vi "Lab Panel V3.0.vi"() -> ()   [LabVIEW 2013]
uses:
  <vilib>/Platform/TimedLoop/XDataNode/timing_clust.ctl
  <vilib>/Platform/TimedLoop/XDataNode/nitl_modes.ctl
  <vilib>/Platform/TimedLoop/XDataNode/wakeup.ctl
  <vilib>/platform/TimedLoop/XDataNode/XDataNode.xnode
  <vilib>/Platform/TimedLoop/XDataNode/XDNodeRunTimeDep.lvlib
panel:
  out "TEMP update":bool
  out "AI update":bool
  in  "stop":bool
  in  "Tab Control 2":T1(tab)
  out "LAB05-2 (SIG)":T2 {"PF" format="%.2f"; "AMPS" format="%.1f"}
  out "LAB05-1 (SIG)":T2 {"PF" format="%.2f"; "AMPS" format="%.1f"}
  out "LAB04-2 (SIG)":T2 {"PF" format="%.2f"; "AMPS" format="%.1f"}
  out "LAB04-1 (SIG)":T2 {"PF" format="%.2f"; "AMPS" format="%.1f"}
  out "LAB03-2 (SIG)":T2 {"PF" format="%.2f"; "AMPS" format="%.1f"}
  out "LAB03-1 (SIG)":T2 {"PF" format="%.2f"; "AMPS" format="%.1f"}
  out "LAB02-2 (SIG)":T2 {"PF" format="%.2f"; "AMPS" format="%.1f"}
  in  "LAB01-1RUN":bool
  in  "LAB05-1 (O/I)":bool
  in  "LAB05-2 (O/I)":bool
  in  "LAB04-1 (O/I)":bool
  in  "LAB04-2 (O/I)":bool
  in  "LAB02-1 (O/I)":bool
  in  "LAB02-2 (O/I)":bool
  in  "LAB01-2 (O/I)":bool
  in  "LAB01-1 (O/I)":bool
  in  "LAB03-1 (O/I)":bool
  in  "LAB05-2 RUN":bool
  in  "LAB05-1 RUN":bool
  in  "LAB04-2 RUN":bool
  in  "LAB04-1 RUN":bool
  in  "LAB03-2 RUN":bool
  in  "LAB03-1 RUN":bool
  in  "LAB02-2 RUN":bool
  in  "LAB02-1 RUN":bool
  in  "LAB01-2 RUN":bool
  in  "LAB05-2 SELECT":T3(radio)
  in  "LAB05-1 SELECT":T3(radio)
  in  "LAB04-2 SELECT":T3(radio)
  in  "LAB04-1 SELECT":T3(radio)
  in  "LAB03-2 SELECT":T3(radio)
  in  "LAB03-1 SELECT":T3(radio)
  in  "LAB02-2 SELECT":T3(radio)
  in  "LAB02-1 SELECT":T3(radio)
  in  "LAB01-2 SELECT":T3(radio)
  in  "LAB01-1 SELECT":T3(radio)
  in  "LAB03-2 (O/I)":bool
  out "LAB01-1 (SIG)":T2 {"PF" format="%.2f"; "AMPS" format="%.1f"}
  out "LAB01-2 (SIG)":T2 {"PF" format="%.2f"; "AMPS" format="%.1f"}
  out "LAB02-1 (SIG)":T2 {"PF" format="%.2f"; "AMPS" format="%.1f"}
  out "LAB05-2 (DISP)":T4 {"MINS" format="%.2g"}
  out "LAB05-1 (DISP)":T4 {"MINS" format="%.2g"}
  out "LAB04-2 (DISP)":T4 {"MINS" format="%.2g"}
  out "LAB04-1 (DISP)":T4 {"MINS" format="%.2g"}
  out "LAB03-2 (DISP)":T4 {"MINS" format="%.2g"}
  out "LAB03-1 (DISP)":T4 {"MINS" format="%.2g"}
  in  "LAB05-2 (SET)":T5
  in  "LAB05-1 (SET)":T5
  in  "LAB04-2 (SET)":T5
  in  "LAB04-1 (SET)":T5
  in  "LAB03-2 (SET)":T5
  in  "LAB03-1 (SET)":T5
  out "LAB02-2 (DISP)":T4 {"MINS" format="%.2g"}
  out "LAB02-1 (DISP)":T4 {"MINS" format="%.2g"}
  in  "LAB02-2 (SET)":T5
  in  "LAB02-1 (SET)":T5
  out "LAB05-2 (RESULT)":bool
  out "LAB05-1 (RESULT)":bool
  out "LAB04-2 (RESULT)":bool
  out "LAB04-1 (RESULT)":bool
  out "LAB03-2 (RESULT)":bool
  out "LAB03-1 (RESULT)":bool
  out "LAB02-2 (RESULT)":bool
  out "LAB02-1 (RESULT)":bool
  out "LAB01-2 (RESULT)":bool
  out "LAB01-1 (RESULT)":bool
  in  "LAB01-1 (SET)":T5
  in  "LAB01-2 (SET)":T5
  out "LAB01-1 (DISP)":T4 {"MINS" format="%.2g"}
  out "LAB01-2 (DISP)":T4 {"MINS" format="%.2f"}
  in  "Network Directory":path
  in  "JIG OFF TIME (S)":dbl=2.0 min=2.0 max=10.0 step=0.5 format="%.1g"
  in  "JIG ON TIME (S)":dbl=1.0 min=1.0 max=10.0 step=0.5 format="%.1g"
  out "LAB05-2 (FAIL)":cluster{"LO":dbl, "HI":dbl}
  out "LAB05-1 (FAIL)":cluster{"LO":dbl, "HI":dbl}
  out "LAB04-2 (FAIL)":cluster{"LO":dbl, "HI":dbl}
  out "LAB04-1 (FAIL)":cluster{"LO":dbl, "HI":dbl}
  out "LAB03-2 (FAIL)":cluster{"LO":dbl, "HI":dbl}
  out "LAB03-1 (FAIL)":cluster{"LO":dbl, "HI":dbl}
  out "LAB02-2 (FAIL)":cluster{"LO":dbl, "HI":dbl}
  out "LAB02-1 (FAIL)":cluster{"LO":dbl, "HI":dbl}
  out "LAB01-2 (FAIL)":cluster{"LO":dbl, "HI":dbl}
  out "LAB01-1 (FAIL)":cluster{"LO":dbl, "HI":dbl}
  out "LAB05-2 (TEMP START)":cluster{"TL":dbl, "TN":dbl}
  out "LAB04-2 (TEMP START)":cluster{"TL":dbl, "TN":dbl}
  out "LAB03-2 (TEMP START)":cluster{"TL":dbl, "TN":dbl}
  out "LAB02-2 (TEMP START)":cluster{"TL":dbl, "TN":dbl}
  out "LAB01-2 (TEMP START)":cluster{"TL":dbl, "TN":dbl}
  out "LAB05-1 (TEMP START)":cluster{"TL":dbl, "TN":dbl}
  out "LAB04-1 (TEMP START)":cluster{"TL":dbl, "TN":dbl}
  out "LAB03-1 (TEMP START)":cluster{"TL":dbl, "TN":dbl}
  out "LAB02-1 (TEMP START)":cluster{"TL":dbl, "TN":dbl}
  out "LAB01-1 (TEMP START)":cluster{"TL":dbl, "TN":dbl}
  out "LAB01-1 (JIG)":bool
  out "LAB01-2 (JIG)":bool
  out "LAB02-1 (JIG)":bool
  out "LAB02-2 (JIG)":bool
  out "LAB03-1 (JIG)":bool
  out "LAB03-2 (JIG)":bool
  out "LAB04-1 (JIG)":bool
  out "LAB04-2 (JIG)":bool
  out "LAB05-1 (JIG)":bool
  out "LAB05-2 (JIG)":bool
  out "LAB01 (CAL)":T6 {"2 (TN) cal" min=0.0 step=0.01 format="%.2f"; "2 (TL) cal" min=0.0 step=0.01 format="%.2f"; "2 (PF) cal" min=0.0 step=0.01 format="%.2f"; "2 (V) cal" min=0.0 step=0.01 format="%.2f"; "2 (A) cal" min=0.0 step=0.01 format="%.2f"; "1 (TN) cal" min=0.0 step=0.01 format="%.2f"; "1 (TL) cal" min=0.0 step=0.01 format="%.2f"; "1 (PF) cal" min=0.0 step=0.01 format="%.2f"; "1 (V) cal" min=0.0 step=0.01 format="%.2f"; "1  (A) cal" min=0.0 step=0.01 format="%.2f"}
  out "LAB03 (CAL)":T6 {"2 (TN) cal" min=0.0 step=0.01 format="%.2f"; "2 (TL) cal" min=0.0 step=0.01 format="%.2f"; "2 (PF) cal" min=0.0 step=0.01 format="%.2f"; "2 (V) cal" min=0.0 step=0.01 format="%.2f"; "2 (A) cal" min=0.0 step=0.01 format="%.2f"; "1 (TN) cal" min=0.0 step=0.01 format="%.2f"; "1 (TL) cal" min=0.0 step=0.01 format="%.2f"; "1 (PF) cal" min=0.0 step=0.01 format="%.2f"; "1 (V) cal" min=0.0 step=0.01 format="%.2f"; "1  (A) cal" min=0.0 step=0.01 format="%.2f"}
  out "LAB02 (CAL)":T7 {"2 (TN) cal" min=0.0 step=0.01 format="%.2f"; "2 (TL) cal" min=0.0 step=0.01 format="%.2f"; "2 (PF) cal" min=0.0 step=0.01 format="%.2f"; "2 (V) cal" min=0.0 step=0.01 format="%.2f"; "2 (A) cal" min=0.0 step=0.01 format="%.2f"; "1 (TN) cal" min=0.0 step=0.01 format="%.2f"; "1 (TL) cal" min=0.0 step=0.01 format="%.2f"; "1 (PF) cal" min=0.0 step=0.01 format="%.2f"; "1 (V) cal" min=0.0 step=0.01 format="%.2f"; "1 (A) cal" min=0.0 step=0.01 format="%.2f"}
  out "LAB05 (CAL)":T6 {"2 (TN) cal" min=0.0 step=0.01 format="%.2f"; "2 (TL) cal" min=0.0 step=0.01 format="%.2f"; "2 (PF) cal" min=0.0 step=0.01 format="%.2f"; "2 (V) cal" min=0.0 step=0.01 format="%.2f"; "2 (A) cal" min=0.0 step=0.01 format="%.2f"; "1 (TN) cal" min=0.0 step=0.01 format="%.2f"; "1 (TL) cal" min=0.0 step=0.01 format="%.2f"; "1 (PF) cal" min=0.0 step=0.01 format="%.2f"; "1 (V) cal" min=0.0 step=0.01 format="%.2f"; "1  (A) cal" min=0.0 step=0.01 format="%.2f"}
  out "LAB04 (CAL)":T6 {"2 (TN) cal" min=0.0 step=0.01 format="%.2f"; "2 (TL) cal" min=0.0 step=0.01 format="%.2f"; "2 (PF) cal" min=0.0 step=0.01 format="%.2f"; "2 (V) cal" min=0.0 step=0.01 format="%.2f"; "2 (A) cal" min=0.0 step=0.01 format="%.2f"; "1 (TN) cal" min=0.0 step=0.01 format="%.2f"; "1 (TL) cal" min=0.0 step=0.01 format="%.2f"; "1 (PF) cal" min=0.0 step=0.01 format="%.2f"; "1 (V) cal" min=0.0 step=0.01 format="%.2f"; "1  (A) cal" min=0.0 step=0.01 format="%.2f"}
  out "calibration file error out":errorcluster
  in  "CALIBRATE":bool
  in  "Tab Control":T8(tab)
  out "LAB01-2 (GRAPH)":dynamicdata(graph)
  out "LAB01-1 (GRAPH)":dynamicdata(graph)
  out "LAB02-2 (GRAPH)":dynamicdata(graph)
  out "LAB02-1 (GRAPH)":dynamicdata(graph)
  out "LAB03-2 (GRAPH)":dynamicdata(graph)
  out "LAB03-1 (GRAPH)":dynamicdata(graph)
  out "LAB04-2 (GRAPH)":dynamicdata(graph)
  out "LAB04-1 (GRAPH)":dynamicdata(graph)
  out "LAB05-2 (GRAPH)":dynamicdata(graph)
  out "LAB05-1 (GRAPH)":dynamicdata(graph)
  out "LAB05 TEMP":T9
  out "LAB04 TEMP":T9
  out "LAB02 TEMP":T9
  out "LAB01 TEMP":T9
  out "LAB03 TEMP":T9
  out "Analog Error Array":errorcluster[](array[cluster])
  out "AI loop time":dbl format="%.6g"
  out "loops":dbl
  in  "loop  delay(mS)":dbl
  out "on loops":dbl
  out "off loops":dbl
  out "jig cycle":dbl
  out "LAB01-1 (TDMS)":refnum<k34>
  out "data file error":errorcluster
  out "LAB02-1 (TDMS)":refnum<k34>
  out "LAB01-2 (TDMS)":refnum<k34>
  out "LAB02-2 (TDMS)":refnum<k34>
  out "LAB03-1 (TDMS)":refnum<k34>
  out "LAB03-2 (TDMS)":refnum<k34>
  out "LAB04-1 (TDMS)":refnum<k34>
  out "LAB04-2 (TDMS)":refnum<k34>
  out "LAB05-1 (TDMS)":refnum<k34>
  out "LAB05-2 (TDMS)":refnum<k34>
  # "LAB01"
  # "LAB02"
  # "LAB05"
  # "LAB03"
  # "LAB04"
  # "LAB01"
  # "LAB02"
  # "LAB03"
  # "LAB04"
  # "LAB05"
  # "JIG SET"
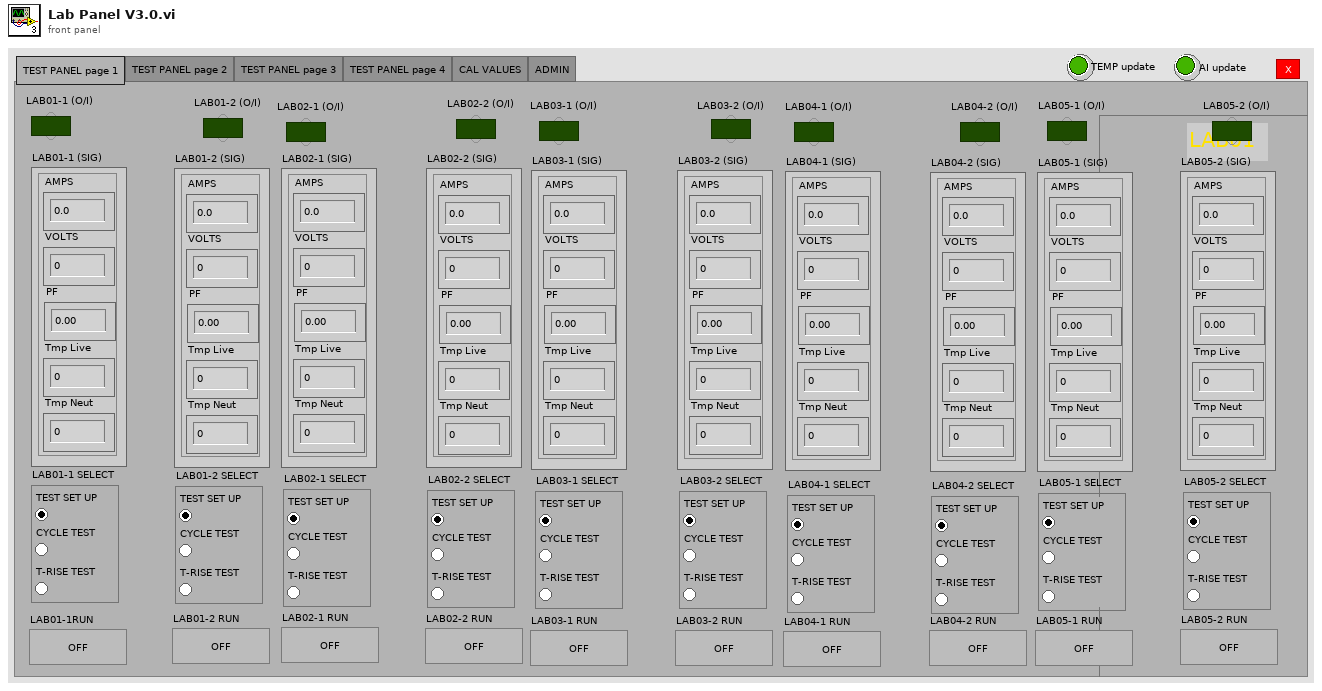
[diagram p1: front panel]
types:
  T1 = enum32{"TEST PANEL page 1", "TEST PANEL page 2", "TEST PANEL page 3", "TEST PANEL page 4", "CAL VALUES", "ADMIN"}
  T2 = cluster{"AMPS":dbl, "VOLTS":dbl, "PF":dbl, "Tmp Live":dbl, "Tmp Neut":dbl}
  T3 = enum32{"TEST SET UP", "CYCLE TEST", "T-RISE TEST"}
  T4 = cluster{"CYCLE":dbl, "MINS":dbl, "STATUS":string}
  T5 = cluster{"NAME":string, "DESCRIPTION":string, "CYCLES":dbl, "T-RISE mins":dbl, "T-RISE deg C":dbl}
  T6 = cluster{"1  (A) cal":dbl, "1 (V) cal":dbl, "1 (PF) cal":dbl, "1 (TL) cal":dbl, "1 (TN) cal":dbl, "2 (A) cal":dbl, "2 (V) cal":dbl, "2 (PF) cal":dbl, "2 (TL) cal":dbl, "2 (TN) cal":dbl}
  T7 = cluster{"1 (A) cal":dbl, "1 (V) cal":dbl, "1 (PF) cal":dbl, "1 (TL) cal":dbl, "1 (TN) cal":dbl, "2 (A) cal":dbl, "2 (V) cal":dbl, "2 (PF) cal":dbl, "2 (TL) cal":dbl, "2 (TN) cal":dbl}
  T8 = enum32{"LAB01", "LAB02", "LAB03", "LAB04", "LAB05", "TEMPERATURE", "ERROR"}
  T9 = cluster{"T1 Live":dbl, "T1 Neut":dbl, "T2 Live":dbl, "T2 Neut":dbl, "ID":dbl, "ER":dbl}
  T10 = enum8{"Enabled", "Disabled", "Disabled and Grayed Out"}
  T11 = typedef "XDNodeRunTimeDep.lvlib/timing_clust.ctl" = cluster{"Expected End [f-1]":u64, "Actual End [f-1]":u64, "Finished Late? [f-1]":bool, "Expected End [i-1]":u64, "Actual End [i-1]":u64, "Finished Late? [i-1]":bool, "Expected Start [i]":u64, "Actual Start [i]":u64, "Expected Start [f]":u64, "Actual Start [f]":u64, "Source Name":string, "Structure Name":string, "Period":i64, "Deadline":i64, "Offset":i64, "Start":i64, "Priority":i32, "Timeout":i32, "Mode":T12, "Wakeup Reason":T13, "Error":errorcluster, "Source Type":string, "Secondary Source Type":string, "Global End Time":u64, "Global Start Time":u64, "Frame Duration":u64, "Iteration Duration":u64, "Assigned CPU":i32, "I/O Scan Engine Mode":u32}
  T12 = typedef "XDNodeRunTimeDep.lvlib/nitl_modes.ctl" = enum32{"No Change", "Process missed periods, maintain original phase", "Discard missed periods, maintain original phase", "Process missed periods, ignore original phase", "Discard missed periods, ignore original phase"}
  T13 = typedef "XDNodeRunTimeDep.lvlib/wakeup.ctl" = enum32{"Normal", "Aborted", "Asynchronous wakeup", "Timing source error", "Timed loop error", "Timeout"}
  T14 = enum16{"open", "open or create", "create or replace", "create", "open (read-only)"}
  T15 = enum16{"open", "replace", "create", "open or create", "replace or create", "replace or create with confirmation"}
  T16 = cluster{"LAB01-1 (SET)":cluster{"NAME":string, "DESCRIPTION":string, "CYCLES":dbl, "T-RISE mins":dbl, "T-RISE deg C":dbl}, "LAB01-2 (SET)":cluster{"NAME":string, "DESCRIPTION":string, "CYCLES":dbl, "T-RISE mins":dbl, "T-RISE deg C":dbl}, "LAB02-1 (SET)":cluster{"NAME":string, "DESCRIPTION":string, "CYCLES":dbl, "T-RISE mins":dbl, "T-RISE deg C":dbl}, "LAB02-2 (SET)":cluster{"NAME":string, "DESCRIPTION":string, "CYCLES":dbl, "T-RISE mins":dbl, "T-RISE deg C":dbl}, "LAB03-1 (SET)":cluster{"NAME":string, "DESCRIPTION":string, "CYCLES":dbl, "T-RISE mins":dbl, "T-RISE deg C":dbl}, "LAB03-2 (SET)":cluster{"NAME":string, "DESCRIPTION":string, "CYCLES":dbl, "T-RISE mins":dbl, "T-RISE deg C":dbl}, "LAB04-1 (SET)":cluster{"NAME":string, "DESCRIPTION":string, "CYCLES":dbl, "T-RISE mins":dbl, "T-RISE deg C":dbl}, "LAB04-2 (SET)":cluster{"NAME":string, "DESCRIPTION":string, "CYCLES":dbl, "T-RISE mins":dbl, "T-RISE deg C":dbl}, "LAB05-1 (SET)":cluster{"NAME":string, "DESCRIPTION":string, "CYCLES":dbl, "T-RISE mins":dbl, "T-RISE deg C":dbl}, "LAB05-2 (SET)":cluster{"NAME":string, "DESCRIPTION":string, "CYCLES":dbl, "T-RISE mins":dbl, "T-RISE deg C":dbl}, "Network Directory":path}
  T17 = cluster{"T1":dbl, "T2":dbl, "T3":dbl, "T4":dbl, "ID":dbl, "ER":dbl}
  T18 = cluster{"LAB01-1 (A)":dbl, "LAB01-1 (V)":dbl, "LAB01-1 (PF)":dbl, "LAB01-2 (A)":dbl, "LAB01-2 (V)":dbl, "LAB01-2 (PF)":dbl}
  T19 = cluster{"LAB02-1 (A)":dbl, "LAB02-1 (V)":dbl, "LAB02-1 (PF)":dbl, "LAB02-2 (A)":dbl, "LAB02-2 (V)":dbl, "LAB02-2 (PF)":dbl}
  T20 = cluster{"LAB03-1 (A)":dbl, "LAB03-1 (V)":dbl, "LAB03-1 (PF)":dbl, "LAB03-2 (A)":dbl, "LAB03-2 (V)":dbl, "LAB03-2 (PF)":dbl}
  T21 = cluster{"LAB04-1 (A)":dbl, "LAB04-1 (V)":dbl, "LAB04-1 (PF)":dbl, "LAB04-2 (A)":dbl, "LAB04-2 (V)":dbl, "LAB04-2 (PF)":dbl}
  T22 = cluster{"LAB05-1 (A)":dbl, "LAB05-1 (V)":dbl, "LAB05-1 (PF)":dbl, "LAB05-2 (A)":dbl, "LAB05-2 (V)":dbl, "LAB05-2 (PF)":dbl}
  T23 = cluster{"LAB01-1 (FAIL)":cluster{"LO":dbl, "HI":dbl}, "LAB01-1 (SIG)":cluster{"AMPS":dbl, "VOLTS":dbl, "PF":dbl, "Tmp Live":dbl, "Tmp Neut":dbl}, "LAB01-1 (TEMP START)":cluster{"TL":dbl, "TN":dbl}, "LAB01-1 (DISP)":cluster{"CYCLE":dbl, "MINS":dbl, "STATUS":string}, "LAB01-1 (SET)":cluster{"NAME":string, "DESCRIPTION":string, "CYCLES":dbl, "T-RISE mins":dbl, "T-RISE deg C":dbl}, "LAB01-1 (TDMS)":refnum<k34>}
  T24 = cluster{"LAB01-2 (FAIL)":cluster{"LO":dbl, "HI":dbl}, "LAB01-2 (SIG)":cluster{"AMPS":dbl, "VOLTS":dbl, "PF":dbl, "Tmp Live":dbl, "Tmp Neut":dbl}, "LAB01-2 (TEMP START)":cluster{"TL":dbl, "TN":dbl}, "LAB01-2 (DISP)":cluster{"CYCLE":dbl, "MINS":dbl, "STATUS":string}, "LAB01-2 (SET)":cluster{"NAME":string, "DESCRIPTION":string, "CYCLES":dbl, "T-RISE mins":dbl, "T-RISE deg C":dbl}, "LAB01-2 (TDMS)":refnum<k34>}
  T25 = cluster{"LAB02-1 (FAIL)":cluster{"LO":dbl, "HI":dbl}, "LAB02-1 (SIG)":cluster{"AMPS":dbl, "VOLTS":dbl, "PF":dbl, "Tmp Live":dbl, "Tmp Neut":dbl}, "LAB02-1 (TEMP START)":cluster{"TL":dbl, "TN":dbl}, "LAB02-1 (DISP)":cluster{"CYCLE":dbl, "MINS":dbl, "STATUS":string}, "LAB02-1 (SET)":cluster{"NAME":string, "DESCRIPTION":string, "CYCLES":dbl, "T-RISE mins":dbl, "T-RISE deg C":dbl}, "LAB02-1 (TDMS)":refnum<k34>}
  T26 = cluster{"LAB02-2 (FAIL)":cluster{"LO":dbl, "HI":dbl}, "LAB02-2 (SIG)":cluster{"AMPS":dbl, "VOLTS":dbl, "PF":dbl, "Tmp Live":dbl, "Tmp Neut":dbl}, "LAB02-2 (TEMP START)":cluster{"TL":dbl, "TN":dbl}, "LAB02-2 (DISP)":cluster{"CYCLE":dbl, "MINS":dbl, "STATUS":string}, "LAB02-2 (SET)":cluster{"NAME":string, "DESCRIPTION":string, "CYCLES":dbl, "T-RISE mins":dbl, "T-RISE deg C":dbl}, "LAB02-2 (TDMS)":refnum<k34>}
  T27 = cluster{"LAB03-1 (FAIL)":cluster{"LO":dbl, "HI":dbl}, "LAB03-1 (SIG)":cluster{"AMPS":dbl, "VOLTS":dbl, "PF":dbl, "Tmp Live":dbl, "Tmp Neut":dbl}, "LAB03-1 (TEMP START)":cluster{"TL":dbl, "TN":dbl}, "LAB03-1 (DISP)":cluster{"CYCLE":dbl, "MINS":dbl, "STATUS":string}, "LAB03-1 (SET)":cluster{"NAME":string, "DESCRIPTION":string, "CYCLES":dbl, "T-RISE mins":dbl, "T-RISE deg C":dbl}, "LAB03-1 (TDMS)":refnum<k34>}
  T28 = cluster{"LAB03-2 (FAIL)":cluster{"LO":dbl, "HI":dbl}, "LAB03-2 (SIG)":cluster{"AMPS":dbl, "VOLTS":dbl, "PF":dbl, "Tmp Live":dbl, "Tmp Neut":dbl}, "LAB03-2 (TEMP START)":cluster{"TL":dbl, "TN":dbl}, "LAB03-2 (DISP)":cluster{"CYCLE":dbl, "MINS":dbl, "STATUS":string}, "LAB03-2 (SET)":cluster{"NAME":string, "DESCRIPTION":string, "CYCLES":dbl, "T-RISE mins":dbl, "T-RISE deg C":dbl}, "LAB03-2 (TDMS)":refnum<k34>}
  T29 = cluster{"LAB04-1 (FAIL)":cluster{"LO":dbl, "HI":dbl}, "LAB04-1 (SIG)":cluster{"AMPS":dbl, "VOLTS":dbl, "PF":dbl, "Tmp Live":dbl, "Tmp Neut":dbl}, "LAB04-1 (TEMP START)":cluster{"TL":dbl, "TN":dbl}, "LAB04-1 (DISP)":cluster{"CYCLE":dbl, "MINS":dbl, "STATUS":string}, "LAB04-1 (SET)":cluster{"NAME":string, "DESCRIPTION":string, "CYCLES":dbl, "T-RISE mins":dbl, "T-RISE deg C":dbl}, "LAB04-1 (TDMS)":refnum<k34>}
  T30 = cluster{"LAB04-2 (FAIL)":cluster{"LO":dbl, "HI":dbl}, "LAB04-2 (SIG)":cluster{"AMPS":dbl, "VOLTS":dbl, "PF":dbl, "Tmp Live":dbl, "Tmp Neut":dbl}, "LAB04-2 (TEMP START)":cluster{"TL":dbl, "TN":dbl}, "LAB04-2 (DISP)":cluster{"CYCLE":dbl, "MINS":dbl, "STATUS":string}, "LAB04-2 (SET)":cluster{"NAME":string, "DESCRIPTION":string, "CYCLES":dbl, "T-RISE mins":dbl, "T-RISE deg C":dbl}, "LAB04-2 (TDMS)":refnum<k34>}
  T31 = cluster{"LAB05-1 (FAIL)":cluster{"LO":dbl, "HI":dbl}, "LAB05-1 (SIG)":cluster{"AMPS":dbl, "VOLTS":dbl, "PF":dbl, "Tmp Live":dbl, "Tmp Neut":dbl}, "LAB05-1 (TEMP START)":cluster{"TL":dbl, "TN":dbl}, "LAB05-1 (DISP)":cluster{"CYCLE":dbl, "MINS":dbl, "STATUS":string}, "LAB05-1 (SET)":cluster{"NAME":string, "DESCRIPTION":string, "CYCLES":dbl, "T-RISE mins":dbl, "T-RISE deg C":dbl}, "LAB05-1 (TDMS)":refnum<k34>}
  T32 = cluster{"LAB05-2 (FAIL)":cluster{"LO":dbl, "HI":dbl}, "LAB05-2 (SIG)":cluster{"AMPS":dbl, "VOLTS":dbl, "PF":dbl, "Tmp Live":dbl, "Tmp Neut":dbl}, "LAB05-2 (TEMP START)":cluster{"TL":dbl, "TN":dbl}, "LAB05-2 (DISP)":cluster{"CYCLE":dbl, "MINS":dbl, "STATUS":string}, "LAB05-2 (SET)":cluster{"NAME":string, "DESCRIPTION":string, "CYCLES":dbl, "T-RISE mins":dbl, "T-RISE deg C":dbl}, "LAB05-2 (TDMS)":refnum<k34>}
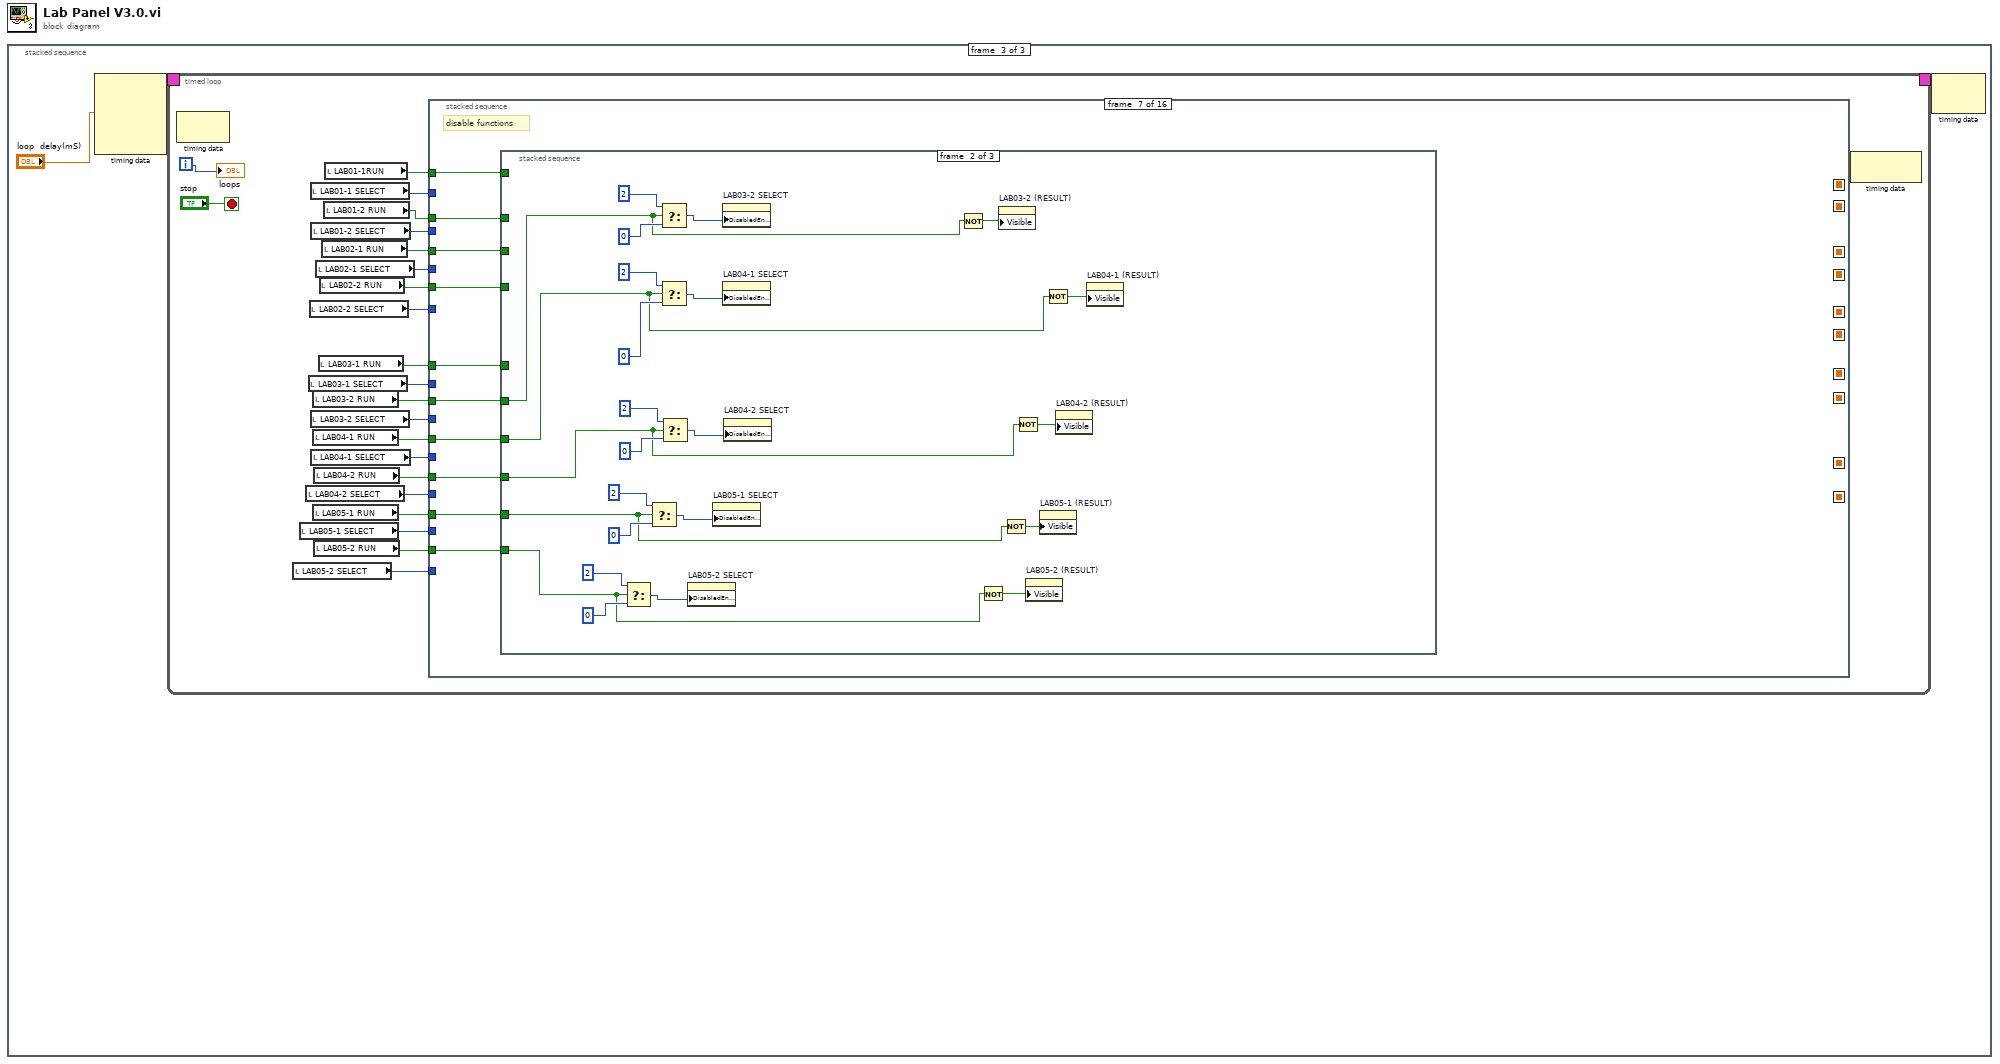
[diagram p0: block diagram]
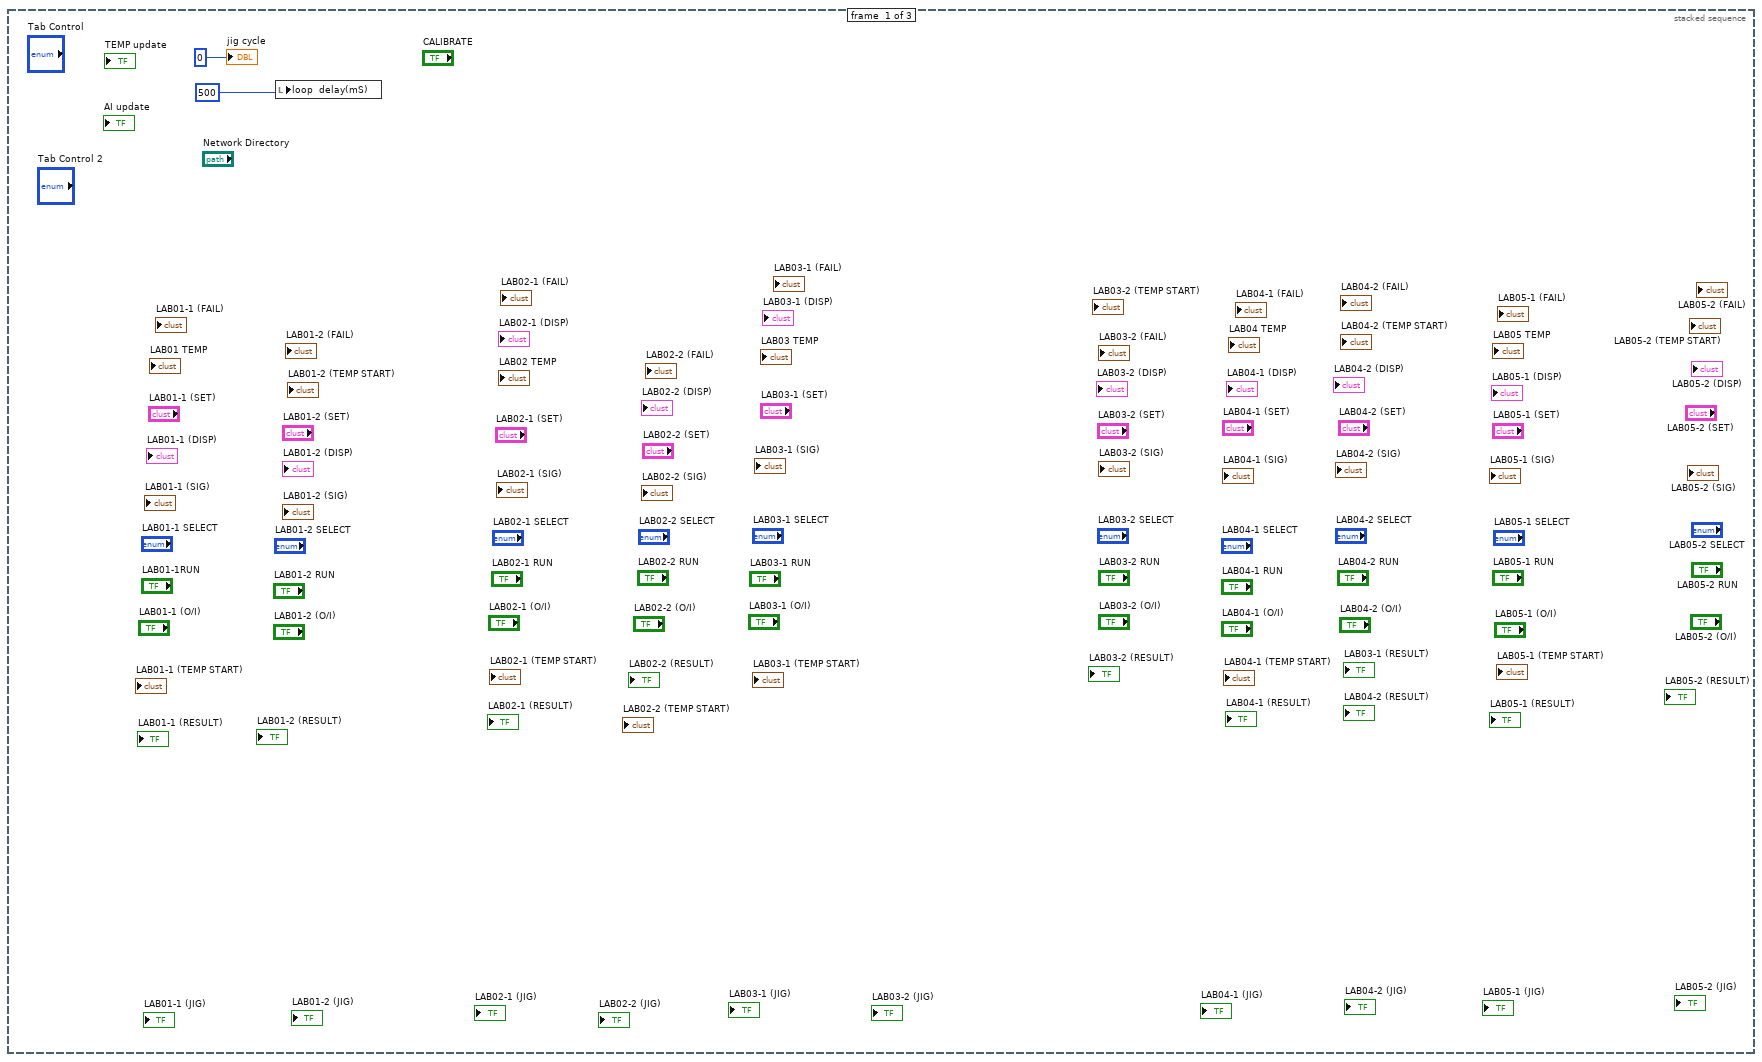
[diagram p2: hidden frame]
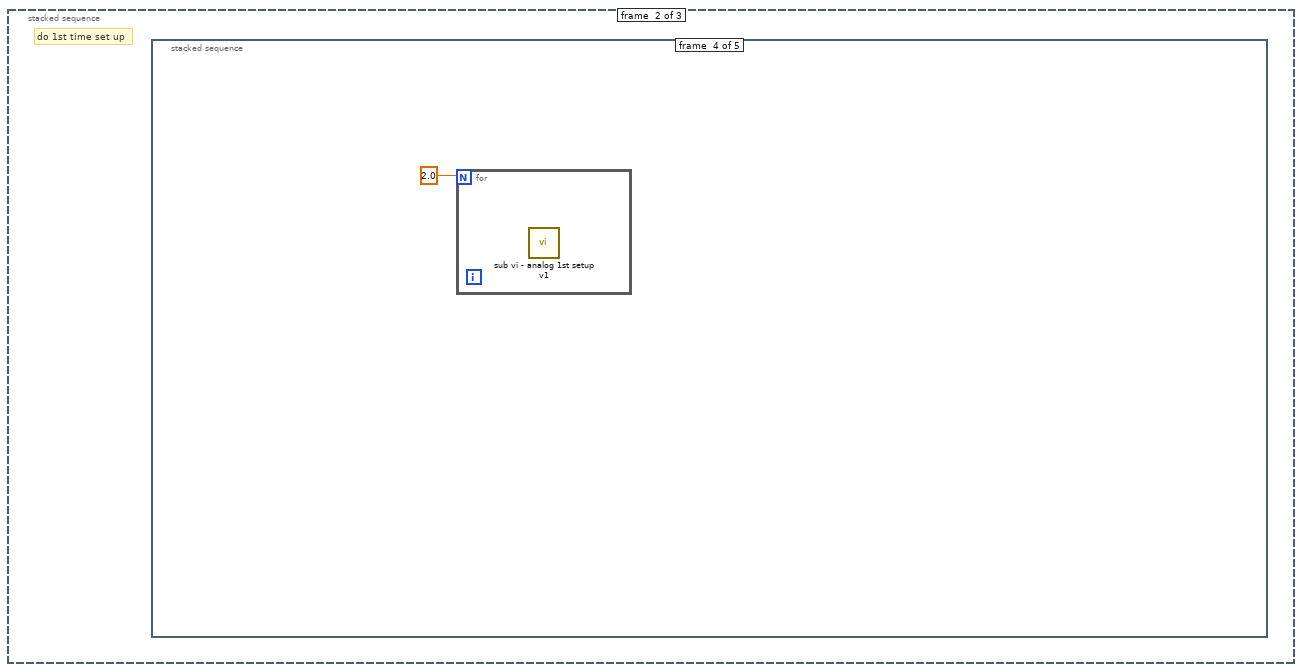
[diagram p3: hidden frame]
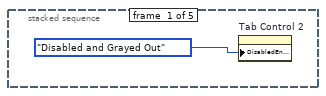
[diagram p4: hidden frame]
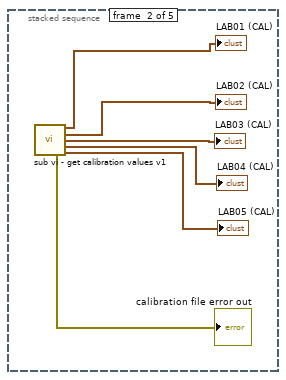
[diagram p5: hidden frame]
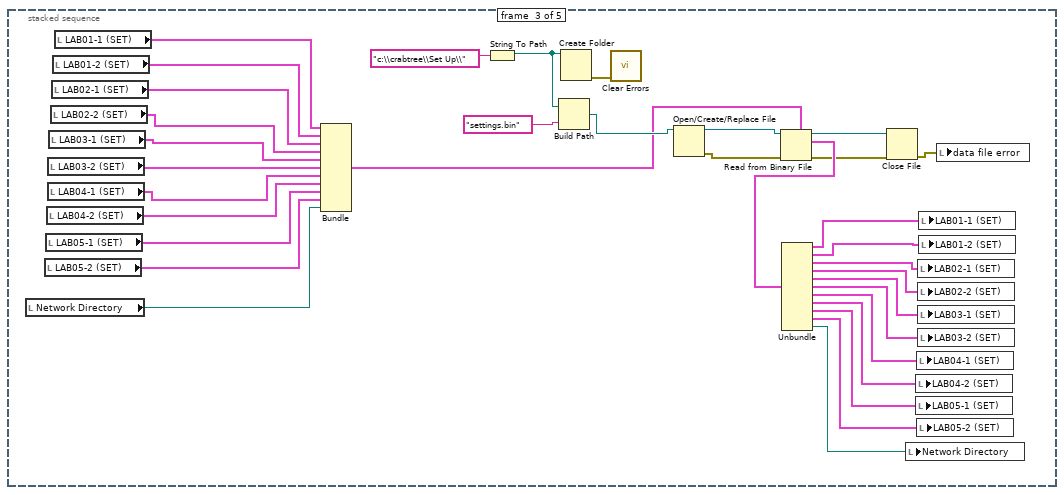
[diagram p6: hidden frame]
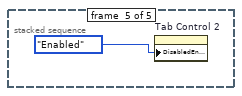
[diagram p7: hidden frame]
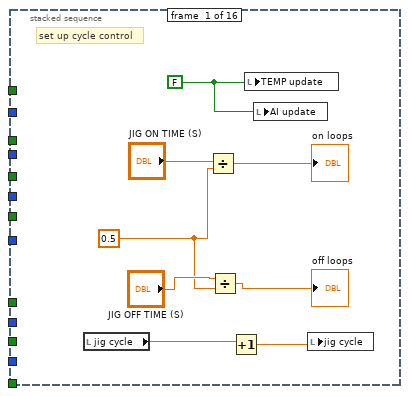
[diagram p8: hidden frame]
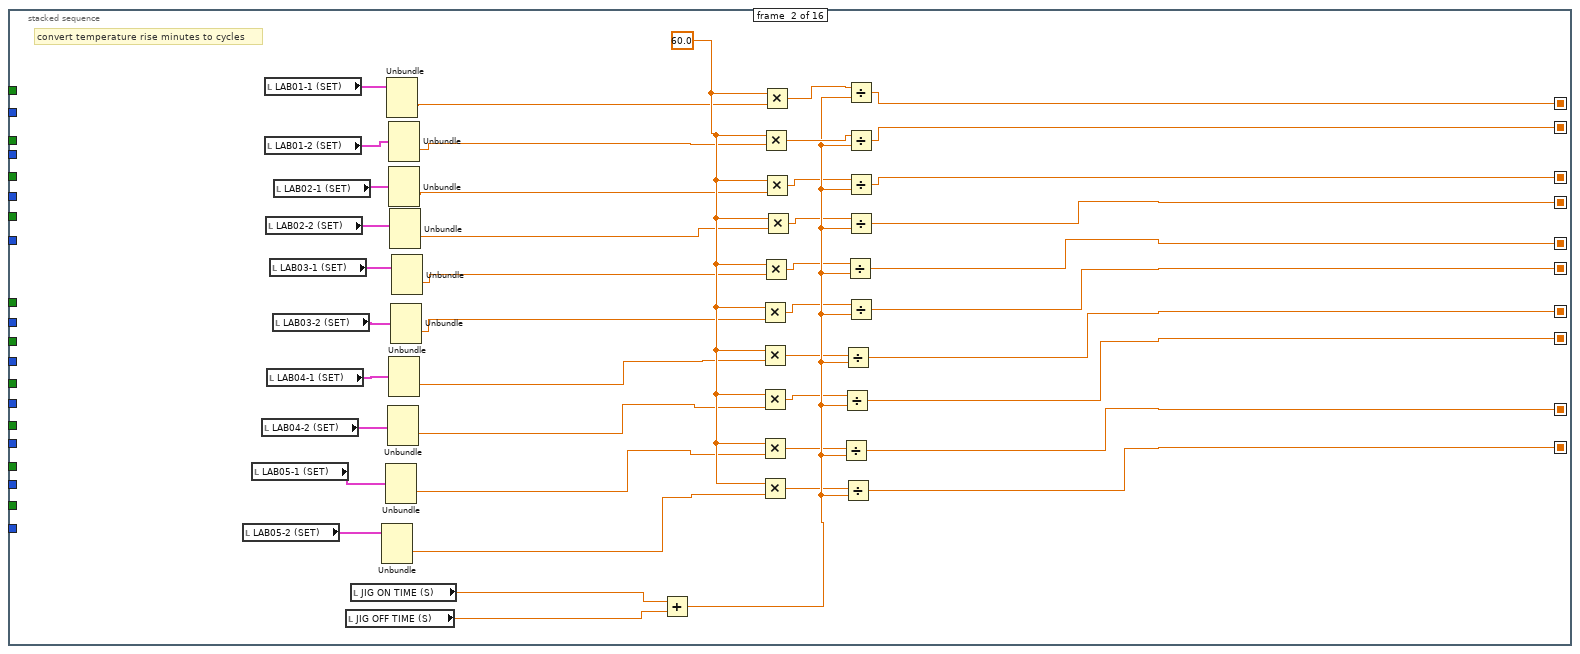
[diagram p9: hidden frame]
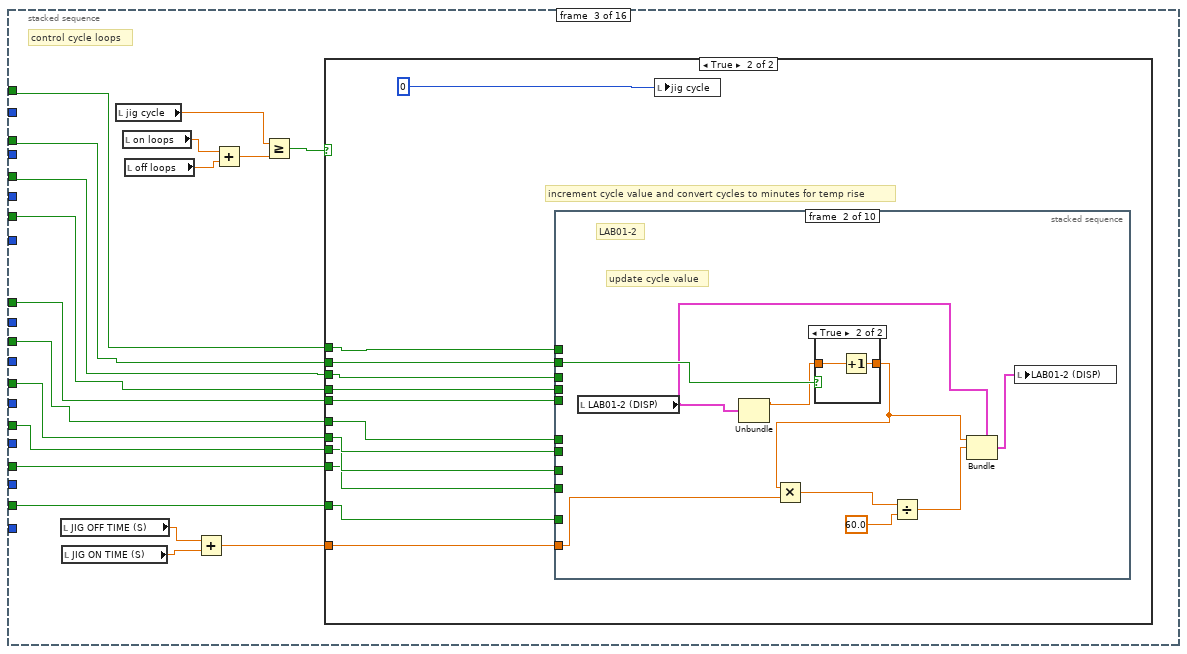
[diagram p10: hidden frame]
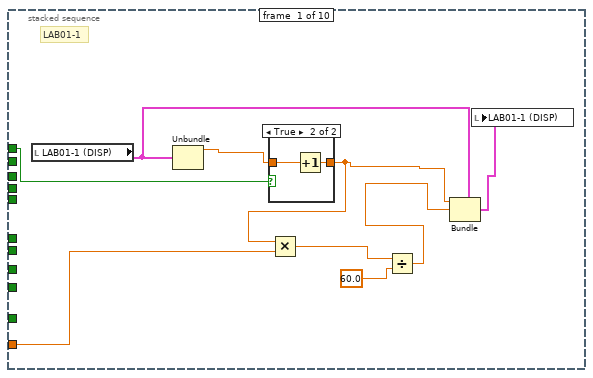
[diagram p12: hidden frame]
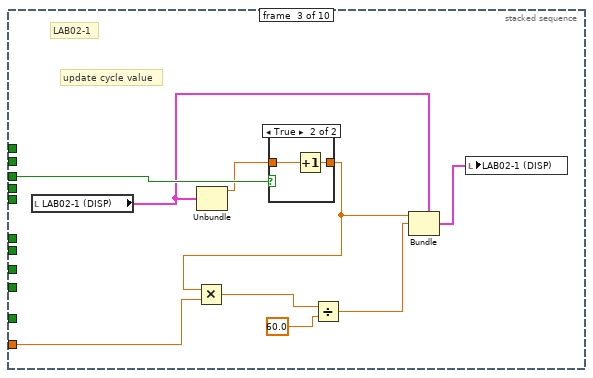
[diagram p15: hidden frame]
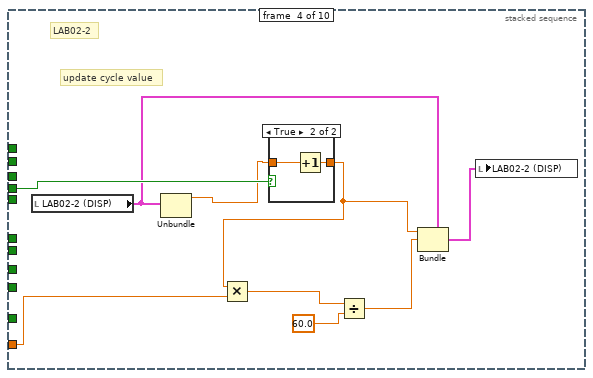
[diagram p17: hidden frame]
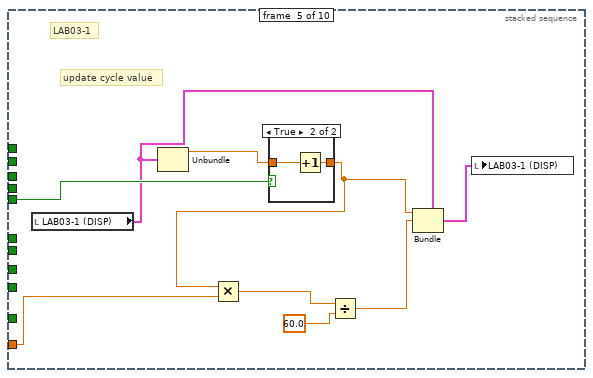
[diagram p19: hidden frame]
diagram:
  n1 = stacked-sequence {
    frame #0 {
      n2 = local write "loop  delay(mS)"(500) -> ()
      "jig cycle" <- 0
    }
    frame #1 {
      # "do 1st time set up"
      n3 = stacked-sequence {
        frame #0 {
          n4 = property on="Tab Control 2" class="TabCtl (strict)"("DisabledEnum"=T10."Disabled and Grayed Out" ("Disabled")) -> ()  [unwired: 2 in, 2 out]
        }
        frame #1 {
          n5 = call "sub vi - get calibration values v1.vi"() -> ("LAB01 (CAL)"=→"LAB01 (CAL)":T6, "LAB02 (CAL)"=→"LAB02 (CAL)":T7, "LAB03 (CAL)"=→"LAB03 (CAL)":T6, "LAB04 (CAL)"=→"LAB04 (CAL)":T6, "calibration file error out"=→"calibration file error out":errorcluster, "LAB05 (CAL)"=→"LAB05 (CAL)":T6)  [unwired: 10 in]
        }
        frame #2 {
          n6 = local read "Network Directory"() -> (w39:path)
          n7 = local read "LAB05-2 (SET)"() -> (w40:T5)
          n8 = local read "LAB05-1 (SET)"() -> (w41:T5)
          n9 = local read "LAB04-2 (SET)"() -> (w42:T5)
          n10 = local read "LAB03-2 (SET)"() -> (w38:T5)
          n11 = local read "LAB04-1 (SET)"() -> (w43:T5)
          n12 = local read "LAB03-1 (SET)"() -> (w37:T5)
          n13 = local read "LAB02-2 (SET)"() -> (w36:T5)
          n14 = local read "LAB02-1 (SET)"() -> (w35:T5)
          n15 = local read "LAB01-2 (SET)"() -> (w34:T5)
          n16 = local read "LAB01-1 (SET)"() -> (w33:T5)
          n17 = Bundle("LAB01-1 (SET)"=w33, "LAB01-2 (SET)"=w34, "LAB02-1 (SET)"=w35, "LAB02-2 (SET)"=w36, "LAB03-1 (SET)"=w37, "LAB03-2 (SET)"=w38, "LAB04-1 (SET)"=w43, "LAB04-2 (SET)"=w42, "LAB05-1 (SET)"=w41, "LAB05-2 (SET)"=w40, "Network Directory"=w39) -> (w26:T16)  [unwired: 1 in]
          n18 = String To Path(string="c:\\crabtree\\Set Up\\") -> (path=w30:path)
          n19 = Build Path(base path=w30, name or relative path="settings.bin") -> (appended path=w28:path)
          n20 = Create Folder(path (use dialog)=w30) -> (error out=w32:errorcluster)  [unwired: 2 in, 2 out]
          n21 = call <vilib>:"Clear Errors.vi"("error in (no error)"=w32) -> ()  [unwired: 6 in, 1 out]
          n22 = Open/Create/Replace File(file path (use dialog)=w28) -> (refnum out=w25:refnum<file>, error out=w27:errorcluster)  [unwired: 5 in, 1 out]
          n23 = Read from Binary File(5:w26, 8:w27, 11:w25) -> (0:w22:errorcluster, 2:w24:T16, 3:w23:refnum<file>)  [unwired: 3 in, 1 out]
          n24 = Unbundle(w24) -> ("LAB01-1 (SET)"=w20:T5, "LAB01-2 (SET)"=w19:T5, "LAB02-1 (SET)"=w18:T5, "LAB02-2 (SET)"=w17:T5, "LAB03-1 (SET)"=w16:T5, "LAB03-2 (SET)"=w15:T5, "LAB04-1 (SET)"=w14:T5, "LAB04-2 (SET)"=w13:T5, "LAB05-1 (SET)"=w12:T5, "LAB05-2 (SET)"=w11:T5, "Network Directory"=w10:path)
          n25 = Close File(refnum=w23, error in=w22) -> (error out=w21:errorcluster)  [unwired: 1 out]
          n26 = local write "Network Directory"(w10) -> ()
          n27 = local write "LAB04-2 (SET)"(w13) -> ()
          n28 = local write "LAB05-1 (SET)"(w12) -> ()
          n29 = local write "LAB04-1 (SET)"(w14) -> ()
          n30 = local write "LAB05-2 (SET)"(w11) -> ()
          n31 = local write "LAB02-1 (SET)"(w18) -> ()
          n32 = local write "LAB02-2 (SET)"(w17) -> ()
          n33 = local write "LAB03-1 (SET)"(w16) -> ()
          n34 = local write "LAB03-2 (SET)"(w15) -> ()
          n35 = local write "LAB01-1 (SET)"(w20) -> ()
          n36 = local write "LAB01-2 (SET)"(w19) -> ()
          n37 = local write "data file error"(w21) -> ()
        }
        frame #3 {
          n38 = for {
            N: 2.0 -> [_]
            n39 = call "sub vi - analog 1st setup v1.vi"() -> ()  [unwired: 11 in, 5 out]
          }
        }
        frame #4 {
          n40 = property on="Tab Control 2" class="TabCtl (strict)"("DisabledEnum"=T10."Enabled" ("Disabled")) -> ()  [unwired: 2 in, 2 out]
        }
      }
    }
    frame #2 {
      n41 = node-c288("loop  delay(mS)") -> (w48:T11)  [unwired: 3 in]
      n42 = timed-loop {
        timing: w48 -> [_]
        timing-out: [_] -> w47
        i -> [w70]
        stop <- "stop" stop-if-true
        n43 = node-c288() -> ()  [unwired: 1 in, 1 out]
        n44 = local read "LAB05-2 SELECT"() -> (w49:T3)
        n45 = local read "LAB05-1 SELECT"() -> (w50:T3)
        n46 = local read "LAB04-2 SELECT"() -> (w51:T3)
        n47 = local read "LAB03-1 SELECT"() -> (w54:T3)
        n48 = local read "LAB02-2 SELECT"() -> (w55:T3)
        n49 = local read "LAB01-1 SELECT"() -> (w58:T3)
        n50 = local read "LAB03-2 SELECT"() -> (w53:T3)
        n51 = local read "LAB01-2 SELECT"() -> (w57:T3)
        n52 = local read "LAB04-1 SELECT"() -> (w52:T3)
        n53 = local read "LAB03-2 RUN"() -> (w63:bool)
        n54 = local read "LAB04-1 RUN"() -> (w62:bool)
        n55 = local read "LAB05-1 RUN"() -> (w60:bool)
        n56 = local read "LAB04-2 RUN"() -> (w61:bool)
        n57 = local read "LAB05-2 RUN"() -> (w59:bool)
        n58 = local read "LAB02-1 SELECT"() -> (w56:T3)
        n59 = local read "LAB03-1 RUN"() -> (w64:bool)
        n60 = local read "LAB02-2 RUN"() -> (w65:bool)
        n61 = local read "LAB02-1 RUN"() -> (w66:bool)
        n62 = local read "LAB01-2 RUN"() -> (w67:bool)
        n63 = local read "LAB01-1RUN"() -> (w68:bool)
        n64 = stacked-sequence {
          seq-local: [_ w122 _ _ _ _ _ _ _ _ _ _ _ _ _ _] -> [_ _ _ _ _ w1501 _ _ _ _ _ _ _ _ _ _]
          seq-local: [_ w121 _ _ _ _ _ _ _ _ _ _ _ _ _ _] -> [_ _ _ _ _ _ _ _ _ _ _ _ _ _ _ _]
          seq-local: [_ w108 _ _ _ _ _ _ _ _ _ _ _ _ _ _] -> [_ _ _ _ _ _ _ _ _ _ _ _ _ _ _ _]
          seq-local: [_ w107 _ _ _ _ _ _ _ _ _ _ _ _ _ _] -> [_ _ _ _ _ _ _ _ _ _ _ _ _ _ _ _]
          seq-local: [_ w106 _ _ _ _ _ _ _ _ _ _ _ _ _ _] -> [_ _ _ _ _ _ _ _ _ _ _ _ _ _ _ _]
          seq-local: [_ w105 _ _ _ _ _ _ _ _ _ _ _ _ _ _] -> [_ _ _ _ _ _ _ _ _ _ _ _ _ _ _ _]
          seq-local: [_ w104 _ _ _ _ _ _ _ _ _ _ _ _ _ _] -> [_ _ _ _ _ _ _ _ _ _ _ _ _ _ _ _]
          seq-local: [_ w103 _ _ _ _ _ _ _ _ _ _ _ _ _ _] -> [_ _ _ _ _ _ _ _ _ _ _ _ _ _ _ _]
          seq-local: [_ w102 _ _ _ _ _ _ _ _ _ _ _ _ _ _] -> [_ _ _ _ _ _ _ _ _ _ _ _ _ _ _ _]
          seq-local: [_ w101 _ _ _ _ _ _ _ _ _ _ _ _ _ _] -> [_ _ _ _ _ _ _ _ _ _ _ _ _ _ _ _]
          tunnel: w68 -> [_ _ w138 w294 w1101 w1512 w1822 w1903 _ _ _ _ w2407 w2895 _ _]
          tunnel: w67 -> [_ _ w137 w292 w1100 w1511 w1821 w1904 _ _ _ _ w2406 w2893 _ _]
          tunnel: w66 -> [_ _ w136 w290 w1099 w1510 w1820 w1902 _ _ _ _ w2405 w2891 _ _]
          tunnel: w65 -> [_ _ w135 w288 w1098 w1509 w1819 w1901 _ _ _ _ w2404 w2889 _ _]
          tunnel: w64 -> [_ _ w134 w286 w1097 w1508 w1818 w1900 _ _ _ _ w2403 w2887 _ _]
          tunnel: w63 -> [_ _ w133 w284 w1096 w1507 w1817 w1899 _ _ _ _ w2402 w2885 _ _]
          tunnel: w62 -> [_ _ w132 w282 w1095 w1506 w1816 w1898 _ _ _ _ w2401 w2883 _ _]
          tunnel: w61 -> [_ _ w131 w280 w1094 w1505 w1815 w1897 _ _ _ _ w2400 w2881 _ _]
          tunnel: w60 -> [_ _ w130 w278 w1093 w1504 w1814 w1896 _ _ _ _ w2399 w2879 _ _]
          tunnel: w59 -> [_ _ w129 w276 w1092 w1503 w1813 w1895 _ _ _ _ w2398 w2877 _ _]
          tunnel: w58 -> [_ _ _ w293 w1091 w1502 _ _ _ _ _ _ _ w2897 _ _]
          tunnel: w57 -> [_ _ _ w291 w1090 w1500 _ _ _ _ _ _ _ w2892 _ _]
          tunnel: w56 -> [_ _ _ w289 w1089 w1499 _ _ _ _ _ _ _ w2890 _ _]
          tunnel: w55 -> [_ _ _ w287 w1088 w1498 _ _ _ _ _ _ _ w2888 _ _]
          tunnel: w54 -> [_ _ _ w285 w1087 w1497 _ _ _ _ _ _ _ w2886 _ _]
          tunnel: w53 -> [_ _ _ w283 w1086 w1496 _ _ _ _ _ _ _ w2884 _ _]
          tunnel: w52 -> [_ _ _ w281 w1085 w1495 _ _ _ _ _ _ _ w2882 _ _]
          tunnel: w51 -> [_ _ _ w279 w1084 w1494 _ _ _ _ _ _ _ w2880 _ _]
          tunnel: w50 -> [_ _ _ w277 w1083 w1493 _ _ _ _ _ _ _ w2878 _ _]
          tunnel: w49 -> [_ _ _ w275 w1082 w1492 _ _ _ _ _ _ _ w2876 _ _]
          frame #0 {
            w73 = FALSE
            w78 = 0.5
            # "set up cycle control"
            n65 = local read "jig cycle"() -> (w77:dbl)
            n66 = Divide(x="JIG ON TIME (S)", y=w78) -> (x/y=→"on loops":dbl)
            n67 = Divide(x="JIG OFF TIME (S)", y=w78) -> (x/y=→"off loops":dbl)
            n68 = Increment(x=w77) -> (x+1=w76:dbl)
            n69 = local write "TEMP update"(w73) -> ()
            n70 = local write "AI update"(w73) -> ()
            n71 = local write "jig cycle"(w76) -> ()
          }
          frame #1 {
            w118 = 60.0
            # "convert temperature rise minutes to cycles"
            n72 = local read "LAB05-2 (SET)"() -> (w82:T5)
            n73 = local read "LAB05-1 (SET)"() -> (w84:T5)
            n74 = local read "LAB04-2 (SET)"() -> (w86:T5)
            n75 = local read "LAB01-1 (SET)"() -> (w100:T5)
            n76 = local read "LAB01-2 (SET)"() -> (w98:T5)
            n77 = local read "LAB02-2 (SET)"() -> (w94:T5)
            n78 = local read "LAB04-1 (SET)"() -> (w88:T5)
            n79 = local read "LAB03-1 (SET)"() -> (w92:T5)
            n80 = local read "LAB03-2 (SET)"() -> (w90:T5)
            n81 = local read "LAB02-1 (SET)"() -> (w96:T5)
            n82 = local read "JIG OFF TIME (S)"() -> (w123:dbl)
            n83 = local read "JIG ON TIME (S)"() -> (w124:dbl)
            n84 = Unbundle(w82) -> ("T-RISE mins"=w81:dbl)  [unwired: 4 out]
            n85 = Unbundle(w84) -> ("T-RISE mins"=w83:dbl)  [unwired: 4 out]
            n86 = Unbundle(w100) -> ("T-RISE mins"=w99:dbl)  [unwired: 4 out]
            n87 = Unbundle(w86) -> ("T-RISE mins"=w85:dbl)  [unwired: 4 out]
            n88 = Unbundle(w98) -> ("T-RISE mins"=w97:dbl)  [unwired: 4 out]
            n89 = Unbundle(w96) -> ("T-RISE mins"=w95:dbl)  [unwired: 4 out]
            n90 = Unbundle(w88) -> ("T-RISE mins"=w87:dbl)  [unwired: 4 out]
            n91 = Unbundle(w94) -> ("T-RISE mins"=w93:dbl)  [unwired: 4 out]
            n92 = Unbundle(w90) -> ("T-RISE mins"=w89:dbl)  [unwired: 4 out]
            n93 = Unbundle(w92) -> ("T-RISE mins"=w91:dbl)  [unwired: 4 out]
            n94 = Add(x=w124, y=w123) -> (x+y=w117:dbl)
            n95 = Multiply(x=w118, y=w89) -> (x*y=w113:dbl)
            n96 = Multiply(x=w118, y=w87) -> (x*y=w112:dbl)
            n97 = Multiply(x=w118, y=w85) -> (x*y=w111:dbl)
            n98 = Multiply(x=w118, y=w83) -> (x*y=w110:dbl)
            n99 = Multiply(x=w118, y=w81) -> (x*y=w109:dbl)
            n100 = Multiply(x=w118, y=w97) -> (x*y=w119:dbl)
            n101 = Multiply(x=w118, y=w91) -> (x*y=w114:dbl)
            n102 = Multiply(x=w118, y=w99) -> (x*y=w120:dbl)
            n103 = Multiply(x=w118, y=w95) -> (x*y=w116:dbl)
            n104 = Multiply(x=w118, y=w93) -> (x*y=w115:dbl)
            n105 = Divide(x=w110, y=w117) -> (x/y=w102:dbl)
            n106 = Divide(x=w111, y=w117) -> (x/y=w103:dbl)
            n107 = Divide(x=w112, y=w117) -> (x/y=w104:dbl)
            n108 = Divide(x=w109, y=w117) -> (x/y=w101:dbl)
            n109 = Divide(x=w114, y=w117) -> (x/y=w106:dbl)
            n110 = Divide(x=w120, y=w117) -> (x/y=w122:dbl)
            n111 = Divide(x=w119, y=w117) -> (x/y=w121:dbl)
            n112 = Divide(x=w116, y=w117) -> (x/y=w108:dbl)
            n113 = Divide(x=w115, y=w117) -> (x/y=w107:dbl)
            n114 = Divide(x=w113, y=w117) -> (x/y=w105:dbl)
          }
          frame #2 {
            # "control cycle loops"
            n115 = local read "JIG OFF TIME (S)"() -> (w127:dbl)
            n116 = local read "JIG ON TIME (S)"() -> (w126:dbl)
            n117 = local read "jig cycle"() -> (w140:dbl)
            n118 = local read "on loops"() -> (w142:dbl)
            n119 = local read "off loops"() -> (w141:dbl)
            n120 = Add(x=w127, y=w126) -> (x+y=w125:dbl)
            n121 = Add(x=w142, y=w141) -> (x+y=w128:dbl)
            n122 = Greater Or Equal?(x=w140, y=w128) -> (x >= y?=w139:bool)
            n123 = case shown="True" w139 {
              tunnel: w138 -> [_ w153]
              tunnel: w137 -> [_ w152]
              tunnel: w136 -> [_ w151]
              tunnel: w135 -> [_ w150]
              tunnel: w134 -> [_ w149]
              tunnel: w133 -> [_ w148]
              tunnel: w132 -> [_ w147]
              tunnel: w131 -> [_ w146]
              tunnel: w130 -> [_ w145]
              tunnel: w129 -> [_ w144]
              tunnel: w125 -> [_ w143]
              frame False {
              }
              frame True {
                # "increment cycle value and convert cycles to minutes for temp rise"
                n124 = stacked-sequence {
                  tunnel: w153 -> [w163 _ _ _ _ _ _ _ _ _]
                  tunnel: w152 -> [_ w175 _ _ _ _ _ _ _ _]
                  tunnel: w151 -> [_ _ w187 _ _ _ _ _ _ _]
                  tunnel: w150 -> [_ _ _ w199 _ _ _ _ _ _]
                  tunnel: w149 -> [_ _ _ _ w211 _ _ _ _ _]
                  tunnel: w148 -> [_ _ _ _ _ w223 _ _ _ _]
                  tunnel: w147 -> [_ _ _ _ _ _ w235 _ _ _]
                  tunnel: w146 -> [_ _ _ _ _ _ _ w247 _ _]
                  tunnel: w145 -> [_ _ _ _ _ _ _ _ w259 _]
                  tunnel: w144 -> [_ _ _ _ _ _ _ _ _ w271]
                  tunnel: w143 -> [w160 w172 w184 w196 w208 w220 w232 w244 w256 w268]
                  frame #0 {
                    # "LAB01-1"
                    n125 = local read "LAB01-1 (DISP)"() -> (w158:T4)
                    n126 = Unbundle(w158) -> ("CYCLE"=w159:dbl)  [unwired: 2 out]
                    n127 = case shown="True" w163 {
                      tunnel: w159 -> [w164 w166]
                      tunnel: [w164 w165] -> w157
                      frame False {
                      }
                      frame True {
                        n128 = Increment(x=w166) -> (x+1=w165:dbl)
                      }
                    }
                    n129 = Multiply(x=w157, y=w160) -> (x*y=w161:dbl)
                    n130 = Divide(x=w161, y=60.0) -> (x/y=w156:dbl)
                    n131 = Bundle(cluster=w158, "CYCLE"=w157, "MINS"=w156) -> (w155:T4)  [unwired: 1 in]
                    n132 = local write "LAB01-1 (DISP)"(w155) -> ()
                  }
                  frame #1 {
                    # "update cycle value"
                    # "LAB01-2"
                    n133 = local read "LAB01-2 (DISP)"() -> (w170:T4)
                    n134 = Unbundle(w170) -> ("CYCLE"=w171:dbl)  [unwired: 2 out]
                    n135 = case shown="True" w175 {
                      tunnel: w171 -> [w176 w178]
                      tunnel: [w176 w177] -> w168
                      frame False {
                      }
                      frame True {
                        n136 = Increment(x=w178) -> (x+1=w177:dbl)
                      }
                    }
                    n137 = Multiply(x=w168, y=w172) -> (x*y=w173:dbl)
                    n138 = Divide(x=w173, y=60.0) -> (x/y=w167:dbl)
                    n139 = Bundle(cluster=w170, "CYCLE"=w168, "MINS"=w167) -> (w169:T4)  [unwired: 1 in]
                    n140 = local write "LAB01-2 (DISP)"(w169) -> ()
                  }
                  frame #2 {
                    # "update cycle value"
                    # "LAB02-1"
                    n141 = local read "LAB02-1 (DISP)"() -> (w182:T4)
                    n142 = Unbundle(w182) -> ("CYCLE"=w183:dbl)  [unwired: 2 out]
                    n143 = case shown="True" w187 {
                      tunnel: [w188 w190] -> w180
                      tunnel: w183 -> [w188 w189]
                      frame False {
                      }
                      frame True {
                        n144 = Increment(x=w189) -> (x+1=w190:dbl)
                      }
                    }
                    n145 = Multiply(x=w180, y=w184) -> (x*y=w185:dbl)
                    n146 = Divide(x=w185, y=60.0) -> (x/y=w179:dbl)
                    n147 = Bundle(cluster=w182, "CYCLE"=w180, "MINS"=w179) -> (w181:T4)  [unwired: 1 in]
                    n148 = local write "LAB02-1 (DISP)"(w181) -> ()
                  }
                  frame #3 {
                    # "update cycle value"
                    # "LAB02-2"
                    n149 = local read "LAB02-2 (DISP)"() -> (w194:T4)
                    n150 = Unbundle(w194) -> ("CYCLE"=w195:dbl)  [unwired: 2 out]
                    n151 = case shown="True" w199 {
                      tunnel: [w200 w202] -> w193
                      tunnel: w195 -> [w200 w201]
                      frame False {
                      }
                      frame True {
                        n152 = Increment(x=w201) -> (x+1=w202:dbl)
                      }
                    }
                    n153 = Multiply(x=w193, y=w196) -> (x*y=w197:dbl)
                    n154 = Divide(x=w197, y=60.0) -> (x/y=w192:dbl)
                    n155 = Bundle(cluster=w194, "CYCLE"=w193, "MINS"=w192) -> (w191:T4)  [unwired: 1 in]
                    n156 = local write "LAB02-2 (DISP)"(w191) -> ()
                  }
                  frame #4 {
                    # "update cycle value"
                    # "LAB03-1"
                    n157 = local read "LAB03-1 (DISP)"() -> (w206:T4)
                    n158 = Unbundle(w206) -> ("CYCLE"=w207:dbl)  [unwired: 2 out]
                    n159 = case shown="True" w211 {
                      tunnel: [w212 w214] -> w203
                      tunnel: w207 -> [w212 w213]
                      frame False {
                      }
                      frame True {
                        n160 = Increment(x=w213) -> (x+1=w214:dbl)
                      }
                    }
                    n161 = Multiply(x=w203, y=w208) -> (x*y=w209:dbl)
                    n162 = Divide(x=w209, y=60.0) -> (x/y=w204:dbl)
                    n163 = Bundle(cluster=w206, "CYCLE"=w203, "MINS"=w204) -> (w205:T4)  [unwired: 1 in]
                    n164 = local write "LAB03-1 (DISP)"(w205) -> ()
                  }
                  frame #5 {
                    # "update cycle value"
                    # "LAB03-2"
                    n165 = local read "LAB03-2 (DISP)"() -> (w218:T4)
                    n166 = Unbundle(w218) -> ("CYCLE"=w219:dbl)  [unwired: 2 out]
                    n167 = case shown="False" w223 {
                      tunnel: [w224 w226] -> w217
                      tunnel: w219 -> [w224 w225]
                      frame False {
                      }
                      frame True {
                        n168 = Increment(x=w225) -> (x+1=w226:dbl)
                      }
                    }
                    n169 = Multiply(x=w217, y=w220) -> (x*y=w221:dbl)
                    n170 = Divide(x=w221, y=60.0) -> (x/y=w216:dbl)
                    n171 = Bundle(cluster=w218, "CYCLE"=w217, "MINS"=w216) -> (w215:T4)  [unwired: 1 in]
                    n172 = local write "LAB03-2 (DISP)"(w215) -> ()
                  }
                  frame #6 {
                    # "update cycle value"
                    # "LAB04-1"
                    n173 = local read "LAB04-1 (DISP)"() -> (w230:T4)
                    n174 = Unbundle(w230) -> ("CYCLE"=w231:dbl)  [unwired: 2 out]
                    n175 = case shown="True" w235 {
                      tunnel: [w236 w238] -> w228
                      tunnel: w231 -> [w236 w237]
                      frame False {
                      }
                      frame True {
                        n176 = Increment(x=w237) -> (x+1=w238:dbl)
                      }
                    }
                    n177 = Multiply(x=w228, y=w232) -> (x*y=w233:dbl)
                    n178 = Divide(x=w233, y=60.0) -> (x/y=w227:dbl)
                    n179 = Bundle(cluster=w230, "CYCLE"=w228, "MINS"=w227) -> (w229:T4)  [unwired: 1 in]
                    n180 = local write "LAB04-1 (DISP)"(w229) -> ()
                  }
                  frame #7 {
                    # "update cycle value"
                    # "LAB04-2"
                    n181 = local read "LAB04-2 (DISP)"() -> (w242:T4)
                    n182 = Unbundle(w242) -> ("CYCLE"=w243:dbl)  [unwired: 2 out]
                    n183 = case shown="True" w247 {
                      tunnel: [w248 w250] -> w240
                      tunnel: w243 -> [w248 w249]
                      frame False {
                      }
                      frame True {
                        n184 = Increment(x=w249) -> (x+1=w250:dbl)
                      }
                    }
                    n185 = Multiply(x=w240, y=w244) -> (x*y=w246:dbl)
                    n186 = Divide(x=w246, y=60.0) -> (x/y=w239:dbl)
                    n187 = Bundle(cluster=w242, "CYCLE"=w240, "MINS"=w239) -> (w241:T4)  [unwired: 1 in]
                    n188 = local write "LAB04-2 (DISP)"(w241) -> ()
                  }
                  frame #8 {
                    # "update cycle value"
                    # "LAB05-1"
                    n189 = local read "LAB05-1 (DISP)"() -> (w254:T4)
                    n190 = Unbundle(w254) -> ("CYCLE"=w255:dbl)  [unwired: 2 out]
                    n191 = case shown="True" w259 {
                      tunnel: [w260 w262] -> w252
                      tunnel: w255 -> [w260 w261]
                      frame False {
                      }
                      frame True {
                        n192 = Increment(x=w261) -> (x+1=w262:dbl)
                      }
                    }
                    n193 = Multiply(x=w252, y=w256) -> (x*y=w257:dbl)
                    n194 = Divide(x=w257, y=60.0) -> (x/y=w251:dbl)
                    n195 = Bundle(cluster=w254, "CYCLE"=w252, "MINS"=w251) -> (w253:T4)  [unwired: 1 in]
                    n196 = local write "LAB05-1 (DISP)"(w253) -> ()
                  }
                  frame #9 {
                    # "update cycle value"
                    # "LAB05-2"
                    n197 = local read "LAB05-2 (DISP)"() -> (w267:T4)
                    n198 = Unbundle(w267) -> ("CYCLE"=w266:dbl)  [unwired: 2 out]
                    n199 = case shown="True" w271 {
                      tunnel: [w272 w274] -> w265
                      tunnel: w266 -> [w272 w273]
                      frame False {
                      }
                      frame True {
                        n200 = Increment(x=w273) -> (x+1=w274:dbl)
                      }
                    }
                    n201 = Multiply(x=w265, y=w268) -> (x*y=w269:dbl)
                    n202 = Divide(x=w269, y=60.0) -> (x/y=w264:dbl)
                    n203 = Bundle(cluster=w267, "CYCLE"=w265, "MINS"=w264) -> (w263:T4)  [unwired: 1 in]
                    n204 = local write "LAB05-2 (DISP)"(w263) -> ()
                  }
                }
                n205 = local write "jig cycle"(0) -> ()
              }
            }
          }
          frame #3 {
            # "START & STOP test RUN switch change, start test if true and stop test if false"
            n206 = Get Date/Time In Seconds() -> (seconds since 1Jan1904=w297:timestamp)
            n207 = Format Date/Time String(time format string (%c)="%Y%m%d", seconds (now)=w297) -> (date/time string=w298:string)  [unwired: 1 in]
            n208 = Format Date/Time String(time format string (%c)="%H%M", seconds (now)=w297) -> (date/time string=w295:string)  [unwired: 1 in]
            n209 = event shown="[1] \"LAB01-1RUN\": Value Change" {
              selector: _ -> [_ _ _ _ _ _ _ _ _ _ _]
              dyn-events: _ -> [_ _ _ _ _ _ _ _ _ _ _]
              timeout: 10 -> [_ _ _ _ _ _ _ _ _ _ _]
              tunnel: "c:\\crabtree\\Test Data\\" -> [_ w306 w384 w462 w540 w618 w696 w774 w852 w930 w1008]
              tunnel: w298 -> [_ w305 w383 w461 w539 w617 w695 w773 w851 w929 w1007]
              tunnel: w295 -> [_ w303 w382 w460 w538 w616 w694 w772 w850 w928 w1006]
              tunnel: w293 -> [_ w304 _ _ _ _ _ _ _ _ _]
              tunnel: w294 -> [_ _ _ _ _ _ _ _ _ _ _]
              tunnel: w292 -> [_ _ _ _ _ _ _ _ _ _ _]
              tunnel: w291 -> [_ _ w381 _ _ _ _ _ _ _ _]
              tunnel: w290 -> [_ _ _ _ _ _ _ _ _ _ _]
              tunnel: w289 -> [_ _ _ w459 _ _ _ _ _ _ _]
              tunnel: w288 -> [_ _ _ _ _ _ _ _ _ _ _]
              tunnel: w287 -> [_ _ _ _ w537 _ _ _ _ _ _]
              tunnel: w286 -> [_ _ _ _ _ _ _ _ _ _ _]
              tunnel: w285 -> [_ _ _ _ _ w615 _ _ _ _ _]
              tunnel: w284 -> [_ _ _ _ _ _ _ _ _ _ _]
              tunnel: w283 -> [_ _ _ _ _ _ w693 _ _ _ _]
              tunnel: w282 -> [_ _ _ _ _ _ _ _ _ _ _]
              tunnel: w281 -> [_ _ _ _ _ _ _ w771 _ _ _]
              tunnel: w280 -> [_ _ _ _ _ _ _ _ _ _ _]
              tunnel: w279 -> [_ _ _ _ _ _ _ _ w849 _ _]
              tunnel: w278 -> [_ _ _ _ _ _ _ _ _ _ _]
              tunnel: w277 -> [_ _ _ _ _ _ _ _ _ w927 _]
              tunnel: w276 -> [_ _ _ _ _ _ _ _ _ _ _]
              tunnel: w275 -> [_ _ _ _ _ _ _ _ _ _ w1005]
              event Timeout {
                n210 = event-data() -> ()  [unwired: 1 in, 3 out]
              }
              event "LAB01-1RUN": Value Change {
                n211 = event-data() -> ("NewVal"=w302:bool)  [unwired: 1 in, 5 out]
                n212 = case shown="True" w302 {
                  tunnel: w306 -> [_ w328]
                  tunnel: w305 -> [_ w327]
                  tunnel: w304 -> [w307 w326]
                  tunnel: w303 -> [_ w325]
                  frame False {
                    # "stop test"
                    n213 = stacked-sequence {
                      tunnel: w307 -> [w313 _]
                      frame #0 {
                        n214 = local read "LAB01-1 (DISP)"() -> (w312:T4)
                        n215 = Unbundle(w312) -> ("CYCLE"=w310:dbl, "MINS"=w311:dbl)  [unwired: 1 out]
                        n216 = case shown="\"CYCLE TEST\"" w313 {
                          tunnel: w311 -> [_ _ w320]
                          tunnel: w310 -> [w318 w319 _]
                          tunnel: [w318 w319 w320] -> w309
                          frame "TEST SET UP", Default {
                          }
                          frame "CYCLE TEST" {
                          }
                          frame "T-RISE TEST" {
                          }
                        }
                        n217 = local read "LAB01-1 (TDMS)"() -> (w317:refnum<k34>)
                        n218 = Build Array("STOPPED") -> (w314:string[])
                        n219 = Build Array(w309) -> (w308:dbl[])
                        n220 = TDMS Write(0:w317, 5:"TEST RESULT", 7:w314, 9:w308) -> ()  [unwired: 2 in, 4 out]
                      }
                      frame #1 {
                        n221 = local read "LAB01-1 (DISP)"() -> (w324:T4)
                        n222 = Bundle(cluster=w324, "STATUS"="STOP") -> (w322:T4)  [unwired: 2 in]
                        n223 = local write "LAB01-1 (RESULT)"(FALSE) -> ()
                        n224 = local write "LAB01-1 (DISP)"(w322) -> ()
                      }
                    }
                  }
                  frame True {
                    # "start new test and create test file"
                    n225 = stacked-sequence {
                      seq-local: [w334 _ _ _ _] -> [_ w353 _ _ _]
                      tunnel: w328 -> [w343 _ _ _ _]
                      tunnel: w327 -> [w341 _ _ _ _]
                      tunnel: w326 -> [w340 _ _ _ _]
                      tunnel: w325 -> [w331 _ _ _ _]
                      frame #0 {
                        n226 = local read "LAB01-1 (SET)"() -> (w333:T5)
                        n227 = case shown="\"TEST SET UP\", Default" w340 {
                          tunnel: ["TEST SET UP-" "CYCLE TEST-" "T-RISE TEST-"] -> w336
                          frame "TEST SET UP", Default {
                          }
                          frame "CYCLE TEST" {
                          }
                          frame "T-RISE TEST" {
                          }
                        }
                        n228 = Unbundle(w333) -> ("DESCRIPTION"=w332:string)  [unwired: 4 out]
                        n229 = Concatenate Strings(w343, "LAB01-1\\", w341, "\\") -> (w337:string)
                        n230 = String To Path(string=w337) -> (path=w339:path)
                        n231 = Concatenate Strings(w337, w336, w332, "-", w331, ".tdms") -> (w334:string)
                        n232 = Create Folder(path (use dialog)=w339) -> (error out=w338:errorcluster)  [unwired: 2 in, 2 out]
                        n233 = call <vilib>:"Clear Errors.vi"("error in (no error)"=w338) -> ()  [unwired: 6 in, 1 out]
                      }
                      frame #1 {
                        n234 = String To Path(string=w353) -> (path=w347:path)
                        n235 = TDMS Open(5:FALSE, 6:FALSE, 10:T14."create or replace" ("operation (0:open)"), 11:w347) -> (0:w349:errorcluster, 3:→"LAB01-1 (TDMS)":refnum<k34>)  [unwired: 3 in]
                        n236 = local write "data file error"(w349) -> ()
                      }
                      frame #2 {
                        n237 = local read "LAB01-1 (SET)"() -> (w359:T5)
                        n238 = local read "LAB01-1 (TDMS)"() -> (w370:refnum<k34>)
                        n239 = Build Array("Testers Name", "Description", "Set Test Cycles", "T-Rise minutes", "T-Rise Deg C") -> (w360:string[])
                        n240 = Unbundle(w359) -> ("NAME"=w358:string, "DESCRIPTION"=w357:string, "CYCLES"=w356:dbl, "T-RISE mins"=w355:dbl, "T-RISE deg C"=w354:dbl)
                        n241 = Number To Decimal String(number=w356) -> (decimal integer string=w369:string)  [unwired: 1 in]
                        n242 = Number To Decimal String(number=w355) -> (decimal integer string=w368:string)  [unwired: 1 in]
                        n243 = Number To Decimal String(number=w354) -> (decimal integer string=w367:string)  [unwired: 1 in]
                        n244 = Build Array(w358, w357, w369, w368, w367) -> (w366:string[])
                        n245 = TDMS Set Properties(5:w366, 7:w360, 11:w370) -> ()  [unwired: 3 in, 4 out]
                      }
                      frame #3 {
                        w371 = 0.0
                        n246 = local read "LAB01-1 (DISP)"() -> (w374:T4)
                        n247 = Bundle(cluster=w374, "CYCLE"=w371, "MINS"=w371, "STATUS"="RUN") -> (w373:T4)
                        n248 = local write "LAB01-1 (DISP)"(w373) -> ()
                      }
                      frame #4 {
                        n249 = local read "LAB01-1 (SIG)"() -> (w377:T2)
                        n250 = local read "LAB01-1 (TEMP START)"() -> (w379:cluster{"TL":dbl, "TN":dbl})
                        n251 = Unbundle(w377) -> ("Tmp Live"=w376:dbl, "Tmp Neut"=w375:dbl)  [unwired: 3 out]
                        n252 = Bundle(cluster=w379, "TL"=w376, "TN"=w375) -> (w378:cluster{"TL":dbl, "TN":dbl})
                        n253 = local write "LAB01-1 (TEMP START)"(w378) -> ()
                      }
                    }
                  }
                }
              }
              event "LAB01-2 RUN": Value Change {
                n254 = event-data() -> ("NewVal"=w380:bool)  [unwired: 1 in, 5 out]
                n255 = case shown="True" w380 {
                  tunnel: w384 -> [_ w406]
                  tunnel: w383 -> [_ w405]
                  tunnel: w381 -> [w385 w404]
                  tunnel: w382 -> [_ w403]
                  frame False {
                    # "stop test"
                    n256 = stacked-sequence {
                      tunnel: w385 -> [w391 _]
                      frame #0 {
                        n257 = local read "LAB01-2 (DISP)"() -> (w390:T4)
                        n258 = Unbundle(w390) -> ("CYCLE"=w388:dbl, "MINS"=w389:dbl)  [unwired: 1 out]
                        n259 = case shown="\"CYCLE TEST\"" w391 {
                          tunnel: w389 -> [_ _ w398]
                          tunnel: w388 -> [w396 w397 _]
                          tunnel: [w396 w397 w398] -> w387
                          frame "TEST SET UP", Default {
                          }
                          frame "CYCLE TEST" {
                          }
                          frame "T-RISE TEST" {
                          }
                        }
                        n260 = local read "LAB01-2 (TDMS)"() -> (w395:refnum<k34>)
                        n261 = Build Array("STOPPED") -> (w392:string[])
                        n262 = Build Array(w387) -> (w386:dbl[])
                        n263 = TDMS Write(0:w395, 5:"TEST RESULT", 7:w392, 9:w386) -> ()  [unwired: 2 in, 4 out]
                      }
                      frame #1 {
                        n264 = local read "LAB01-2 (DISP)"() -> (w402:T4)
                        n265 = Bundle(cluster=w402, "STATUS"="STOP") -> (w400:T4)  [unwired: 2 in]
                        n266 = local write "LAB01-2 (RESULT)"(FALSE) -> ()
                        n267 = local write "LAB01-2 (DISP)"(w400) -> ()
                      }
                    }
                  }
                  frame True {
                    # "start new test and create test file"
                    n268 = stacked-sequence {
                      seq-local: [w412 _ _ _ _] -> [_ w431 _ _ _]
                      tunnel: w406 -> [w421 _ _ _ _]
                      tunnel: w405 -> [w419 _ _ _ _]
                      tunnel: w404 -> [w418 _ _ _ _]
                      tunnel: w403 -> [w409 _ _ _ _]
                      frame #0 {
                        n269 = local read "LAB01-2 (SET)"() -> (w411:T5)
                        n270 = case shown="\"TEST SET UP\", Default" w418 {
                          tunnel: ["TEST SET UP-" "CYCLE TEST-" "T-RISE TEST-"] -> w414
                          frame "TEST SET UP", Default {
                          }
                          frame "CYCLE TEST" {
                          }
                          frame "T-RISE TEST" {
                          }
                        }
                        n271 = Unbundle(w411) -> ("DESCRIPTION"=w410:string)  [unwired: 4 out]
                        n272 = Concatenate Strings(w421, "LAB01-2\\", w419, "\\") -> (w415:string)
                        n273 = String To Path(string=w415) -> (path=w417:path)
                        n274 = Concatenate Strings(w415, w414, w410, "-", w409, ".tdms") -> (w412:string)
                        n275 = Create Folder(path (use dialog)=w417) -> (error out=w416:errorcluster)  [unwired: 2 in, 2 out]
                        n276 = call <vilib>:"Clear Errors.vi"("error in (no error)"=w416) -> ()  [unwired: 6 in, 1 out]
                      }
                      frame #1 {
                        n277 = String To Path(string=w431) -> (path=w425:path)
                        n278 = TDMS Open(5:FALSE, 6:FALSE, 10:T14."create or replace" ("operation (0:open)"), 11:w425) -> (0:w427:errorcluster, 3:→"LAB01-2 (TDMS)":refnum<k34>)  [unwired: 3 in]
                        n279 = local write "data file error"(w427) -> ()
                      }
                      frame #2 {
                        n280 = local read "LAB01-2 (SET)"() -> (w437:T5)
                        n281 = local read "LAB01-2 (TDMS)"() -> (w448:refnum<k34>)
                        n282 = Build Array("Testers Name", "Description", "Set Test Cycles", "T-Rise minutes", "T-Rise Deg C") -> (w438:string[])
                        n283 = Unbundle(w437) -> ("NAME"=w436:string, "DESCRIPTION"=w435:string, "CYCLES"=w434:dbl, "T-RISE mins"=w433:dbl, "T-RISE deg C"=w432:dbl)
                        n284 = Number To Decimal String(number=w434) -> (decimal integer string=w447:string)  [unwired: 1 in]
                        n285 = Number To Decimal String(number=w433) -> (decimal integer string=w446:string)  [unwired: 1 in]
                        n286 = Number To Decimal String(number=w432) -> (decimal integer string=w445:string)  [unwired: 1 in]
                        n287 = Build Array(w436, w435, w447, w446, w445) -> (w444:string[])
                        n288 = TDMS Set Properties(5:w444, 7:w438, 11:w448) -> ()  [unwired: 3 in, 4 out]
                      }
                      frame #3 {
                        w450 = 0.0
                        n289 = local read "LAB01-2 (DISP)"() -> (w452:T4)
                        n290 = Bundle(cluster=w452, "CYCLE"=w450, "MINS"=w450, "STATUS"="RUN") -> (w451:T4)
                        n291 = local write "LAB01-2 (DISP)"(w451) -> ()
                      }
                      frame #4 {
                        n292 = local read "LAB01-2 (SIG)"() -> (w455:T2)
                        n293 = local read "LAB01-2 (TEMP START)"() -> (w457:cluster{"TL":dbl, "TN":dbl})
                        n294 = Unbundle(w455) -> ("Tmp Live"=w454:dbl, "Tmp Neut"=w453:dbl)  [unwired: 3 out]
                        n295 = Bundle(cluster=w457, "TL"=w454, "TN"=w453) -> (w456:cluster{"TL":dbl, "TN":dbl})
                        n296 = local write "LAB01-2 (TEMP START)"(w456) -> ()
                      }
                    }
                  }
                }
              }
              event "LAB02-1 RUN": Value Change {
                n297 = event-data() -> ("NewVal"=w458:bool)  [unwired: 1 in, 5 out]
                n298 = case shown="True" w458 {
                  tunnel: w462 -> [_ w484]
                  tunnel: w461 -> [_ w483]
                  tunnel: w459 -> [w463 w482]
                  tunnel: w460 -> [_ w481]
                  frame False {
                    # "stop test"
                    n299 = stacked-sequence {
                      tunnel: w463 -> [w469 _]
                      frame #0 {
                        n300 = local read "LAB02-1 (DISP)"() -> (w468:T4)
                        n301 = Unbundle(w468) -> ("CYCLE"=w466:dbl, "MINS"=w467:dbl)  [unwired: 1 out]
                        n302 = case shown="\"CYCLE TEST\"" w469 {
                          tunnel: w467 -> [_ _ w476]
                          tunnel: w466 -> [w474 w475 _]
                          tunnel: [w474 w475 w476] -> w465
                          frame "TEST SET UP", Default {
                          }
                          frame "CYCLE TEST" {
                          }
                          frame "T-RISE TEST" {
                          }
                        }
                        n303 = local read "LAB02-1 (TDMS)"() -> (w473:refnum<k34>)
                        n304 = Build Array("STOPPED") -> (w470:string[])
                        n305 = Build Array(w465) -> (w464:dbl[])
                        n306 = TDMS Write(0:w473, 5:"TEST RESULT", 7:w470, 9:w464) -> ()  [unwired: 2 in, 4 out]
                      }
                      frame #1 {
                        n307 = local read "LAB02-1 (DISP)"() -> (w480:T4)
                        n308 = Bundle(cluster=w480, "STATUS"="STOPPED") -> (w478:T4)  [unwired: 2 in]
                        n309 = local write "LAB02-1 (RESULT)"(FALSE) -> ()
                        n310 = local write "LAB02-1 (DISP)"(w478) -> ()
                      }
                    }
                  }
                  frame True {
                    # "start new test and create test file"
                    n311 = stacked-sequence {
                      seq-local: [w490 _ _ _ _] -> [_ w509 _ _ _]
                      tunnel: w484 -> [w499 _ _ _ _]
                      tunnel: w483 -> [w497 _ _ _ _]
                      tunnel: w482 -> [w496 _ _ _ _]
                      tunnel: w481 -> [w487 _ _ _ _]
                      frame #0 {
                        n312 = local read "LAB02-1 (SET)"() -> (w489:T5)
                        n313 = case shown="\"TEST SET UP\", Default" w496 {
                          tunnel: ["TEST SET UP-" "CYCLE TEST-" "T-RISE TEST-"] -> w492
                          frame "TEST SET UP", Default {
                          }
                          frame "CYCLE TEST" {
                          }
                          frame "T-RISE TEST" {
                          }
                        }
                        n314 = Unbundle(w489) -> ("DESCRIPTION"=w488:string)  [unwired: 4 out]
                        n315 = Concatenate Strings(w499, "LAB02-1\\", w497, "\\") -> (w493:string)
                        n316 = String To Path(string=w493) -> (path=w495:path)
                        n317 = Concatenate Strings(w493, w492, w488, "-", w487, ".tdms") -> (w490:string)
                        n318 = Create Folder(path (use dialog)=w495) -> (error out=w494:errorcluster)  [unwired: 2 in, 2 out]
                        n319 = call <vilib>:"Clear Errors.vi"("error in (no error)"=w494) -> ()  [unwired: 6 in, 1 out]
                      }
                      frame #1 {
                        n320 = String To Path(string=w509) -> (path=w503:path)
                        n321 = TDMS Open(5:FALSE, 6:FALSE, 10:T14."create or replace" ("operation (0:open)"), 11:w503) -> (0:w505:errorcluster, 3:→"LAB02-1 (TDMS)":refnum<k34>)  [unwired: 3 in]
                        n322 = local write "data file error"(w505) -> ()
                      }
                      frame #2 {
                        n323 = local read "LAB02-1 (SET)"() -> (w515:T5)
                        n324 = local read "LAB02-1 (TDMS)"() -> (w526:refnum<k34>)
                        n325 = Build Array("Testers Name", "Description", "Set Test Cycles", "T-Rise minutes", "T-Rise Deg C") -> (w516:string[])
                        n326 = Unbundle(w515) -> ("NAME"=w514:string, "DESCRIPTION"=w513:string, "CYCLES"=w512:dbl, "T-RISE mins"=w511:dbl, "T-RISE deg C"=w510:dbl)
                        n327 = Number To Decimal String(number=w512) -> (decimal integer string=w525:string)  [unwired: 1 in]
                        n328 = Number To Decimal String(number=w511) -> (decimal integer string=w524:string)  [unwired: 1 in]
                        n329 = Number To Decimal String(number=w510) -> (decimal integer string=w523:string)  [unwired: 1 in]
                        n330 = Build Array(w514, w513, w525, w524, w523) -> (w522:string[])
                        n331 = TDMS Set Properties(5:w522, 7:w516, 11:w526) -> ()  [unwired: 3 in, 4 out]
                      }
                      frame #3 {
                        w528 = 0.0
                        n332 = local read "LAB02-1 (DISP)"() -> (w530:T4)
                        n333 = Bundle(cluster=w530, "CYCLE"=w528, "MINS"=w528, "STATUS"="RUN") -> (w529:T4)
                        n334 = local write "LAB02-1 (DISP)"(w529) -> ()
                      }
                      frame #4 {
                        n335 = local read "LAB02-1 (SIG)"() -> (w533:T2)
                        n336 = local read "LAB02-1 (TEMP START)"() -> (w535:cluster{"TL":dbl, "TN":dbl})
                        n337 = Unbundle(w533) -> ("Tmp Live"=w532:dbl, "Tmp Neut"=w531:dbl)  [unwired: 3 out]
                        n338 = Bundle(cluster=w535, "TL"=w532, "TN"=w531) -> (w534:cluster{"TL":dbl, "TN":dbl})
                        n339 = local write "LAB02-1 (TEMP START)"(w534) -> ()
                      }
                    }
                  }
                }
              }
              event "LAB02-2 RUN": Value Change {
                n340 = event-data() -> ("NewVal"=w536:bool)  [unwired: 1 in, 5 out]
                n341 = case shown="True" w536 {
                  tunnel: w540 -> [_ w562]
                  tunnel: w539 -> [_ w561]
                  tunnel: w537 -> [w541 w560]
                  tunnel: w538 -> [_ w559]
                  frame False {
                    # "stop test"
                    n342 = stacked-sequence {
                      tunnel: w541 -> [w547 _]
                      frame #0 {
                        n343 = local read "LAB02-2 (DISP)"() -> (w546:T4)
                        n344 = Unbundle(w546) -> ("CYCLE"=w544:dbl, "MINS"=w545:dbl)  [unwired: 1 out]
                        n345 = case shown="\"CYCLE TEST\"" w547 {
                          tunnel: w545 -> [_ _ w554]
                          tunnel: w544 -> [w552 w553 _]
                          tunnel: [w552 w553 w554] -> w543
                          frame "TEST SET UP", Default {
                          }
                          frame "CYCLE TEST" {
                          }
                          frame "T-RISE TEST" {
                          }
                        }
                        n346 = local read "LAB02-2 (TDMS)"() -> (w551:refnum<k34>)
                        n347 = Build Array("STOPPED") -> (w548:string[])
                        n348 = Build Array(w543) -> (w542:dbl[])
                        n349 = TDMS Write(0:w551, 5:"TEST RESULT", 7:w548, 9:w542) -> ()  [unwired: 2 in, 4 out]
                      }
                      frame #1 {
                        n350 = local read "LAB02-2 (DISP)"() -> (w558:T4)
                        n351 = Bundle(cluster=w558, "STATUS"="STOP") -> (w556:T4)  [unwired: 2 in]
                        n352 = local write "LAB02-2 (RESULT)"(FALSE) -> ()
                        n353 = local write "LAB02-2 (DISP)"(w556) -> ()
                      }
                    }
                  }
                  frame True {
                    # "start new test and create test file"
                    n354 = stacked-sequence {
                      seq-local: [w568 _ _ _ _] -> [_ w587 _ _ _]
                      tunnel: w562 -> [w577 _ _ _ _]
                      tunnel: w561 -> [w575 _ _ _ _]
                      tunnel: w560 -> [w574 _ _ _ _]
                      tunnel: w559 -> [w565 _ _ _ _]
                      frame #0 {
                        n355 = local read "LAB02-2 (SET)"() -> (w567:T5)
                        n356 = case shown="\"TEST SET UP\", Default" w574 {
                          tunnel: ["TEST SET UP-" "CYCLE TEST-" "T-RISE TEST-"] -> w570
                          frame "TEST SET UP", Default {
                          }
                          frame "CYCLE TEST" {
                          }
                          frame "T-RISE TEST" {
                          }
                        }
                        n357 = Unbundle(w567) -> ("DESCRIPTION"=w566:string)  [unwired: 4 out]
                        n358 = Concatenate Strings(w577, "LAB02-2\\", w575, "\\") -> (w571:string)
                        n359 = String To Path(string=w571) -> (path=w573:path)
                        n360 = Concatenate Strings(w571, w570, w566, "-", w565, ".tdms") -> (w568:string)
                        n361 = Create Folder(path (use dialog)=w573) -> (error out=w572:errorcluster)  [unwired: 2 in, 2 out]
                        n362 = call <vilib>:"Clear Errors.vi"("error in (no error)"=w572) -> ()  [unwired: 6 in, 1 out]
                      }
                      frame #1 {
                        n363 = String To Path(string=w587) -> (path=w581:path)
                        n364 = TDMS Open(5:FALSE, 6:FALSE, 10:T14."create or replace" ("operation (0:open)"), 11:w581) -> (0:w583:errorcluster, 3:→"LAB02-2 (TDMS)":refnum<k34>)  [unwired: 3 in]
                        n365 = local write "data file error"(w583) -> ()
                      }
                      frame #2 {
                        n366 = local read "LAB02-2 (SET)"() -> (w593:T5)
                        n367 = local read "LAB02-2 (TDMS)"() -> (w604:refnum<k34>)
                        n368 = Build Array("Testers Name", "Description", "Set Test Cycles", "T-Rise minutes", "T-Rise Deg C") -> (w594:string[])
                        n369 = Unbundle(w593) -> ("NAME"=w592:string, "DESCRIPTION"=w591:string, "CYCLES"=w590:dbl, "T-RISE mins"=w589:dbl, "T-RISE deg C"=w588:dbl)
                        n370 = Number To Decimal String(number=w590) -> (decimal integer string=w603:string)  [unwired: 1 in]
                        n371 = Number To Decimal String(number=w589) -> (decimal integer string=w602:string)  [unwired: 1 in]
                        n372 = Number To Decimal String(number=w588) -> (decimal integer string=w601:string)  [unwired: 1 in]
                        n373 = Build Array(w592, w591, w603, w602, w601) -> (w600:string[])
                        n374 = TDMS Set Properties(5:w600, 7:w594, 11:w604) -> ()  [unwired: 3 in, 4 out]
                      }
                      frame #3 {
                        w606 = 0.0
                        n375 = local read "LAB02-2 (DISP)"() -> (w608:T4)
                        n376 = Bundle(cluster=w608, "CYCLE"=w606, "MINS"=w606, "STATUS"="RUN") -> (w607:T4)
                        n377 = local write "LAB02-2 (DISP)"(w607) -> ()
                      }
                      frame #4 {
                        n378 = local read "LAB02-2 (SIG)"() -> (w611:T2)
                        n379 = local read "LAB02-2 (TEMP START)"() -> (w613:cluster{"TL":dbl, "TN":dbl})
                        n380 = Unbundle(w611) -> ("Tmp Live"=w610:dbl, "Tmp Neut"=w609:dbl)  [unwired: 3 out]
                        n381 = Bundle(cluster=w613, "TL"=w610, "TN"=w609) -> (w612:cluster{"TL":dbl, "TN":dbl})
                        n382 = local write "LAB02-2 (TEMP START)"(w612) -> ()
                      }
                    }
                  }
                }
              }
              event "LAB03-1 RUN": Value Change {
                n383 = event-data() -> ("NewVal"=w614:bool)  [unwired: 1 in, 5 out]
                n384 = case shown="True" w614 {
                  tunnel: w618 -> [_ w640]
                  tunnel: w617 -> [_ w639]
                  tunnel: w615 -> [w619 w638]
                  tunnel: w616 -> [_ w637]
                  frame False {
                    # "stop test"
                    n385 = stacked-sequence {
                      tunnel: w619 -> [w625 _]
                      frame #0 {
                        n386 = local read "LAB03-1 (DISP)"() -> (w624:T4)
                        n387 = Unbundle(w624) -> ("CYCLE"=w622:dbl, "MINS"=w623:dbl)  [unwired: 1 out]
                        n388 = case shown="\"CYCLE TEST\"" w625 {
                          tunnel: w623 -> [_ _ w632]
                          tunnel: w622 -> [w630 w631 _]
                          tunnel: [w630 w631 w632] -> w621
                          frame "TEST SET UP", Default {
                          }
                          frame "CYCLE TEST" {
                          }
                          frame "T-RISE TEST" {
                          }
                        }
                        n389 = local read "LAB03-1 (TDMS)"() -> (w629:refnum<k34>)
                        n390 = Build Array("STOPPED") -> (w626:string[])
                        n391 = Build Array(w621) -> (w620:dbl[])
                        n392 = TDMS Write(0:w629, 5:"TEST RESULT", 7:w626, 9:w620) -> ()  [unwired: 2 in, 4 out]
                      }
                      frame #1 {
                        n393 = local read "LAB03-1 (DISP)"() -> (w636:T4)
                        n394 = Bundle(cluster=w636, "STATUS"="STOP") -> (w634:T4)  [unwired: 2 in]
                        n395 = local write "LAB03-1 (RESULT)"(FALSE) -> ()
                        n396 = local write "LAB03-1 (DISP)"(w634) -> ()
                      }
                    }
                  }
                  frame True {
                    # "start new test and create test file"
                    n397 = stacked-sequence {
                      seq-local: [w646 _ _ _ _] -> [_ w665 _ _ _]
                      tunnel: w640 -> [w655 _ _ _ _]
                      tunnel: w639 -> [w653 _ _ _ _]
                      tunnel: w638 -> [w652 _ _ _ _]
                      tunnel: w637 -> [w643 _ _ _ _]
                      frame #0 {
                        n398 = local read "LAB03-1 (SET)"() -> (w645:T5)
                        n399 = case shown="\"TEST SET UP\", Default" w652 {
                          tunnel: ["TEST SET UP-" "CYCLE TEST-" "T-RISE TEST-"] -> w648
                          frame "TEST SET UP", Default {
                          }
                          frame "CYCLE TEST" {
                          }
                          frame "T-RISE TEST" {
                          }
                        }
                        n400 = Unbundle(w645) -> ("DESCRIPTION"=w644:string)  [unwired: 4 out]
                        n401 = Concatenate Strings(w655, "LAB03-1\\", w653, "\\") -> (w649:string)
                        n402 = String To Path(string=w649) -> (path=w651:path)
                        n403 = Concatenate Strings(w649, w648, w644, "-", w643, ".tdms") -> (w646:string)
                        n404 = Create Folder(path (use dialog)=w651) -> (error out=w650:errorcluster)  [unwired: 2 in, 2 out]
                        n405 = call <vilib>:"Clear Errors.vi"("error in (no error)"=w650) -> ()  [unwired: 6 in, 1 out]
                      }
                      frame #1 {
                        n406 = String To Path(string=w665) -> (path=w659:path)
                        n407 = TDMS Open(5:FALSE, 6:FALSE, 10:T14."create or replace" ("operation (0:open)"), 11:w659) -> (0:w661:errorcluster, 3:→"LAB03-1 (TDMS)":refnum<k34>)  [unwired: 3 in]
                        n408 = local write "data file error"(w661) -> ()
                      }
                      frame #2 {
                        n409 = local read "LAB03-1 (SET)"() -> (w671:T5)
                        n410 = local read "LAB03-1 (TDMS)"() -> (w682:refnum<k34>)
                        n411 = Build Array("Testers Name", "Description", "Set Test Cycles", "T-Rise minutes", "T-Rise Deg C") -> (w672:string[])
                        n412 = Unbundle(w671) -> ("NAME"=w670:string, "DESCRIPTION"=w669:string, "CYCLES"=w668:dbl, "T-RISE mins"=w667:dbl, "T-RISE deg C"=w666:dbl)
                        n413 = Number To Decimal String(number=w668) -> (decimal integer string=w681:string)  [unwired: 1 in]
                        n414 = Number To Decimal String(number=w667) -> (decimal integer string=w680:string)  [unwired: 1 in]
                        n415 = Number To Decimal String(number=w666) -> (decimal integer string=w679:string)  [unwired: 1 in]
                        n416 = Build Array(w670, w669, w681, w680, w679) -> (w678:string[])
                        n417 = TDMS Set Properties(5:w678, 7:w672, 11:w682) -> ()  [unwired: 3 in, 4 out]
                      }
                      frame #3 {
                        w684 = 0.0
                        n418 = local read "LAB03-1 (DISP)"() -> (w686:T4)
                        n419 = Bundle(cluster=w686, "CYCLE"=w684, "MINS"=w684, "STATUS"="RUN") -> (w685:T4)
                        n420 = local write "LAB03-1 (DISP)"(w685) -> ()
                      }
                      frame #4 {
                        n421 = local read "LAB03-1 (SIG)"() -> (w689:T2)
                        n422 = local read "LAB03-1 (TEMP START)"() -> (w691:cluster{"TL":dbl, "TN":dbl})
                        n423 = Unbundle(w689) -> ("Tmp Live"=w688:dbl, "Tmp Neut"=w687:dbl)  [unwired: 3 out]
                        n424 = Bundle(cluster=w691, "TL"=w688, "TN"=w687) -> (w690:cluster{"TL":dbl, "TN":dbl})
                        n425 = local write "LAB03-1 (TEMP START)"(w690) -> ()
                      }
                    }
                  }
                }
              }
              event "LAB03-2 RUN": Value Change {
                n426 = event-data() -> ("NewVal"=w692:bool)  [unwired: 1 in, 5 out]
                n427 = case shown="True" w692 {
                  tunnel: w696 -> [_ w718]
                  tunnel: w695 -> [_ w717]
                  tunnel: w693 -> [w697 w716]
                  tunnel: w694 -> [_ w715]
                  frame False {
                    # "stop test"
                    n428 = stacked-sequence {
                      tunnel: w697 -> [w703 _]
                      frame #0 {
                        n429 = local read "LAB03-2 (DISP)"() -> (w702:T4)
                        n430 = Unbundle(w702) -> ("CYCLE"=w700:dbl, "MINS"=w701:dbl)  [unwired: 1 out]
                        n431 = case shown="\"CYCLE TEST\"" w703 {
                          tunnel: w701 -> [_ _ w710]
                          tunnel: w700 -> [w708 w709 _]
                          tunnel: [w708 w709 w710] -> w699
                          frame "TEST SET UP", Default {
                          }
                          frame "CYCLE TEST" {
                          }
                          frame "T-RISE TEST" {
                          }
                        }
                        n432 = local read "LAB03-2 (TDMS)"() -> (w707:refnum<k34>)
                        n433 = Build Array("STOPPED") -> (w704:string[])
                        n434 = Build Array(w699) -> (w698:dbl[])
                        n435 = TDMS Write(0:w707, 5:"TEST RESULT", 7:w704, 9:w698) -> ()  [unwired: 2 in, 4 out]
                      }
                      frame #1 {
                        n436 = local read "LAB03-2 (DISP)"() -> (w714:T4)
                        n437 = Bundle(cluster=w714, "STATUS"="STOP") -> (w712:T4)  [unwired: 2 in]
                        n438 = local write "LAB03-2 (RESULT)"(FALSE) -> ()
                        n439 = local write "LAB03-2 (DISP)"(w712) -> ()
                      }
                    }
                  }
                  frame True {
                    # "start new test and create test file"
                    n440 = stacked-sequence {
                      seq-local: [w724 _ _ _ _] -> [_ w743 _ _ _]
                      tunnel: w718 -> [w733 _ _ _ _]
                      tunnel: w717 -> [w731 _ _ _ _]
                      tunnel: w716 -> [w730 _ _ _ _]
                      tunnel: w715 -> [w721 _ _ _ _]
                      frame #0 {
                        n441 = local read "LAB03-2 (SET)"() -> (w723:T5)
                        n442 = case shown="\"TEST SET UP\", Default" w730 {
                          tunnel: ["TEST SET UP-" "CYCLE TEST-" "T-RISE TEST-"] -> w726
                          frame "TEST SET UP", Default {
                          }
                          frame "CYCLE TEST" {
                          }
                          frame "T-RISE TEST" {
                          }
                        }
                        n443 = Unbundle(w723) -> ("DESCRIPTION"=w722:string)  [unwired: 4 out]
                        n444 = Concatenate Strings(w733, "LAB03-2\\", w731, "\\") -> (w727:string)
                        n445 = String To Path(string=w727) -> (path=w729:path)
                        n446 = Concatenate Strings(w727, w726, w722, "-", w721, ".tdms") -> (w724:string)
                        n447 = Create Folder(path (use dialog)=w729) -> (error out=w728:errorcluster)  [unwired: 2 in, 2 out]
                        n448 = call <vilib>:"Clear Errors.vi"("error in (no error)"=w728) -> ()  [unwired: 6 in, 1 out]
                      }
                      frame #1 {
                        n449 = String To Path(string=w743) -> (path=w737:path)
                        n450 = TDMS Open(5:FALSE, 6:FALSE, 10:T14."create or replace" ("operation (0:open)"), 11:w737) -> (0:w739:errorcluster, 3:→"LAB03-2 (TDMS)":refnum<k34>)  [unwired: 3 in]
                        n451 = local write "data file error"(w739) -> ()
                      }
                      frame #2 {
                        n452 = local read "LAB03-2 (SET)"() -> (w749:T5)
                        n453 = local read "LAB03-2 (TDMS)"() -> (w760:refnum<k34>)
                        n454 = Build Array("Testers Name", "Description", "Set Test Cycles", "T-Rise minutes", "T-Rise Deg C") -> (w750:string[])
                        n455 = Unbundle(w749) -> ("NAME"=w748:string, "DESCRIPTION"=w747:string, "CYCLES"=w746:dbl, "T-RISE mins"=w745:dbl, "T-RISE deg C"=w744:dbl)
                        n456 = Number To Decimal String(number=w746) -> (decimal integer string=w759:string)  [unwired: 1 in]
                        n457 = Number To Decimal String(number=w745) -> (decimal integer string=w758:string)  [unwired: 1 in]
                        n458 = Number To Decimal String(number=w744) -> (decimal integer string=w757:string)  [unwired: 1 in]
                        n459 = Build Array(w748, w747, w759, w758, w757) -> (w756:string[])
                        n460 = TDMS Set Properties(5:w756, 7:w750, 11:w760) -> ()  [unwired: 3 in, 4 out]
                      }
                      frame #3 {
                        w762 = 0.0
                        n461 = local read "LAB03-2 (DISP)"() -> (w764:T4)
                        n462 = Bundle(cluster=w764, "CYCLE"=w762, "MINS"=w762, "STATUS"="RUN") -> (w763:T4)
                        n463 = local write "LAB03-2 (DISP)"(w763) -> ()
                      }
                      frame #4 {
                        n464 = local read "LAB03-2 (SIG)"() -> (w767:T2)
                        n465 = local read "LAB03-2 (TEMP START)"() -> (w769:cluster{"TL":dbl, "TN":dbl})
                        n466 = Unbundle(w767) -> ("Tmp Live"=w766:dbl, "Tmp Neut"=w765:dbl)  [unwired: 3 out]
                        n467 = Bundle(cluster=w769, "TL"=w766, "TN"=w765) -> (w768:cluster{"TL":dbl, "TN":dbl})
                        n468 = local write "LAB03-2 (TEMP START)"(w768) -> ()
                      }
                    }
                  }
                }
              }
              event "LAB04-1 RUN": Value Change {
                n469 = event-data() -> ("NewVal"=w770:bool)  [unwired: 1 in, 5 out]
                n470 = case shown="True" w770 {
                  tunnel: w774 -> [_ w796]
                  tunnel: w773 -> [_ w795]
                  tunnel: w771 -> [w775 w794]
                  tunnel: w772 -> [_ w793]
                  frame False {
                    # "stop test"
                    n471 = stacked-sequence {
                      tunnel: w775 -> [w781 _]
                      frame #0 {
                        n472 = local read "LAB04-1 (DISP)"() -> (w780:T4)
                        n473 = Unbundle(w780) -> ("CYCLE"=w778:dbl, "MINS"=w779:dbl)  [unwired: 1 out]
                        n474 = case shown="\"CYCLE TEST\"" w781 {
                          tunnel: w779 -> [_ _ w788]
                          tunnel: w778 -> [w786 w787 _]
                          tunnel: [w786 w787 w788] -> w777
                          frame "TEST SET UP", Default {
                          }
                          frame "CYCLE TEST" {
                          }
                          frame "T-RISE TEST" {
                          }
                        }
                        n475 = local read "LAB04-1 (TDMS)"() -> (w785:refnum<k34>)
                        n476 = Build Array("STOPPED") -> (w782:string[])
                        n477 = Build Array(w777) -> (w776:dbl[])
                        n478 = TDMS Write(0:w785, 5:"TEST RESULT", 7:w782, 9:w776) -> ()  [unwired: 2 in, 4 out]
                      }
                      frame #1 {
                        n479 = local read "LAB04-1 (DISP)"() -> (w792:T4)
                        n480 = Bundle(cluster=w792, "STATUS"="STOP") -> (w790:T4)  [unwired: 2 in]
                        n481 = local write "LAB04-1 (RESULT)"(FALSE) -> ()
                        n482 = local write "LAB04-1 (DISP)"(w790) -> ()
                      }
                    }
                  }
                  frame True {
                    # "start new test and create test file"
                    n483 = stacked-sequence {
                      seq-local: [w802 _ _ _ _] -> [_ w821 _ _ _]
                      tunnel: w796 -> [w811 _ _ _ _]
                      tunnel: w795 -> [w809 _ _ _ _]
                      tunnel: w794 -> [w808 _ _ _ _]
                      tunnel: w793 -> [w799 _ _ _ _]
                      frame #0 {
                        n484 = local read "LAB04-1 (SET)"() -> (w801:T5)
                        n485 = case shown="\"TEST SET UP\", Default" w808 {
                          tunnel: ["TEST SET UP-" "CYCLE TEST-" "T-RISE TEST-"] -> w804
                          frame "TEST SET UP", Default {
                          }
                          frame "CYCLE TEST" {
                          }
                          frame "T-RISE TEST" {
                          }
                        }
                        n486 = Unbundle(w801) -> ("DESCRIPTION"=w800:string)  [unwired: 4 out]
                        n487 = Concatenate Strings(w811, "LAB04-1\\", w809, "\\") -> (w805:string)
                        n488 = String To Path(string=w805) -> (path=w807:path)
                        n489 = Concatenate Strings(w805, w804, w800, "-", w799, ".tdms") -> (w802:string)
                        n490 = Create Folder(path (use dialog)=w807) -> (error out=w806:errorcluster)  [unwired: 2 in, 2 out]
                        n491 = call <vilib>:"Clear Errors.vi"("error in (no error)"=w806) -> ()  [unwired: 6 in, 1 out]
                      }
                      frame #1 {
                        n492 = String To Path(string=w821) -> (path=w815:path)
                        n493 = TDMS Open(5:FALSE, 6:FALSE, 10:T14."create or replace" ("operation (0:open)"), 11:w815) -> (0:w817:errorcluster, 3:→"LAB04-1 (TDMS)":refnum<k34>)  [unwired: 3 in]
                        n494 = local write "data file error"(w817) -> ()
                      }
                      frame #2 {
                        n495 = local read "LAB04-1 (SET)"() -> (w827:T5)
                        n496 = local read "LAB04-1 (TDMS)"() -> (w838:refnum<k34>)
                        n497 = Build Array("Testers Name", "Description", "Set Test Cycles", "T-Rise minutes", "T-Rise Deg C") -> (w828:string[])
                        n498 = Unbundle(w827) -> ("NAME"=w826:string, "DESCRIPTION"=w825:string, "CYCLES"=w824:dbl, "T-RISE mins"=w823:dbl, "T-RISE deg C"=w822:dbl)
                        n499 = Number To Decimal String(number=w824) -> (decimal integer string=w837:string)  [unwired: 1 in]
                        n500 = Number To Decimal String(number=w823) -> (decimal integer string=w836:string)  [unwired: 1 in]
                        n501 = Number To Decimal String(number=w822) -> (decimal integer string=w835:string)  [unwired: 1 in]
                        n502 = Build Array(w826, w825, w837, w836, w835) -> (w834:string[])
                        n503 = TDMS Set Properties(5:w834, 7:w828, 11:w838) -> ()  [unwired: 3 in, 4 out]
                      }
                      frame #3 {
                        w840 = 0.0
                        n504 = local read "LAB04-1 (DISP)"() -> (w842:T4)
                        n505 = Bundle(cluster=w842, "CYCLE"=w840, "MINS"=w840, "STATUS"="RUN") -> (w841:T4)
                        n506 = local write "LAB04-1 (DISP)"(w841) -> ()
                      }
                      frame #4 {
                        n507 = local read "LAB04-1 (SIG)"() -> (w845:T2)
                        n508 = local read "LAB04-1 (TEMP START)"() -> (w847:cluster{"TL":dbl, "TN":dbl})
                        n509 = Unbundle(w845) -> ("Tmp Live"=w844:dbl, "Tmp Neut"=w843:dbl)  [unwired: 3 out]
                        n510 = Bundle(cluster=w847, "TL"=w844, "TN"=w843) -> (w846:cluster{"TL":dbl, "TN":dbl})
                        n511 = local write "LAB04-1 (TEMP START)"(w846) -> ()
                      }
                    }
                  }
                }
              }
              event "LAB04-2 RUN": Value Change {
                n512 = event-data() -> ("NewVal"=w848:bool)  [unwired: 1 in, 5 out]
                n513 = case shown="True" w848 {
                  tunnel: w852 -> [_ w874]
                  tunnel: w851 -> [_ w873]
                  tunnel: w849 -> [w853 w872]
                  tunnel: w850 -> [_ w871]
                  frame False {
                    # "stop test"
                    n514 = stacked-sequence {
                      tunnel: w853 -> [w859 _]
                      frame #0 {
                        n515 = local read "LAB04-2 (DISP)"() -> (w858:T4)
                        n516 = Unbundle(w858) -> ("CYCLE"=w856:dbl, "MINS"=w857:dbl)  [unwired: 1 out]
                        n517 = case shown="\"CYCLE TEST\"" w859 {
                          tunnel: w857 -> [_ _ w866]
                          tunnel: w856 -> [w864 w865 _]
                          tunnel: [w864 w865 w866] -> w855
                          frame "TEST SET UP", Default {
                          }
                          frame "CYCLE TEST" {
                          }
                          frame "T-RISE TEST" {
                          }
                        }
                        n518 = local read "LAB04-2 (TDMS)"() -> (w863:refnum<k34>)
                        n519 = Build Array("STOPPED") -> (w860:string[])
                        n520 = Build Array(w855) -> (w854:dbl[])
                        n521 = TDMS Write(0:w863, 5:"TEST RESULT", 7:w860, 9:w854) -> ()  [unwired: 2 in, 4 out]
                      }
                      frame #1 {
                        n522 = local read "LAB04-2 (DISP)"() -> (w870:T4)
                        n523 = Bundle(cluster=w870, "STATUS"="STOP") -> (w868:T4)  [unwired: 2 in]
                        n524 = local write "LAB04-2 (RESULT)"(FALSE) -> ()
                        n525 = local write "LAB04-2 (DISP)"(w868) -> ()
                      }
                    }
                  }
                  frame True {
                    # "start new test and create test file"
                    n526 = stacked-sequence {
                      seq-local: [w880 _ _ _ _] -> [_ w899 _ _ _]
                      tunnel: w874 -> [w889 _ _ _ _]
                      tunnel: w873 -> [w887 _ _ _ _]
                      tunnel: w872 -> [w886 _ _ _ _]
                      tunnel: w871 -> [w877 _ _ _ _]
                      frame #0 {
                        n527 = local read "LAB04-2 (SET)"() -> (w879:T5)
                        n528 = case shown="\"TEST SET UP\", Default" w886 {
                          tunnel: ["TEST SET UP-" "CYCLE TEST-" "T-RISE TEST-"] -> w882
                          frame "TEST SET UP", Default {
                          }
                          frame "CYCLE TEST" {
                          }
                          frame "T-RISE TEST" {
                          }
                        }
                        n529 = Unbundle(w879) -> ("DESCRIPTION"=w878:string)  [unwired: 4 out]
                        n530 = Concatenate Strings(w889, "LAB04-2\\", w887, "\\") -> (w883:string)
                        n531 = String To Path(string=w883) -> (path=w885:path)
                        n532 = Concatenate Strings(w883, w882, w878, "-", w877, ".tdms") -> (w880:string)
                        n533 = Create Folder(path (use dialog)=w885) -> (error out=w884:errorcluster)  [unwired: 2 in, 2 out]
                        n534 = call <vilib>:"Clear Errors.vi"("error in (no error)"=w884) -> ()  [unwired: 6 in, 1 out]
                      }
                      frame #1 {
                        n535 = String To Path(string=w899) -> (path=w893:path)
                        n536 = TDMS Open(5:FALSE, 6:FALSE, 10:T14."create or replace" ("operation (0:open)"), 11:w893) -> (0:w895:errorcluster, 3:→"LAB04-2 (TDMS)":refnum<k34>)  [unwired: 3 in]
                        n537 = local write "data file error"(w895) -> ()
                      }
                      frame #2 {
                        n538 = local read "LAB04-2 (SET)"() -> (w905:T5)
                        n539 = local read "LAB04-2 (TDMS)"() -> (w916:refnum<k34>)
                        n540 = Build Array("Testers Name", "Description", "Set Test Cycles", "T-Rise minutes", "T-Rise Deg C") -> (w906:string[])
                        n541 = Unbundle(w905) -> ("NAME"=w904:string, "DESCRIPTION"=w903:string, "CYCLES"=w902:dbl, "T-RISE mins"=w901:dbl, "T-RISE deg C"=w900:dbl)
                        n542 = Number To Decimal String(number=w902) -> (decimal integer string=w915:string)  [unwired: 1 in]
                        n543 = Number To Decimal String(number=w901) -> (decimal integer string=w914:string)  [unwired: 1 in]
                        n544 = Number To Decimal String(number=w900) -> (decimal integer string=w913:string)  [unwired: 1 in]
                        n545 = Build Array(w904, w903, w915, w914, w913) -> (w912:string[])
                        n546 = TDMS Set Properties(5:w912, 7:w906, 11:w916) -> ()  [unwired: 3 in, 4 out]
                      }
                      frame #3 {
                        w918 = 0.0
                        n547 = local read "LAB04-2 (DISP)"() -> (w920:T4)
                        n548 = Bundle(cluster=w920, "CYCLE"=w918, "MINS"=w918, "STATUS"="RUN") -> (w919:T4)
                        n549 = local write "LAB04-2 (DISP)"(w919) -> ()
                      }
                      frame #4 {
                        n550 = local read "LAB04-2 (SIG)"() -> (w923:T2)
                        n551 = local read "LAB04-2 (TEMP START)"() -> (w925:cluster{"TL":dbl, "TN":dbl})
                        n552 = Unbundle(w923) -> ("Tmp Live"=w922:dbl, "Tmp Neut"=w921:dbl)  [unwired: 3 out]
                        n553 = Bundle(cluster=w925, "TL"=w922, "TN"=w921) -> (w924:cluster{"TL":dbl, "TN":dbl})
                        n554 = local write "LAB04-2 (TEMP START)"(w924) -> ()
                      }
                    }
                  }
                }
              }
              event "LAB05-1 RUN": Value Change {
                n555 = event-data() -> ("NewVal"=w926:bool)  [unwired: 1 in, 5 out]
                n556 = case shown="True" w926 {
                  tunnel: w930 -> [_ w952]
                  tunnel: w929 -> [_ w951]
                  tunnel: w927 -> [w931 w950]
                  tunnel: w928 -> [_ w949]
                  frame False {
                    # "stop test"
                    n557 = stacked-sequence {
                      tunnel: w931 -> [w937 _]
                      frame #0 {
                        n558 = local read "LAB05-1 (DISP)"() -> (w936:T4)
                        n559 = Unbundle(w936) -> ("CYCLE"=w934:dbl, "MINS"=w935:dbl)  [unwired: 1 out]
                        n560 = case shown="\"CYCLE TEST\"" w937 {
                          tunnel: w935 -> [_ _ w944]
                          tunnel: w934 -> [w942 w943 _]
                          tunnel: [w942 w943 w944] -> w933
                          frame "TEST SET UP", Default {
                          }
                          frame "CYCLE TEST" {
                          }
                          frame "T-RISE TEST" {
                          }
                        }
                        n561 = local read "LAB05-1 (TDMS)"() -> (w941:refnum<k34>)
                        n562 = Build Array("STOPPED") -> (w938:string[])
                        n563 = Build Array(w933) -> (w932:dbl[])
                        n564 = TDMS Write(0:w941, 5:"TEST RESULT", 7:w938, 9:w932) -> ()  [unwired: 2 in, 4 out]
                      }
                      frame #1 {
                        n565 = local read "LAB05-1 (DISP)"() -> (w948:T4)
                        n566 = Bundle(cluster=w948, "STATUS"="STOP") -> (w946:T4)  [unwired: 2 in]
                        n567 = local write "LAB05-1 (RESULT)"(FALSE) -> ()
                        n568 = local write "LAB05-1 (DISP)"(w946) -> ()
                      }
                    }
                  }
                  frame True {
                    # "start new test and create test file"
                    n569 = stacked-sequence {
                      seq-local: [w958 _ _ _ _] -> [_ w977 _ _ _]
                      tunnel: w952 -> [w967 _ _ _ _]
                      tunnel: w951 -> [w965 _ _ _ _]
                      tunnel: w950 -> [w964 _ _ _ _]
                      tunnel: w949 -> [w955 _ _ _ _]
                      frame #0 {
                        n570 = local read "LAB05-1 (SET)"() -> (w957:T5)
                        n571 = case shown="\"TEST SET UP\", Default" w964 {
                          tunnel: ["TEST SET UP-" "CYCLE TEST-" "T-RISE TEST-"] -> w960
                          frame "TEST SET UP", Default {
                          }
                          frame "CYCLE TEST" {
                          }
                          frame "T-RISE TEST" {
                          }
                        }
                        n572 = Unbundle(w957) -> ("DESCRIPTION"=w956:string)  [unwired: 4 out]
                        n573 = Concatenate Strings(w967, "LAB05-1\\", w965, "\\") -> (w961:string)
                        n574 = String To Path(string=w961) -> (path=w963:path)
                        n575 = Concatenate Strings(w961, w960, w956, "-", w955, ".tdms") -> (w958:string)
                        n576 = Create Folder(path (use dialog)=w963) -> (error out=w962:errorcluster)  [unwired: 2 in, 2 out]
                        n577 = call <vilib>:"Clear Errors.vi"("error in (no error)"=w962) -> ()  [unwired: 6 in, 1 out]
                      }
                      frame #1 {
                        n578 = String To Path(string=w977) -> (path=w971:path)
                        n579 = TDMS Open(5:FALSE, 6:FALSE, 10:T14."create or replace" ("operation (0:open)"), 11:w971) -> (0:w973:errorcluster, 3:→"LAB05-1 (TDMS)":refnum<k34>)  [unwired: 3 in]
                        n580 = local write "data file error"(w973) -> ()
                      }
                      frame #2 {
                        n581 = local read "LAB05-1 (SET)"() -> (w983:T5)
                        n582 = local read "LAB05-1 (TDMS)"() -> (w994:refnum<k34>)
                        n583 = Build Array("Testers Name", "Description", "Set Test Cycles", "T-Rise minutes", "T-Rise Deg C") -> (w984:string[])
                        n584 = Unbundle(w983) -> ("NAME"=w982:string, "DESCRIPTION"=w981:string, "CYCLES"=w980:dbl, "T-RISE mins"=w979:dbl, "T-RISE deg C"=w978:dbl)
                        n585 = Number To Decimal String(number=w980) -> (decimal integer string=w993:string)  [unwired: 1 in]
                        n586 = Number To Decimal String(number=w979) -> (decimal integer string=w992:string)  [unwired: 1 in]
                        n587 = Number To Decimal String(number=w978) -> (decimal integer string=w991:string)  [unwired: 1 in]
                        n588 = Build Array(w982, w981, w993, w992, w991) -> (w990:string[])
                        n589 = TDMS Set Properties(5:w990, 7:w984, 11:w994) -> ()  [unwired: 3 in, 4 out]
                      }
                      frame #3 {
                        w996 = 0.0
                        n590 = local read "LAB05-1 (DISP)"() -> (w998:T4)
                        n591 = Bundle(cluster=w998, "CYCLE"=w996, "MINS"=w996, "STATUS"="RUN") -> (w997:T4)
                        n592 = local write "LAB05-1 (DISP)"(w997) -> ()
                      }
                      frame #4 {
                        n593 = local read "LAB05-1 (SIG)"() -> (w1001:T2)
                        n594 = local read "LAB05-1 (TEMP START)"() -> (w1003:cluster{"TL":dbl, "TN":dbl})
                        n595 = Unbundle(w1001) -> ("Tmp Live"=w1000:dbl, "Tmp Neut"=w999:dbl)  [unwired: 3 out]
                        n596 = Bundle(cluster=w1003, "TL"=w1000, "TN"=w999) -> (w1002:cluster{"TL":dbl, "TN":dbl})
                        n597 = local write "LAB05-1 (TEMP START)"(w1002) -> ()
                      }
                    }
                  }
                }
              }
              event "LAB05-2 RUN": Value Change {
                n598 = event-data() -> ("NewVal"=w1004:bool)  [unwired: 1 in, 5 out]
                n599 = case shown="True" w1004 {
                  tunnel: w1008 -> [_ w1030]
                  tunnel: w1007 -> [_ w1029]
                  tunnel: w1005 -> [w1009 w1028]
                  tunnel: w1006 -> [_ w1027]
                  frame False {
                    # "stop test"
                    n600 = stacked-sequence {
                      tunnel: w1009 -> [w1015 _]
                      frame #0 {
                        n601 = local read "LAB05-2 (DISP)"() -> (w1014:T4)
                        n602 = Unbundle(w1014) -> ("CYCLE"=w1012:dbl, "MINS"=w1013:dbl)  [unwired: 1 out]
                        n603 = case shown="\"CYCLE TEST\"" w1015 {
                          tunnel: w1013 -> [_ _ w1022]
                          tunnel: w1012 -> [w1020 w1021 _]
                          tunnel: [w1020 w1021 w1022] -> w1011
                          frame "TEST SET UP", Default {
                          }
                          frame "CYCLE TEST" {
                          }
                          frame "T-RISE TEST" {
                          }
                        }
                        n604 = local read "LAB05-2 (TDMS)"() -> (w1019:refnum<k34>)
                        n605 = Build Array("STOPPED") -> (w1016:string[])
                        n606 = Build Array(w1011) -> (w1010:dbl[])
                        n607 = TDMS Write(0:w1019, 5:"TEST RESULT", 7:w1016, 9:w1010) -> ()  [unwired: 2 in, 4 out]
                      }
                      frame #1 {
                        n608 = local read "LAB05-2 (DISP)"() -> (w1026:T4)
                        n609 = Bundle(cluster=w1026, "STATUS"="STOP") -> (w1024:T4)  [unwired: 2 in]
                        n610 = local write "LAB05-2 (RESULT)"(FALSE) -> ()
                        n611 = local write "LAB05-2 (DISP)"(w1024) -> ()
                      }
                    }
                  }
                  frame True {
                    # "start new test and create test file"
                    n612 = stacked-sequence {
                      seq-local: [w1036 _ _ _ _] -> [_ w1055 _ _ _]
                      tunnel: w1030 -> [w1045 _ _ _ _]
                      tunnel: w1029 -> [w1043 _ _ _ _]
                      tunnel: w1028 -> [w1042 _ _ _ _]
                      tunnel: w1027 -> [w1033 _ _ _ _]
                      frame #0 {
                        n613 = local read "LAB05-2 (SET)"() -> (w1035:T5)
                        n614 = case shown="\"TEST SET UP\", Default" w1042 {
                          tunnel: ["TEST SET UP-" "CYCLE TEST-" "T-RISE TEST-"] -> w1038
                          frame "TEST SET UP", Default {
                          }
                          frame "CYCLE TEST" {
                          }
                          frame "T-RISE TEST" {
                          }
                        }
                        n615 = Unbundle(w1035) -> ("DESCRIPTION"=w1034:string)  [unwired: 4 out]
                        n616 = Concatenate Strings(w1045, "LAB05-2\\", w1043, "\\") -> (w1039:string)
                        n617 = String To Path(string=w1039) -> (path=w1041:path)
                        n618 = Concatenate Strings(w1039, w1038, w1034, "-", w1033, ".tdms") -> (w1036:string)
                        n619 = Create Folder(path (use dialog)=w1041) -> (error out=w1040:errorcluster)  [unwired: 2 in, 2 out]
                        n620 = call <vilib>:"Clear Errors.vi"("error in (no error)"=w1040) -> ()  [unwired: 6 in, 1 out]
                      }
                      frame #1 {
                        n621 = String To Path(string=w1055) -> (path=w1049:path)
                        n622 = TDMS Open(5:FALSE, 6:FALSE, 10:T14."create or replace" ("operation (0:open)"), 11:w1049) -> (0:w1051:errorcluster, 3:→"LAB05-2 (TDMS)":refnum<k34>)  [unwired: 3 in]
                        n623 = local write "data file error"(w1051) -> ()
                      }
                      frame #2 {
                        n624 = local read "LAB05-2 (SET)"() -> (w1061:T5)
                        n625 = local read "LAB05-2 (TDMS)"() -> (w1072:refnum<k34>)
                        n626 = Build Array("Testers Name", "Description", "Set Test Cycles", "T-Rise minutes", "T-Rise Deg C") -> (w1062:string[])
                        n627 = Unbundle(w1061) -> ("NAME"=w1060:string, "DESCRIPTION"=w1059:string, "CYCLES"=w1058:dbl, "T-RISE mins"=w1057:dbl, "T-RISE deg C"=w1056:dbl)
                        n628 = Number To Decimal String(number=w1058) -> (decimal integer string=w1071:string)  [unwired: 1 in]
                        n629 = Number To Decimal String(number=w1057) -> (decimal integer string=w1070:string)  [unwired: 1 in]
                        n630 = Number To Decimal String(number=w1056) -> (decimal integer string=w1069:string)  [unwired: 1 in]
                        n631 = Build Array(w1060, w1059, w1071, w1070, w1069) -> (w1068:string[])
                        n632 = TDMS Set Properties(5:w1068, 7:w1062, 11:w1072) -> ()  [unwired: 3 in, 4 out]
                      }
                      frame #3 {
                        w1074 = 0.0
                        n633 = local read "LAB05-2 (DISP)"() -> (w1076:T4)
                        n634 = Bundle(cluster=w1076, "CYCLE"=w1074, "MINS"=w1074, "STATUS"="RUN") -> (w1075:T4)
                        n635 = local write "LAB05-2 (DISP)"(w1075) -> ()
                      }
                      frame #4 {
                        n636 = local read "LAB05-2 (SIG)"() -> (w1079:T2)
                        n637 = local read "LAB05-2 (TEMP START)"() -> (w1081:cluster{"TL":dbl, "TN":dbl})
                        n638 = Unbundle(w1079) -> ("Tmp Live"=w1078:dbl, "Tmp Neut"=w1077:dbl)  [unwired: 3 out]
                        n639 = Bundle(cluster=w1081, "TL"=w1078, "TN"=w1077) -> (w1080:cluster{"TL":dbl, "TN":dbl})
                        n640 = local write "LAB05-2 (TEMP START)"(w1080) -> ()
                      }
                    }
                  }
                }
              }
            }
          }
          frame #4 {
            # "check if test cycles reached for cycle tests, if so then test pass"
            n641 = stacked-sequence {
              tunnel: w1101 -> [_ _ _ _ _ _ _ _ _ _]
              tunnel: w1100 -> [_ _ _ _ _ _ _ _ _ _]
              tunnel: w1099 -> [_ _ _ _ _ _ _ _ _ _]
              tunnel: w1098 -> [_ _ _ _ _ _ _ _ _ _]
              tunnel: w1097 -> [_ _ _ _ _ _ _ _ _ _]
              tunnel: w1096 -> [_ _ _ _ _ _ _ _ _ _]
              tunnel: w1095 -> [_ _ _ _ _ _ _ _ _ _]
              tunnel: w1094 -> [_ _ _ _ _ _ _ _ _ _]
              tunnel: w1093 -> [_ _ _ _ _ _ _ _ _ _]
              tunnel: w1092 -> [_ _ _ _ _ _ _ _ _ _]
              tunnel: w1091 -> [w1106 _ _ _ _ _ _ _ _ _]
              tunnel: w1090 -> [_ w1141 _ _ _ _ _ _ _ _]
              tunnel: w1089 -> [_ _ w1180 _ _ _ _ _ _ _]
              tunnel: w1088 -> [_ _ _ w1219 _ _ _ _ _ _]
              tunnel: w1087 -> [_ _ _ _ w1258 _ _ _ _ _]
              tunnel: w1086 -> [_ _ _ _ _ w1297 _ _ _ _]
              tunnel: w1085 -> [_ _ _ _ _ _ w1336 _ _ _]
              tunnel: w1084 -> [_ _ _ _ _ _ _ w1375 _ _]
              tunnel: w1083 -> [_ _ _ _ _ _ _ _ w1414 _]
              tunnel: w1082 -> [_ _ _ _ _ _ _ _ _ w1453]
              frame #0 {
                # "LAB01-1"
                n642 = Less?(x=w1106, y=2) -> (x < y?=w1104:bool)
                n643 = local read "LAB01-1 (DISP)"() -> (w1107:T4)
                n644 = Unbundle(w1107) -> ("STATUS"=w1108:string)  [unwired: 2 out]
                n645 = Equal?(x=w1108, y="RUN") -> (x = y?=w1103:bool)
                n646 = And(x=w1103, y=w1104) -> (x .and. y?=w1102:bool)
                n647 = case shown="True" w1102 {
                  tunnel: w1107 -> [_ w1111]
                  tunnel: w1106 -> [_ w1116]
                  frame False {
                  }
                  frame True {
                    n648 = local read "LAB01-1 (SET)"() -> (w1118:T5)
                    n649 = local read "LAB01-1 (TDMS)"() -> (w1110:refnum<k34>)
                    n650 = Unbundle(w1111) -> ("CYCLE"=w1117:dbl)  [unwired: 2 out]
                    n651 = Unbundle(w1118) -> ("CYCLES"=w1113:dbl, "T-RISE mins"=w1115:dbl)  [unwired: 3 out]
                    n652 = case shown="\"TEST SET UP\", Default" w1116 {
                      tunnel: w1115 -> [_ _ w1125]
                      tunnel: [w1120 w1122 w1125] -> w1114
                      tunnel: w1113 -> [w1120 w1122 _]
                      tunnel: ["TEST SET UP CYCLES" "CYCLES" "T-RISE TEST"] -> w1112
                      frame "TEST SET UP", Default {
                      }
                      frame "CYCLE TEST" {
                      }
                      frame "T-RISE TEST" {
                      }
                    }
                    n653 = Greater Or Equal?(x=w1117, y=w1113) -> (x >= y?=w1119:bool)
                    n654 = case shown="True" w1119 {
                      tunnel: w1114 -> [w1129 _]
                      tunnel: w1112 -> [w1128 _]
                      tunnel: w1111 -> [w1127 _]
                      tunnel: w1110 -> [w1126 _]
                      frame True {
                        n655 = stacked-sequence {
                          tunnel: w1129 -> [w1133 _]
                          tunnel: w1128 -> [w1131 _]
                          tunnel: w1127 -> [_ w1139]
                          tunnel: w1126 -> [w1130 _]
                          frame #0 {
                            n656 = Build Array(w1131) -> (w1134:string[])
                            n657 = Build Array(w1133) -> (w1132:dbl[])
                            n658 = TDMS Write(0:w1130, 5:"TEST PASS", 7:w1134, 9:w1132) -> (15:w1136:errorcluster)  [unwired: 2 in, 3 out]
                            n659 = local write "data file error"(w1136) -> ()
                          }
                          frame #1 {
                            n660 = Bundle(cluster=w1139, "STATUS"="CYCLE PASS") -> (w1137:T4)  [unwired: 2 in]
                            n661 = local write "LAB01-1 (RESULT)"(TRUE) -> ()
                            n662 = local write "LAB01-1 (DISP)"(w1137) -> ()
                          }
                        }
                      }
                      frame False {
                      }
                    }
                  }
                }
              }
              frame #1 {
                # "LAB01-2"
                n663 = Less?(x=w1141, y=2) -> (x < y?=w1144:bool)
                n664 = local read "LAB01-2 (DISP)"() -> (w1146:T4)
                n665 = Unbundle(w1146) -> ("STATUS"=w1147:string)  [unwired: 2 out]
                n666 = Equal?(x=w1147, y="RUN") -> (x = y?=w1143:bool)
                n667 = And(x=w1143, y=w1144) -> (x .and. y?=w1142:bool)
                n668 = case shown="True" w1142 {
                  tunnel: w1146 -> [_ w1150]
                  tunnel: w1141 -> [_ w1155]
                  frame False {
                  }
                  frame True {
                    n669 = local read "LAB01-2 (SET)"() -> (w1157:T5)
                    n670 = local read "LAB01-2 (TDMS)"() -> (w1149:refnum<k34>)
                    n671 = Unbundle(w1150) -> ("CYCLE"=w1156:dbl)  [unwired: 2 out]
                    n672 = Unbundle(w1157) -> ("CYCLES"=w1152:dbl, "T-RISE mins"=w1154:dbl)  [unwired: 3 out]
                    n673 = case shown="\"TEST SET UP\", Default" w1155 {
                      tunnel: w1154 -> [_ _ w1164]
                      tunnel: [w1159 w1161 w1164] -> w1153
                      tunnel: w1152 -> [w1159 w1161 _]
                      tunnel: ["TEST SET UP CYCLES" "CYCLES" "T-RISE TEST"] -> w1151
                      frame "TEST SET UP", Default {
                      }
                      frame "CYCLE TEST" {
                      }
                      frame "T-RISE TEST" {
                      }
                    }
                    n674 = Greater Or Equal?(x=w1156, y=w1152) -> (x >= y?=w1158:bool)
                    n675 = case shown="True" w1158 {
                      tunnel: w1153 -> [w1168 _]
                      tunnel: w1151 -> [w1167 _]
                      tunnel: w1150 -> [w1166 _]
                      tunnel: w1149 -> [w1165 _]
                      frame True {
                        n676 = stacked-sequence {
                          tunnel: w1168 -> [w1172 _]
                          tunnel: w1167 -> [w1170 _]
                          tunnel: w1166 -> [_ w1178]
                          tunnel: w1165 -> [w1169 _]
                          frame #0 {
                            n677 = Build Array(w1170) -> (w1173:string[])
                            n678 = Build Array(w1172) -> (w1171:dbl[])
                            n679 = TDMS Write(0:w1169, 5:"TEST PASS", 7:w1173, 9:w1171) -> (15:w1175:errorcluster)  [unwired: 2 in, 3 out]
                            n680 = local write "data file error"(w1175) -> ()
                          }
                          frame #1 {
                            n681 = Bundle(cluster=w1178, "STATUS"="CYCLE PASS") -> (w1176:T4)  [unwired: 2 in]
                            n682 = local write "LAB01-2 (RESULT)"(TRUE) -> ()
                            n683 = local write "LAB01-2 (DISP)"(w1176) -> ()
                          }
                        }
                      }
                      frame False {
                      }
                    }
                  }
                }
              }
              frame #2 {
                # "LAB02-1"
                n684 = Less?(x=w1180, y=2) -> (x < y?=w1183:bool)
                n685 = local read "LAB02-1 (DISP)"() -> (w1185:T4)
                n686 = Unbundle(w1185) -> ("STATUS"=w1186:string)  [unwired: 2 out]
                n687 = Equal?(x=w1186, y="RUN") -> (x = y?=w1182:bool)
                n688 = And(x=w1182, y=w1183) -> (x .and. y?=w1181:bool)
                n689 = case shown="True" w1181 {
                  tunnel: w1185 -> [_ w1189]
                  tunnel: w1180 -> [_ w1194]
                  frame False {
                  }
                  frame True {
                    n690 = local read "LAB02-1 (SET)"() -> (w1196:T5)
                    n691 = local read "LAB02-1 (TDMS)"() -> (w1188:refnum<k34>)
                    n692 = Unbundle(w1189) -> ("CYCLE"=w1195:dbl)  [unwired: 2 out]
                    n693 = Unbundle(w1196) -> ("CYCLES"=w1191:dbl, "T-RISE mins"=w1193:dbl)  [unwired: 3 out]
                    n694 = case shown="\"TEST SET UP\", Default" w1194 {
                      tunnel: w1193 -> [_ _ w1203]
                      tunnel: [w1198 w1200 w1203] -> w1192
                      tunnel: w1191 -> [w1198 w1200 _]
                      tunnel: ["TEST SET UP CYCLES" "CYCLES" "T-RISE TEST"] -> w1190
                      frame "TEST SET UP", Default {
                      }
                      frame "CYCLE TEST" {
                      }
                      frame "T-RISE TEST" {
                      }
                    }
                    n695 = Greater Or Equal?(x=w1195, y=w1191) -> (x >= y?=w1197:bool)
                    n696 = case shown="True" w1197 {
                      tunnel: w1192 -> [w1207 _]
                      tunnel: w1190 -> [w1206 _]
                      tunnel: w1189 -> [w1205 _]
                      tunnel: w1188 -> [w1204 _]
                      frame True {
                        n697 = stacked-sequence {
                          tunnel: w1207 -> [w1211 _]
                          tunnel: w1206 -> [w1209 _]
                          tunnel: w1205 -> [_ w1217]
                          tunnel: w1204 -> [w1208 _]
                          frame #0 {
                            n698 = Build Array(w1209) -> (w1212:string[])
                            n699 = Build Array(w1211) -> (w1210:dbl[])
                            n700 = TDMS Write(0:w1208, 5:"TEST PASS", 7:w1212, 9:w1210) -> (15:w1214:errorcluster)  [unwired: 2 in, 3 out]
                            n701 = local write "data file error"(w1214) -> ()
                          }
                          frame #1 {
                            n702 = Bundle(cluster=w1217, "STATUS"="CYCLE PASS") -> (w1215:T4)  [unwired: 2 in]
                            n703 = local write "LAB02-1 (RESULT)"(TRUE) -> ()
                            n704 = local write "LAB02-1 (DISP)"(w1215) -> ()
                          }
                        }
                      }
                      frame False {
                      }
                    }
                  }
                }
              }
              frame #3 {
                # "LAB02-2"
                n705 = Less?(x=w1219, y=2) -> (x < y?=w1222:bool)
                n706 = local read "LAB02-2 (DISP)"() -> (w1224:T4)
                n707 = Unbundle(w1224) -> ("STATUS"=w1225:string)  [unwired: 2 out]
                n708 = Equal?(x=w1225, y="RUN") -> (x = y?=w1221:bool)
                n709 = And(x=w1221, y=w1222) -> (x .and. y?=w1220:bool)
                n710 = case shown="True" w1220 {
                  tunnel: w1224 -> [_ w1228]
                  tunnel: w1219 -> [_ w1233]
                  frame False {
                  }
                  frame True {
                    n711 = local read "LAB02-2 (SET)"() -> (w1235:T5)
                    n712 = local read "LAB02-2 (TDMS)"() -> (w1227:refnum<k34>)
                    n713 = Unbundle(w1228) -> ("CYCLE"=w1234:dbl)  [unwired: 2 out]
                    n714 = Unbundle(w1235) -> ("CYCLES"=w1230:dbl, "T-RISE mins"=w1232:dbl)  [unwired: 3 out]
                    n715 = case shown="\"TEST SET UP\", Default" w1233 {
                      tunnel: w1232 -> [_ _ w1242]
                      tunnel: [w1237 w1239 w1242] -> w1231
                      tunnel: w1230 -> [w1237 w1239 _]
                      tunnel: ["TEST SET UP CYCLES" "CYCLES" "T-RISE TEST"] -> w1229
                      frame "TEST SET UP", Default {
                      }
                      frame "CYCLE TEST" {
                      }
                      frame "T-RISE TEST" {
                      }
                    }
                    n716 = Greater Or Equal?(x=w1234, y=w1230) -> (x >= y?=w1236:bool)
                    n717 = case shown="True" w1236 {
                      tunnel: w1231 -> [w1246 _]
                      tunnel: w1229 -> [w1245 _]
                      tunnel: w1228 -> [w1244 _]
                      tunnel: w1227 -> [w1243 _]
                      frame True {
                        n718 = stacked-sequence {
                          tunnel: w1246 -> [w1250 _]
                          tunnel: w1245 -> [w1248 _]
                          tunnel: w1244 -> [_ w1256]
                          tunnel: w1243 -> [w1247 _]
                          frame #0 {
                            n719 = Build Array(w1248) -> (w1251:string[])
                            n720 = Build Array(w1250) -> (w1249:dbl[])
                            n721 = TDMS Write(0:w1247, 5:"TEST PASS", 7:w1251, 9:w1249) -> (15:w1253:errorcluster)  [unwired: 2 in, 3 out]
                            n722 = local write "data file error"(w1253) -> ()
                          }
                          frame #1 {
                            n723 = Bundle(cluster=w1256, "STATUS"="CYCLE PASS") -> (w1254:T4)  [unwired: 2 in]
                            n724 = local write "LAB02-2 (RESULT)"(TRUE) -> ()
                            n725 = local write "LAB02-2 (DISP)"(w1254) -> ()
                          }
                        }
                      }
                      frame False {
                      }
                    }
                  }
                }
              }
              frame #4 {
                # "LAB03-1"
                n726 = Less?(x=w1258, y=2) -> (x < y?=w1261:bool)
                n727 = local read "LAB03-1 (DISP)"() -> (w1263:T4)
                n728 = Unbundle(w1263) -> ("STATUS"=w1264:string)  [unwired: 2 out]
                n729 = Equal?(x=w1264, y="RUN") -> (x = y?=w1260:bool)
                n730 = And(x=w1260, y=w1261) -> (x .and. y?=w1259:bool)
                n731 = case shown="True" w1259 {
                  tunnel: w1263 -> [_ w1267]
                  tunnel: w1258 -> [_ w1272]
                  frame False {
                  }
                  frame True {
                    n732 = local read "LAB03-1 (SET)"() -> (w1274:T5)
                    n733 = local read "LAB03-1 (TDMS)"() -> (w1266:refnum<k34>)
                    n734 = Unbundle(w1267) -> ("CYCLE"=w1273:dbl)  [unwired: 2 out]
                    n735 = Unbundle(w1274) -> ("CYCLES"=w1269:dbl, "T-RISE mins"=w1271:dbl)  [unwired: 3 out]
                    n736 = case shown="\"TEST SET UP\", Default" w1272 {
                      tunnel: w1271 -> [_ _ w1281]
                      tunnel: [w1276 w1278 w1281] -> w1270
                      tunnel: w1269 -> [w1276 w1278 _]
                      tunnel: ["TEST SET UP CYCLES" "CYCLES" "T-RISE TEST"] -> w1268
                      frame "TEST SET UP", Default {
                      }
                      frame "CYCLE TEST" {
                      }
                      frame "T-RISE TEST" {
                      }
                    }
                    n737 = Greater Or Equal?(x=w1273, y=w1269) -> (x >= y?=w1275:bool)
                    n738 = case shown="True" w1275 {
                      tunnel: w1270 -> [w1285 _]
                      tunnel: w1268 -> [w1284 _]
                      tunnel: w1267 -> [w1283 _]
                      tunnel: w1266 -> [w1282 _]
                      frame True {
                        n739 = stacked-sequence {
                          tunnel: w1285 -> [w1289 _]
                          tunnel: w1284 -> [w1287 _]
                          tunnel: w1283 -> [_ w1295]
                          tunnel: w1282 -> [w1286 _]
                          frame #0 {
                            n740 = Build Array(w1287) -> (w1290:string[])
                            n741 = Build Array(w1289) -> (w1288:dbl[])
                            n742 = TDMS Write(0:w1286, 5:"TEST PASS", 7:w1290, 9:w1288) -> (15:w1292:errorcluster)  [unwired: 2 in, 3 out]
                            n743 = local write "data file error"(w1292) -> ()
                          }
                          frame #1 {
                            n744 = Bundle(cluster=w1295, "STATUS"="CYCLE PASS") -> (w1293:T4)  [unwired: 2 in]
                            n745 = local write "LAB03-1 (RESULT)"(TRUE) -> ()
                            n746 = local write "LAB03-1 (DISP)"(w1293) -> ()
                          }
                        }
                      }
                      frame False {
                      }
                    }
                  }
                }
              }
              frame #5 {
                # "LAB03-2"
                n747 = Less?(x=w1297, y=2) -> (x < y?=w1300:bool)
                n748 = local read "LAB03-2 (DISP)"() -> (w1302:T4)
                n749 = Unbundle(w1302) -> ("STATUS"=w1303:string)  [unwired: 2 out]
                n750 = Equal?(x=w1303, y="RUN") -> (x = y?=w1299:bool)
                n751 = And(x=w1299, y=w1300) -> (x .and. y?=w1298:bool)
                n752 = case shown="True" w1298 {
                  tunnel: w1302 -> [_ w1306]
                  tunnel: w1297 -> [_ w1311]
                  frame False {
                  }
                  frame True {
                    n753 = local read "LAB03-2 (SET)"() -> (w1313:T5)
                    n754 = local read "LAB03-2 (TDMS)"() -> (w1305:refnum<k34>)
                    n755 = Unbundle(w1306) -> ("CYCLE"=w1312:dbl)  [unwired: 2 out]
                    n756 = Unbundle(w1313) -> ("CYCLES"=w1308:dbl, "T-RISE mins"=w1310:dbl)  [unwired: 3 out]
                    n757 = case shown="\"TEST SET UP\", Default" w1311 {
                      tunnel: w1310 -> [_ _ w1320]
                      tunnel: [w1315 w1317 w1320] -> w1309
                      tunnel: w1308 -> [w1315 w1317 _]
                      tunnel: ["TEST SET UP CYCLES" "CYCLES" "T-RISE TEST"] -> w1307
                      frame "TEST SET UP", Default {
                      }
                      frame "CYCLE TEST" {
                      }
                      frame "T-RISE TEST" {
                      }
                    }
                    n758 = Greater Or Equal?(x=w1312, y=w1308) -> (x >= y?=w1314:bool)
                    n759 = case shown="True" w1314 {
                      tunnel: w1309 -> [w1324 _]
                      tunnel: w1307 -> [w1323 _]
                      tunnel: w1306 -> [w1322 _]
                      tunnel: w1305 -> [w1321 _]
                      frame True {
                        n760 = stacked-sequence {
                          tunnel: w1324 -> [w1328 _]
                          tunnel: w1323 -> [w1326 _]
                          tunnel: w1322 -> [_ w1334]
                          tunnel: w1321 -> [w1325 _]
                          frame #0 {
                            n761 = Build Array(w1326) -> (w1329:string[])
                            n762 = Build Array(w1328) -> (w1327:dbl[])
                            n763 = TDMS Write(0:w1325, 5:"TEST PASS", 7:w1329, 9:w1327) -> (15:w1331:errorcluster)  [unwired: 2 in, 3 out]
                            n764 = local write "data file error"(w1331) -> ()
                          }
                          frame #1 {
                            n765 = Bundle(cluster=w1334, "STATUS"="CYCLE PASS") -> (w1332:T4)  [unwired: 2 in]
                            n766 = local write "LAB03-2 (RESULT)"(TRUE) -> ()
                            n767 = local write "LAB03-2 (DISP)"(w1332) -> ()
                          }
                        }
                      }
                      frame False {
                      }
                    }
                  }
                }
              }
              frame #6 {
                # "LAB04-1"
                n768 = Less?(x=w1336, y=2) -> (x < y?=w1339:bool)
                n769 = local read "LAB04-1 (DISP)"() -> (w1341:T4)
                n770 = Unbundle(w1341) -> ("STATUS"=w1342:string)  [unwired: 2 out]
                n771 = Equal?(x=w1342, y="RUN") -> (x = y?=w1338:bool)
                n772 = And(x=w1338, y=w1339) -> (x .and. y?=w1337:bool)
                n773 = case shown="True" w1337 {
                  tunnel: w1341 -> [_ w1345]
                  tunnel: w1336 -> [_ w1350]
                  frame False {
                  }
                  frame True {
                    n774 = local read "LAB04-1 (SET)"() -> (w1352:T5)
                    n775 = local read "LAB04-1 (TDMS)"() -> (w1344:refnum<k34>)
                    n776 = Unbundle(w1345) -> ("CYCLE"=w1351:dbl)  [unwired: 2 out]
                    n777 = Unbundle(w1352) -> ("CYCLES"=w1347:dbl, "T-RISE mins"=w1349:dbl)  [unwired: 3 out]
                    n778 = case shown="\"TEST SET UP\", Default" w1350 {
                      tunnel: w1349 -> [_ _ w1359]
                      tunnel: [w1354 w1356 w1359] -> w1348
                      tunnel: w1347 -> [w1354 w1356 _]
                      tunnel: ["TEST SET UP CYCLES" "CYCLES" "T-RISE TEST"] -> w1346
                      frame "TEST SET UP", Default {
                      }
                      frame "CYCLE TEST" {
                      }
                      frame "T-RISE TEST" {
                      }
                    }
                    n779 = Greater Or Equal?(x=w1351, y=w1347) -> (x >= y?=w1353:bool)
                    n780 = case shown="True" w1353 {
                      tunnel: w1348 -> [w1363 _]
                      tunnel: w1346 -> [w1362 _]
                      tunnel: w1345 -> [w1361 _]
                      tunnel: w1344 -> [w1360 _]
                      frame True {
                        n781 = stacked-sequence {
                          tunnel: w1363 -> [w1367 _]
                          tunnel: w1362 -> [w1365 _]
                          tunnel: w1361 -> [_ w1373]
                          tunnel: w1360 -> [w1364 _]
                          frame #0 {
                            n782 = Build Array(w1365) -> (w1368:string[])
                            n783 = Build Array(w1367) -> (w1366:dbl[])
                            n784 = TDMS Write(0:w1364, 5:"TEST PASS", 7:w1368, 9:w1366) -> (15:w1370:errorcluster)  [unwired: 2 in, 3 out]
                            n785 = local write "data file error"(w1370) -> ()
                          }
                          frame #1 {
                            n786 = Bundle(cluster=w1373, "STATUS"="CYCLE PASS") -> (w1371:T4)  [unwired: 2 in]
                            n787 = local write "LAB04-1 (RESULT)"(TRUE) -> ()
                            n788 = local write "LAB04-1 (DISP)"(w1371) -> ()
                          }
                        }
                      }
                      frame False {
                      }
                    }
                  }
                }
              }
              frame #7 {
                # "LAB04-2"
                n789 = Less?(x=w1375, y=2) -> (x < y?=w1378:bool)
                n790 = local read "LAB04-2 (DISP)"() -> (w1380:T4)
                n791 = Unbundle(w1380) -> ("STATUS"=w1381:string)  [unwired: 2 out]
                n792 = Equal?(x=w1381, y="RUN") -> (x = y?=w1377:bool)
                n793 = And(x=w1377, y=w1378) -> (x .and. y?=w1376:bool)
                n794 = case shown="True" w1376 {
                  tunnel: w1380 -> [_ w1384]
                  tunnel: w1375 -> [_ w1389]
                  frame False {
                  }
                  frame True {
                    n795 = local read "LAB04-2 (SET)"() -> (w1391:T5)
                    n796 = local read "LAB04-2 (TDMS)"() -> (w1383:refnum<k34>)
                    n797 = Unbundle(w1384) -> ("CYCLE"=w1390:dbl)  [unwired: 2 out]
                    n798 = Unbundle(w1391) -> ("CYCLES"=w1386:dbl, "T-RISE mins"=w1388:dbl)  [unwired: 3 out]
                    n799 = case shown="\"TEST SET UP\", Default" w1389 {
                      tunnel: w1388 -> [_ _ w1398]
                      tunnel: [w1393 w1395 w1398] -> w1387
                      tunnel: w1386 -> [w1393 w1395 _]
                      tunnel: ["TEST SET UP CYCLES" "CYCLES" "T-RISE TEST"] -> w1385
                      frame "TEST SET UP", Default {
                      }
                      frame "CYCLE TEST" {
                      }
                      frame "T-RISE TEST" {
                      }
                    }
                    n800 = Greater Or Equal?(x=w1390, y=w1386) -> (x >= y?=w1392:bool)
                    n801 = case shown="True" w1392 {
                      tunnel: w1387 -> [w1402 _]
                      tunnel: w1385 -> [w1401 _]
                      tunnel: w1384 -> [w1400 _]
                      tunnel: w1383 -> [w1399 _]
                      frame True {
                        n802 = stacked-sequence {
                          tunnel: w1402 -> [w1406 _]
                          tunnel: w1401 -> [w1404 _]
                          tunnel: w1400 -> [_ w1412]
                          tunnel: w1399 -> [w1403 _]
                          frame #0 {
                            n803 = Build Array(w1404) -> (w1407:string[])
                            n804 = Build Array(w1406) -> (w1405:dbl[])
                            n805 = TDMS Write(0:w1403, 5:"TEST PASS", 7:w1407, 9:w1405) -> (15:w1409:errorcluster)  [unwired: 2 in, 3 out]
                            n806 = local write "data file error"(w1409) -> ()
                          }
                          frame #1 {
                            n807 = Bundle(cluster=w1412, "STATUS"="CYCLE PASS") -> (w1410:T4)  [unwired: 2 in]
                            n808 = local write "LAB04-2 (RESULT)"(TRUE) -> ()
                            n809 = local write "LAB04-2 (DISP)"(w1410) -> ()
                          }
                        }
                      }
                      frame False {
                      }
                    }
                  }
                }
              }
              frame #8 {
                # "LAB05-1"
                n810 = Less?(x=w1414, y=2) -> (x < y?=w1417:bool)
                n811 = local read "LAB05-1 (DISP)"() -> (w1419:T4)
                n812 = Unbundle(w1419) -> ("STATUS"=w1420:string)  [unwired: 2 out]
                n813 = Equal?(x=w1420, y="RUN") -> (x = y?=w1416:bool)
                n814 = And(x=w1416, y=w1417) -> (x .and. y?=w1415:bool)
                n815 = case shown="True" w1415 {
                  tunnel: w1419 -> [_ w1423]
                  tunnel: w1414 -> [_ w1428]
                  frame False {
                  }
                  frame True {
                    n816 = local read "LAB05-1 (SET)"() -> (w1430:T5)
                    n817 = local read "LAB05-1 (TDMS)"() -> (w1422:refnum<k34>)
                    n818 = Unbundle(w1423) -> ("CYCLE"=w1429:dbl)  [unwired: 2 out]
                    n819 = Unbundle(w1430) -> ("CYCLES"=w1425:dbl, "T-RISE mins"=w1427:dbl)  [unwired: 3 out]
                    n820 = case shown="\"TEST SET UP\", Default" w1428 {
                      tunnel: w1427 -> [_ _ w1437]
                      tunnel: [w1432 w1434 w1437] -> w1426
                      tunnel: w1425 -> [w1432 w1434 _]
                      tunnel: ["TEST SET UP CYCLES" "CYCLES" "T-RISE TEST"] -> w1424
                      frame "TEST SET UP", Default {
                      }
                      frame "CYCLE TEST" {
                      }
                      frame "T-RISE TEST" {
                      }
                    }
                    n821 = Greater Or Equal?(x=w1429, y=w1425) -> (x >= y?=w1431:bool)
                    n822 = case shown="True" w1431 {
                      tunnel: w1426 -> [w1441 _]
                      tunnel: w1424 -> [w1440 _]
                      tunnel: w1423 -> [w1439 _]
                      tunnel: w1422 -> [w1438 _]
                      frame True {
                        n823 = stacked-sequence {
                          tunnel: w1441 -> [w1445 _]
                          tunnel: w1440 -> [w1443 _]
                          tunnel: w1439 -> [_ w1451]
                          tunnel: w1438 -> [w1442 _]
                          frame #0 {
                            n824 = Build Array(w1443) -> (w1446:string[])
                            n825 = Build Array(w1445) -> (w1444:dbl[])
                            n826 = TDMS Write(0:w1442, 5:"TEST PASS", 7:w1446, 9:w1444) -> (15:w1448:errorcluster)  [unwired: 2 in, 3 out]
                            n827 = local write "data file error"(w1448) -> ()
                          }
                          frame #1 {
                            n828 = Bundle(cluster=w1451, "STATUS"="CYCLE PASS") -> (w1449:T4)  [unwired: 2 in]
                            n829 = local write "LAB05-1 (RESULT)"(TRUE) -> ()
                            n830 = local write "LAB05-1 (DISP)"(w1449) -> ()
                          }
                        }
                      }
                      frame False {
                      }
                    }
                  }
                }
              }
              frame #9 {
                # "LAB05-2"
                n831 = Less?(x=w1453, y=2) -> (x < y?=w1456:bool)
                n832 = local read "LAB05-2 (DISP)"() -> (w1458:T4)
                n833 = Unbundle(w1458) -> ("STATUS"=w1459:string)  [unwired: 2 out]
                n834 = Equal?(x=w1459, y="RUN") -> (x = y?=w1455:bool)
                n835 = And(x=w1455, y=w1456) -> (x .and. y?=w1454:bool)
                n836 = case shown="True" w1454 {
                  tunnel: w1458 -> [_ w1462]
                  tunnel: w1453 -> [_ w1467]
                  frame False {
                  }
                  frame True {
                    n837 = local read "LAB05-2 (SET)"() -> (w1469:T5)
                    n838 = local read "LAB05-1 (TDMS)"() -> (w1461:refnum<k34>)
                    n839 = Unbundle(w1462) -> ("CYCLE"=w1468:dbl)  [unwired: 2 out]
                    n840 = Unbundle(w1469) -> ("CYCLES"=w1464:dbl, "T-RISE mins"=w1466:dbl)  [unwired: 3 out]
                    n841 = case shown="\"TEST SET UP\", Default" w1467 {
                      tunnel: w1466 -> [_ _ w1476]
                      tunnel: [w1471 w1473 w1476] -> w1465
                      tunnel: w1464 -> [w1471 w1473 _]
                      tunnel: ["TEST SET UP CYCLES" "CYCLES" "T-RISE TEST"] -> w1463
                      frame "TEST SET UP", Default {
                      }
                      frame "CYCLE TEST" {
                      }
                      frame "T-RISE TEST" {
                      }
                    }
                    n842 = Greater Or Equal?(x=w1468, y=w1464) -> (x >= y?=w1470:bool)
                    n843 = case shown="True" w1470 {
                      tunnel: w1465 -> [w1480 _]
                      tunnel: w1463 -> [w1479 _]
                      tunnel: w1462 -> [w1478 _]
                      tunnel: w1461 -> [w1477 _]
                      frame True {
                        n844 = stacked-sequence {
                          tunnel: w1480 -> [w1484 _]
                          tunnel: w1479 -> [w1482 _]
                          tunnel: w1478 -> [_ w1490]
                          tunnel: w1477 -> [w1481 _]
                          frame #0 {
                            n845 = Build Array(w1482) -> (w1485:string[])
                            n846 = Build Array(w1484) -> (w1483:dbl[])
                            n847 = TDMS Write(0:w1481, 5:"TEST PASS", 7:w1485, 9:w1483) -> (15:w1487:errorcluster)  [unwired: 2 in, 3 out]
                            n848 = local write "data file error"(w1487) -> ()
                          }
                          frame #1 {
                            n849 = Bundle(cluster=w1490, "STATUS"="CYCLE PASS") -> (w1488:T4)  [unwired: 2 in]
                            n850 = local write "LAB05-2 (RESULT)"(TRUE) -> ()
                            n851 = local write "LAB05-2 (DISP)"(w1488) -> ()
                          }
                        }
                      }
                      frame False {
                      }
                    }
                  }
                }
              }
            }
          }
          frame #5 {
            # "check if test cycles reached for temperature rise test"
            n852 = stacked-sequence {
              tunnel: w1512 -> [_ _ _ _ _ _ _ _ _ _]
              tunnel: w1511 -> [_ _ _ _ _ _ _ _ _ _]
              tunnel: w1510 -> [_ _ _ _ _ _ _ _ _ _]
              tunnel: w1509 -> [_ _ _ _ _ _ _ _ _ _]
              tunnel: w1508 -> [_ _ _ _ _ _ _ _ _ _]
              tunnel: w1507 -> [_ _ _ _ _ _ _ _ _ _]
              tunnel: w1506 -> [_ _ _ _ _ _ _ _ _ _]
              tunnel: w1505 -> [_ _ _ _ _ _ _ _ _ _]
              tunnel: w1504 -> [_ _ _ _ _ _ _ _ _ _]
              tunnel: w1503 -> [_ _ _ _ _ _ _ _ _ _]
              tunnel: w1502 -> [w1518 _ _ _ _ _ _ _ _ _]
              tunnel: w1501 -> [w1513 w1544 w1574 w1604 w1634 w1664 w1694 w1724 w1754 w1784]
              tunnel: w1500 -> [_ w1543 _ _ _ _ _ _ _ _]
              tunnel: w1499 -> [_ _ w1573 _ _ _ _ _ _ _]
              tunnel: w1498 -> [_ _ _ w1603 _ _ _ _ _ _]
              tunnel: w1497 -> [_ _ _ _ w1633 _ _ _ _ _]
              tunnel: w1496 -> [_ _ _ _ _ w1663 _ _ _ _]
              tunnel: w1495 -> [_ _ _ _ _ _ w1693 _ _ _]
              tunnel: w1494 -> [_ _ _ _ _ _ _ w1723 _ _]
              tunnel: w1493 -> [_ _ _ _ _ _ _ _ w1753 _]
              tunnel: w1492 -> [_ _ _ _ _ _ _ _ _ w1783]
              frame #0 {
                # "LAB01-1"
                n853 = Equal?(x=w1518, y=2) -> (x = y?=w1516:bool)
                n854 = local read "LAB01-1 (DISP)"() -> (w1519:T4)
                n855 = Unbundle(w1519) -> ("STATUS"=w1520:string)  [unwired: 2 out]
                n856 = Equal?(x=w1520, y="RUN") -> (x = y?=w1515:bool)
                n857 = And(x=w1515, y=w1516) -> (x .and. y?=w1514:bool)
                n858 = case shown="True" w1514 {
                  tunnel: w1519 -> [_ w1523]
                  tunnel: w1513 -> [_ w1526]
                  frame False {
                  }
                  frame True {
                    n859 = local read "LAB01-1 (SET)"() -> (w1525:T5)
                    n860 = local read "LAB01-1 (TDMS)"() -> (w1522:refnum<k34>)
                    n861 = Unbundle(w1523) -> ("CYCLE"=w1527:dbl)  [unwired: 2 out]
                    n862 = Unbundle(w1525) -> ("T-RISE mins"=w1524:dbl)  [unwired: 4 out]
                    n863 = Greater Or Equal?(x=w1527, y=w1526) -> (x >= y?=w1528:bool)
                    n864 = case shown="True" w1528 {
                      tunnel: w1524 -> [w1531 _]
                      tunnel: w1523 -> [w1530 _]
                      tunnel: w1522 -> [w1529 _]
                      frame True {
                        n865 = stacked-sequence {
                          tunnel: w1531 -> [w1534 _]
                          tunnel: w1530 -> [_ w1539]
                          tunnel: w1529 -> [w1532 _]
                          frame #0 {
                            n866 = Build Array("T-RISE") -> (w1536:string[])
                            n867 = Build Array(w1534) -> (w1535:dbl[])
                            n868 = TDMS Write(0:w1532, 5:"TEST PASS", 7:w1536, 9:w1535) -> (15:w1538:errorcluster)  [unwired: 2 in, 3 out]
                            n869 = local write "data file error"(w1538) -> ()
                          }
                          frame #1 {
                            n870 = Bundle(cluster=w1539, "STATUS"="T-RISE PASS") -> (w1541:T4)  [unwired: 2 in]
                            n871 = local write "LAB01-1 (RESULT)"(TRUE) -> ()
                            n872 = local write "LAB01-1 (DISP)"(w1541) -> ()
                          }
                        }
                      }
                      frame False {
                      }
                    }
                  }
                }
              }
              frame #1 {
                # "LAB01-2"
                n873 = Equal?(x=w1543, y=2) -> (x = y?=w1547:bool)
                n874 = local read "LAB01-2 (DISP)"() -> (w1549:T4)
                n875 = Unbundle(w1549) -> ("STATUS"=w1550:string)  [unwired: 2 out]
                n876 = Equal?(x=w1550, y="RUN") -> (x = y?=w1546:bool)
                n877 = And(x=w1546, y=w1547) -> (x .and. y?=w1545:bool)
                n878 = case shown="True" w1545 {
                  tunnel: w1549 -> [_ w1553]
                  tunnel: w1544 -> [_ w1556]
                  frame False {
                  }
                  frame True {
                    n879 = local read "LAB01-2 (SET)"() -> (w1555:T5)
                    n880 = local read "LAB01-2 (TDMS)"() -> (w1552:refnum<k34>)
                    n881 = Unbundle(w1553) -> ("CYCLE"=w1557:dbl)  [unwired: 2 out]
                    n882 = Unbundle(w1555) -> ("T-RISE mins"=w1554:dbl)  [unwired: 4 out]
                    n883 = Greater Or Equal?(x=w1557, y=w1556) -> (x >= y?=w1558:bool)
                    n884 = case shown="True" w1558 {
                      tunnel: w1554 -> [w1561 _]
                      tunnel: w1553 -> [w1560 _]
                      tunnel: w1552 -> [w1559 _]
                      frame True {
                        n885 = stacked-sequence {
                          tunnel: w1561 -> [w1564 _]
                          tunnel: w1560 -> [_ w1569]
                          tunnel: w1559 -> [w1562 _]
                          frame #0 {
                            n886 = Build Array("T-RISE") -> (w1566:string[])
                            n887 = Build Array(w1564) -> (w1565:dbl[])
                            n888 = TDMS Write(0:w1562, 5:"TEST PASS", 7:w1566, 9:w1565) -> (15:w1568:errorcluster)  [unwired: 2 in, 3 out]
                            n889 = local write "data file error"(w1568) -> ()
                          }
                          frame #1 {
                            n890 = Bundle(cluster=w1569, "STATUS"="T-RISE PASS") -> (w1571:T4)  [unwired: 2 in]
                            n891 = local write "LAB01-2 (RESULT)"(TRUE) -> ()
                            n892 = local write "LAB01-2 (DISP)"(w1571) -> ()
                          }
                        }
                      }
                      frame False {
                      }
                    }
                  }
                }
              }
              frame #2 {
                # "LAB02-1"
                n893 = Equal?(x=w1573, y=2) -> (x = y?=w1577:bool)
                n894 = local read "LAB02-1 (DISP)"() -> (w1579:T4)
                n895 = Unbundle(w1579) -> ("STATUS"=w1580:string)  [unwired: 2 out]
                n896 = Equal?(x=w1580, y="RUN") -> (x = y?=w1576:bool)
                n897 = And(x=w1576, y=w1577) -> (x .and. y?=w1575:bool)
                n898 = case shown="True" w1575 {
                  tunnel: w1579 -> [_ w1583]
                  tunnel: w1574 -> [_ w1586]
                  frame False {
                  }
                  frame True {
                    n899 = local read "LAB02-1 (SET)"() -> (w1585:T5)
                    n900 = local read "LAB02-1 (TDMS)"() -> (w1582:refnum<k34>)
                    n901 = Unbundle(w1583) -> ("CYCLE"=w1587:dbl)  [unwired: 2 out]
                    n902 = Unbundle(w1585) -> ("T-RISE mins"=w1584:dbl)  [unwired: 4 out]
                    n903 = Greater Or Equal?(x=w1587, y=w1586) -> (x >= y?=w1588:bool)
                    n904 = case shown="True" w1588 {
                      tunnel: w1584 -> [w1591 _]
                      tunnel: w1583 -> [w1590 _]
                      tunnel: w1582 -> [w1589 _]
                      frame True {
                        n905 = stacked-sequence {
                          tunnel: w1591 -> [w1594 _]
                          tunnel: w1590 -> [_ w1599]
                          tunnel: w1589 -> [w1592 _]
                          frame #0 {
                            n906 = Build Array("T-RISE") -> (w1596:string[])
                            n907 = Build Array(w1594) -> (w1595:dbl[])
                            n908 = TDMS Write(0:w1592, 5:"TEST PASS", 7:w1596, 9:w1595) -> (15:w1598:errorcluster)  [unwired: 2 in, 3 out]
                            n909 = local write "data file error"(w1598) -> ()
                          }
                          frame #1 {
                            n910 = Bundle(cluster=w1599, "STATUS"="T-RISE PASS") -> (w1601:T4)  [unwired: 2 in]
                            n911 = local write "LAB02-1 (RESULT)"(TRUE) -> ()
                            n912 = local write "LAB02-1 (DISP)"(w1601) -> ()
                          }
                        }
                      }
                      frame False {
                      }
                    }
                  }
                }
              }
              frame #3 {
                # "LAB02-2"
                n913 = Equal?(x=w1603, y=2) -> (x = y?=w1607:bool)
                n914 = local read "LAB02-2 (DISP)"() -> (w1609:T4)
                n915 = Unbundle(w1609) -> ("STATUS"=w1610:string)  [unwired: 2 out]
                n916 = Equal?(x=w1610, y="RUN") -> (x = y?=w1606:bool)
                n917 = And(x=w1606, y=w1607) -> (x .and. y?=w1605:bool)
                n918 = case shown="True" w1605 {
                  tunnel: w1609 -> [_ w1613]
                  tunnel: w1604 -> [_ w1616]
                  frame False {
                  }
                  frame True {
                    n919 = local read "LAB02-2 (SET)"() -> (w1615:T5)
                    n920 = local read "LAB02-2 (TDMS)"() -> (w1612:refnum<k34>)
                    n921 = Unbundle(w1613) -> ("CYCLE"=w1617:dbl)  [unwired: 2 out]
                    n922 = Unbundle(w1615) -> ("T-RISE mins"=w1614:dbl)  [unwired: 4 out]
                    n923 = Greater Or Equal?(x=w1617, y=w1616) -> (x >= y?=w1618:bool)
                    n924 = case shown="True" w1618 {
                      tunnel: w1614 -> [w1621 _]
                      tunnel: w1613 -> [w1620 _]
                      tunnel: w1612 -> [w1619 _]
                      frame True {
                        n925 = stacked-sequence {
                          tunnel: w1621 -> [w1624 _]
                          tunnel: w1620 -> [_ w1629]
                          tunnel: w1619 -> [w1622 _]
                          frame #0 {
                            n926 = Build Array("T-RISE") -> (w1626:string[])
                            n927 = Build Array(w1624) -> (w1625:dbl[])
                            n928 = TDMS Write(0:w1622, 5:"TEST PASS", 7:w1626, 9:w1625) -> (15:w1628:errorcluster)  [unwired: 2 in, 3 out]
                            n929 = local write "data file error"(w1628) -> ()
                          }
                          frame #1 {
                            n930 = Bundle(cluster=w1629, "STATUS"="T-RISE PASS") -> (w1631:T4)  [unwired: 2 in]
                            n931 = local write "LAB02-2 (RESULT)"(TRUE) -> ()
                            n932 = local write "LAB02-2 (DISP)"(w1631) -> ()
                          }
                        }
                      }
                      frame False {
                      }
                    }
                  }
                }
              }
              frame #4 {
                # "LAB03-1"
                n933 = Equal?(x=w1633, y=2) -> (x = y?=w1637:bool)
                n934 = local read "LAB03-1 (DISP)"() -> (w1639:T4)
                n935 = Unbundle(w1639) -> ("STATUS"=w1640:string)  [unwired: 2 out]
                n936 = Equal?(x=w1640, y="RUN") -> (x = y?=w1636:bool)
                n937 = And(x=w1636, y=w1637) -> (x .and. y?=w1635:bool)
                n938 = case shown="True" w1635 {
                  tunnel: w1639 -> [_ w1643]
                  tunnel: w1634 -> [_ w1646]
                  frame False {
                  }
                  frame True {
                    n939 = local read "LAB03-1 (SET)"() -> (w1645:T5)
                    n940 = local read "LAB03-1 (TDMS)"() -> (w1642:refnum<k34>)
                    n941 = Unbundle(w1643) -> ("CYCLE"=w1647:dbl)  [unwired: 2 out]
                    n942 = Unbundle(w1645) -> ("T-RISE mins"=w1644:dbl)  [unwired: 4 out]
                    n943 = Greater Or Equal?(x=w1647, y=w1646) -> (x >= y?=w1648:bool)
                    n944 = case shown="True" w1648 {
                      tunnel: w1644 -> [w1651 _]
                      tunnel: w1643 -> [w1650 _]
                      tunnel: w1642 -> [w1649 _]
                      frame True {
                        n945 = stacked-sequence {
                          tunnel: w1651 -> [w1654 _]
                          tunnel: w1650 -> [_ w1659]
                          tunnel: w1649 -> [w1652 _]
                          frame #0 {
                            n946 = Build Array("T-RISE") -> (w1656:string[])
                            n947 = Build Array(w1654) -> (w1655:dbl[])
                            n948 = TDMS Write(0:w1652, 5:"TEST PASS", 7:w1656, 9:w1655) -> (15:w1658:errorcluster)  [unwired: 2 in, 3 out]
                            n949 = local write "data file error"(w1658) -> ()
                          }
                          frame #1 {
                            n950 = Bundle(cluster=w1659, "STATUS"="T-RISE PASS") -> (w1661:T4)  [unwired: 2 in]
                            n951 = local write "LAB03-1 (RESULT)"(TRUE) -> ()
                            n952 = local write "LAB03-1 (DISP)"(w1661) -> ()
                          }
                        }
                      }
                      frame False {
                      }
                    }
                  }
                }
              }
              frame #5 {
                # "LAB03-2"
                n953 = Equal?(x=w1663, y=2) -> (x = y?=w1667:bool)
                n954 = local read "LAB03-2 (DISP)"() -> (w1669:T4)
                n955 = Unbundle(w1669) -> ("STATUS"=w1670:string)  [unwired: 2 out]
                n956 = Equal?(x=w1670, y="RUN") -> (x = y?=w1666:bool)
                n957 = And(x=w1666, y=w1667) -> (x .and. y?=w1665:bool)
                n958 = case shown="True" w1665 {
                  tunnel: w1669 -> [_ w1673]
                  tunnel: w1664 -> [_ w1676]
                  frame False {
                  }
                  frame True {
                    n959 = local read "LAB03-2 (SET)"() -> (w1675:T5)
                    n960 = local read "LAB03-2 (TDMS)"() -> (w1672:refnum<k34>)
                    n961 = Unbundle(w1673) -> ("CYCLE"=w1677:dbl)  [unwired: 2 out]
                    n962 = Unbundle(w1675) -> ("T-RISE mins"=w1674:dbl)  [unwired: 4 out]
                    n963 = Greater Or Equal?(x=w1677, y=w1676) -> (x >= y?=w1678:bool)
                    n964 = case shown="True" w1678 {
                      tunnel: w1674 -> [w1681 _]
                      tunnel: w1673 -> [w1680 _]
                      tunnel: w1672 -> [w1679 _]
                      frame True {
                        n965 = stacked-sequence {
                          tunnel: w1681 -> [w1684 _]
                          tunnel: w1680 -> [_ w1689]
                          tunnel: w1679 -> [w1682 _]
                          frame #0 {
                            n966 = Build Array("T-RISE") -> (w1686:string[])
                            n967 = Build Array(w1684) -> (w1685:dbl[])
                            n968 = TDMS Write(0:w1682, 5:"TEST PASS", 7:w1686, 9:w1685) -> (15:w1688:errorcluster)  [unwired: 2 in, 3 out]
                            n969 = local write "data file error"(w1688) -> ()
                          }
                          frame #1 {
                            n970 = Bundle(cluster=w1689, "STATUS"="T-RISE PASS") -> (w1691:T4)  [unwired: 2 in]
                            n971 = local write "LAB03-2 (RESULT)"(TRUE) -> ()
                            n972 = local write "LAB03-2 (DISP)"(w1691) -> ()
                          }
                        }
                      }
                      frame False {
                      }
                    }
                  }
                }
              }
              frame #6 {
                # "LAB04-1"
                n973 = Equal?(x=w1693, y=2) -> (x = y?=w1697:bool)
                n974 = local read "LAB04-1 (DISP)"() -> (w1699:T4)
                n975 = Unbundle(w1699) -> ("STATUS"=w1700:string)  [unwired: 2 out]
                n976 = Equal?(x=w1700, y="RUN") -> (x = y?=w1696:bool)
                n977 = And(x=w1696, y=w1697) -> (x .and. y?=w1695:bool)
                n978 = case shown="True" w1695 {
                  tunnel: w1699 -> [_ w1703]
                  tunnel: w1694 -> [_ w1706]
                  frame False {
                  }
                  frame True {
                    n979 = local read "LAB04-1 (SET)"() -> (w1705:T5)
                    n980 = local read "LAB04-1 (TDMS)"() -> (w1702:refnum<k34>)
                    n981 = Unbundle(w1703) -> ("CYCLE"=w1707:dbl)  [unwired: 2 out]
                    n982 = Unbundle(w1705) -> ("T-RISE mins"=w1704:dbl)  [unwired: 4 out]
                    n983 = Greater Or Equal?(x=w1707, y=w1706) -> (x >= y?=w1708:bool)
                    n984 = case shown="True" w1708 {
                      tunnel: w1704 -> [w1711 _]
                      tunnel: w1703 -> [w1710 _]
                      tunnel: w1702 -> [w1709 _]
                      frame True {
                        n985 = stacked-sequence {
                          tunnel: w1711 -> [w1714 _]
                          tunnel: w1710 -> [_ w1719]
                          tunnel: w1709 -> [w1712 _]
                          frame #0 {
                            n986 = Build Array("T-RISE") -> (w1716:string[])
                            n987 = Build Array(w1714) -> (w1715:dbl[])
                            n988 = TDMS Write(0:w1712, 5:"TEST PASS", 7:w1716, 9:w1715) -> (15:w1718:errorcluster)  [unwired: 2 in, 3 out]
                            n989 = local write "data file error"(w1718) -> ()
                          }
                          frame #1 {
                            n990 = Bundle(cluster=w1719, "STATUS"="T-RISE PASS") -> (w1721:T4)  [unwired: 2 in]
                            n991 = local write "LAB04-1 (RESULT)"(TRUE) -> ()
                            n992 = local write "LAB04-1 (DISP)"(w1721) -> ()
                          }
                        }
                      }
                      frame False {
                      }
                    }
                  }
                }
              }
              frame #7 {
                # "LAB04-2"
                n993 = Equal?(x=w1723, y=2) -> (x = y?=w1727:bool)
                n994 = local read "LAB04-2 (DISP)"() -> (w1729:T4)
                n995 = Unbundle(w1729) -> ("STATUS"=w1730:string)  [unwired: 2 out]
                n996 = Equal?(x=w1730, y="RUN") -> (x = y?=w1726:bool)
                n997 = And(x=w1726, y=w1727) -> (x .and. y?=w1725:bool)
                n998 = case shown="True" w1725 {
                  tunnel: w1729 -> [_ w1733]
                  tunnel: w1724 -> [_ w1736]
                  frame False {
                  }
                  frame True {
                    n999 = local read "LAB04-2 (SET)"() -> (w1735:T5)
                    n1000 = local read "LAB04-2 (TDMS)"() -> (w1732:refnum<k34>)
                    n1001 = Unbundle(w1733) -> ("CYCLE"=w1737:dbl)  [unwired: 2 out]
                    n1002 = Unbundle(w1735) -> ("T-RISE mins"=w1734:dbl)  [unwired: 4 out]
                    n1003 = Greater Or Equal?(x=w1737, y=w1736) -> (x >= y?=w1738:bool)
                    n1004 = case shown="True" w1738 {
                      tunnel: w1734 -> [w1741 _]
                      tunnel: w1733 -> [w1740 _]
                      tunnel: w1732 -> [w1739 _]
                      frame True {
                        n1005 = stacked-sequence {
                          tunnel: w1741 -> [w1744 _]
                          tunnel: w1740 -> [_ w1749]
                          tunnel: w1739 -> [w1742 _]
                          frame #0 {
                            n1006 = Build Array("T-RISE") -> (w1746:string[])
                            n1007 = Build Array(w1744) -> (w1745:dbl[])
                            n1008 = TDMS Write(0:w1742, 5:"TEST PASS", 7:w1746, 9:w1745) -> (15:w1748:errorcluster)  [unwired: 2 in, 3 out]
                            n1009 = local write "data file error"(w1748) -> ()
                          }
                          frame #1 {
                            n1010 = Bundle(cluster=w1749, "STATUS"="T-RISE PASS") -> (w1751:T4)  [unwired: 2 in]
                            n1011 = local write "LAB04-2 (RESULT)"(TRUE) -> ()
                            n1012 = local write "LAB04-2 (DISP)"(w1751) -> ()
                          }
                        }
                      }
                      frame False {
                      }
                    }
                  }
                }
              }
              frame #8 {
                # "LAB05-1"
                n1013 = Equal?(x=w1753, y=2) -> (x = y?=w1757:bool)
                n1014 = local read "LAB05-1 (DISP)"() -> (w1759:T4)
                n1015 = Unbundle(w1759) -> ("STATUS"=w1760:string)  [unwired: 2 out]
                n1016 = Equal?(x=w1760, y="RUN") -> (x = y?=w1756:bool)
                n1017 = And(x=w1756, y=w1757) -> (x .and. y?=w1755:bool)
                n1018 = case shown="True" w1755 {
                  tunnel: w1759 -> [_ w1763]
                  tunnel: w1754 -> [_ w1766]
                  frame False {
                  }
                  frame True {
                    n1019 = local read "LAB05-1 (SET)"() -> (w1765:T5)
                    n1020 = local read "LAB05-1 (TDMS)"() -> (w1762:refnum<k34>)
                    n1021 = Unbundle(w1763) -> ("CYCLE"=w1767:dbl)  [unwired: 2 out]
                    n1022 = Unbundle(w1765) -> ("T-RISE mins"=w1764:dbl)  [unwired: 4 out]
                    n1023 = Greater Or Equal?(x=w1767, y=w1766) -> (x >= y?=w1768:bool)
                    n1024 = case shown="True" w1768 {
                      tunnel: w1764 -> [w1771 _]
                      tunnel: w1763 -> [w1770 _]
                      tunnel: w1762 -> [w1769 _]
                      frame True {
                        n1025 = stacked-sequence {
                          tunnel: w1771 -> [w1774 _]
                          tunnel: w1770 -> [_ w1779]
                          tunnel: w1769 -> [w1772 _]
                          frame #0 {
                            n1026 = Build Array("T-RISE") -> (w1776:string[])
                            n1027 = Build Array(w1774) -> (w1775:dbl[])
                            n1028 = TDMS Write(0:w1772, 5:"TEST PASS", 7:w1776, 9:w1775) -> (15:w1778:errorcluster)  [unwired: 2 in, 3 out]
                            n1029 = local write "data file error"(w1778) -> ()
                          }
                          frame #1 {
                            n1030 = Bundle(cluster=w1779, "STATUS"="T-RISE PASS") -> (w1781:T4)  [unwired: 2 in]
                            n1031 = local write "LAB05-1 (RESULT)"(TRUE) -> ()
                            n1032 = local write "LAB05-1 (DISP)"(w1781) -> ()
                          }
                        }
                      }
                      frame False {
                      }
                    }
                  }
                }
              }
              frame #9 {
                # "LAB05-2"
                n1033 = Equal?(x=w1783, y=2) -> (x = y?=w1787:bool)
                n1034 = local read "LAB05-2 (DISP)"() -> (w1789:T4)
                n1035 = Unbundle(w1789) -> ("STATUS"=w1790:string)  [unwired: 2 out]
                n1036 = Equal?(x=w1790, y="RUN") -> (x = y?=w1786:bool)
                n1037 = And(x=w1786, y=w1787) -> (x .and. y?=w1785:bool)
                n1038 = case shown="True" w1785 {
                  tunnel: w1789 -> [_ w1793]
                  tunnel: w1784 -> [_ w1796]
                  frame False {
                  }
                  frame True {
                    n1039 = local read "LAB05-2 (SET)"() -> (w1795:T5)
                    n1040 = local read "LAB05-2 (TDMS)"() -> (w1792:refnum<k34>)
                    n1041 = Unbundle(w1793) -> ("CYCLE"=w1797:dbl)  [unwired: 2 out]
                    n1042 = Unbundle(w1795) -> ("T-RISE mins"=w1794:dbl)  [unwired: 4 out]
                    n1043 = Greater Or Equal?(x=w1797, y=w1796) -> (x >= y?=w1798:bool)
                    n1044 = case shown="True" w1798 {
                      tunnel: w1794 -> [w1801 _]
                      tunnel: w1793 -> [w1800 _]
                      tunnel: w1792 -> [w1799 _]
                      frame True {
                        n1045 = stacked-sequence {
                          tunnel: w1801 -> [w1804 _]
                          tunnel: w1800 -> [_ w1809]
                          tunnel: w1799 -> [w1802 _]
                          frame #0 {
                            n1046 = Build Array("T-RISE") -> (w1806:string[])
                            n1047 = Build Array(w1804) -> (w1805:dbl[])
                            n1048 = TDMS Write(0:w1802, 5:"TEST PASS", 7:w1806, 9:w1805) -> (15:w1808:errorcluster)  [unwired: 2 in, 3 out]
                            n1049 = local write "data file error"(w1808) -> ()
                          }
                          frame #1 {
                            n1050 = Bundle(cluster=w1809, "STATUS"="T-RISE PASS") -> (w1811:T4)  [unwired: 2 in]
                            n1051 = local write "LAB05-2 (RESULT)"(TRUE) -> ()
                            n1052 = local write "LAB05-2 (DISP)"(w1811) -> ()
                          }
                        }
                      }
                      frame False {
                      }
                    }
                  }
                }
              }
            }
          }
          frame #6 {
            # "disable functions"
            n1053 = stacked-sequence {
              tunnel: w1822 -> [w1835 _ w1892]
              tunnel: w1821 -> [w1830 _ w1891]
              tunnel: w1820 -> [w1827 _ w1890]
              tunnel: w1819 -> [w1823 _ w1889]
              tunnel: w1818 -> [w1824 _ w1888]
              tunnel: w1817 -> [_ w1848 w1887]
              tunnel: w1816 -> [_ w1850 w1886]
              tunnel: w1815 -> [_ w1851 w1885]
              tunnel: w1814 -> [_ w1853 w1884]
              tunnel: w1813 -> [_ w1855 w1883]
              frame #0 {
                n1054 = Select(t=2, s=w1823, f=0) -> (s? t:f=w1826:i32)
                n1055 = Select(t=2, s=w1827, f=0) -> (s? t:f=w1828:i32)
                n1056 = Select(t=2, s=w1824, f=0) -> (s? t:f=w1825:i32)
                n1057 = Select(t=2, s=w1835, f=0) -> (s? t:f=w1837:i32)
                n1058 = Select(t=2, s=w1830, f=0) -> (s? t:f=w1829:i32)
                n1059 = property on="LAB02-2 SELECT" class="RadioBtnsControl (strict)"("DisabledEnum"=w1826) -> ()  [unwired: 2 in, 2 out]
                n1060 = property on="LAB02-1 SELECT" class="RadioBtnsControl (strict)"("DisabledEnum"=w1828) -> ()  [unwired: 2 in, 2 out]
                n1061 = property on="LAB03-1 SELECT" class="RadioBtnsControl (strict)"("DisabledEnum"=w1825) -> ()  [unwired: 2 in, 2 out]
                n1062 = property on="LAB01-1 SELECT" class="RadioBtnsControl (strict)"("DisabledEnum"=w1837) -> ()  [unwired: 2 in, 2 out]
                n1063 = property on="LAB01-2 SELECT" class="RadioBtnsControl (strict)"("DisabledEnum"=w1829) -> ()  [unwired: 2 in, 2 out]
                n1064 = Not(x=w1835) -> (.not. x?=w1836:bool)
                n1065 = property on="LAB01-1 (RESULT)" class="Bool (strict)"("Visible"=w1836) -> ()  [unwired: 2 in, 2 out]
                n1066 = Not(x=w1830) -> (.not. x?=w1834:bool)
                n1067 = Not(x=w1827) -> (.not. x?=w1833:bool)
                n1068 = Not(x=w1823) -> (.not. x?=w1832:bool)
                n1069 = property on="LAB01-2 (RESULT)" class="Bool (strict)"("Visible"=w1834) -> ()  [unwired: 2 in, 2 out]
                n1070 = Not(x=w1824) -> (.not. x?=w1831:bool)
                n1071 = property on="LAB02-1 (RESULT)" class="Bool (strict)"("Visible"=w1833) -> ()  [unwired: 2 in, 2 out]
                n1072 = property on="LAB02-2 (RESULT)" class="Bool (strict)"("Visible"=w1832) -> ()  [unwired: 2 in, 2 out]
                n1073 = property on="LAB03-1 (RESULT)" class="Bool (strict)"("Visible"=w1831) -> ()  [unwired: 2 in, 2 out]
              }
              frame #1 {
                n1074 = Select(t=2, s=w1855, f=0) -> (s? t:f=w1856:i32)
                n1075 = Select(t=2, s=w1853, f=0) -> (s? t:f=w1854:i32)
                n1076 = Select(t=2, s=w1848, f=0) -> (s? t:f=w1862:i32)
                n1077 = Select(t=2, s=w1850, f=0) -> (s? t:f=w1849:i32)
                n1078 = Select(t=2, s=w1851, f=0) -> (s? t:f=w1852:i32)
                n1079 = property on="LAB05-2 SELECT" class="RadioBtnsControl (strict)"("DisabledEnum"=w1856) -> ()  [unwired: 2 in, 2 out]
                n1080 = property on="LAB05-1 SELECT" class="RadioBtnsControl (strict)"("DisabledEnum"=w1854) -> ()  [unwired: 2 in, 2 out]
                n1081 = property on="LAB03-2 SELECT" class="RadioBtnsControl (strict)"("DisabledEnum"=w1862) -> ()  [unwired: 2 in, 2 out]
                n1082 = property on="LAB04-1 SELECT" class="RadioBtnsControl (strict)"("DisabledEnum"=w1849) -> ()  [unwired: 2 in, 2 out]
                n1083 = property on="LAB04-2 SELECT" class="RadioBtnsControl (strict)"("DisabledEnum"=w1852) -> ()  [unwired: 2 in, 2 out]
                n1084 = Not(x=w1848) -> (.not. x?=w1861:bool)
                n1085 = Not(x=w1855) -> (.not. x?=w1857:bool)
                n1086 = property on="LAB03-2 (RESULT)" class="Bool (strict)"("Visible"=w1861) -> ()  [unwired: 2 in, 2 out]
                n1087 = Not(x=w1853) -> (.not. x?=w1858:bool)
                n1088 = Not(x=w1851) -> (.not. x?=w1859:bool)
                n1089 = property on="LAB05-2 (RESULT)" class="Bool (strict)"("Visible"=w1857) -> ()  [unwired: 2 in, 2 out]
                n1090 = property on="LAB05-1 (RESULT)" class="Bool (strict)"("Visible"=w1858) -> ()  [unwired: 2 in, 2 out]
                n1091 = Not(x=w1850) -> (.not. x?=w1860:bool)
                n1092 = property on="LAB04-2 (RESULT)" class="Bool (strict)"("Visible"=w1859) -> ()  [unwired: 2 in, 2 out]
                n1093 = property on="LAB04-1 (RESULT)" class="Bool (strict)"("Visible"=w1860) -> ()  [unwired: 2 in, 2 out]
              }
              frame #2 {
                # "disable calibrate if any test running"
                n1094 = Or(x=w1884, y=w1883) -> (x .or. y?=w1877:bool)
                n1095 = Or(x=w1886, y=w1885) -> (x .or. y?=w1879:bool)
                n1096 = Or(x=w1890, y=w1889) -> (x .or. y?=w1881:bool)
                n1097 = Or(x=w1888, y=w1887) -> (x .or. y?=w1880:bool)
                n1098 = Or(x=w1892, y=w1891) -> (x .or. y?=w1882:bool)
                n1099 = Or(x=w1880, y=w1879) -> (x .or. y?=w1878:bool)
                n1100 = Or(x=w1882, y=w1881) -> (x .or. y?=w1876:bool)
                n1101 = Or(x=w1878, y=w1877) -> (x .or. y?=w1875:bool)
                n1102 = Or(x=w1876, y=w1875) -> (x .or. y?=w1874:bool)
                n1103 = case shown="False" w1874 {
                  tunnel: [0 2] -> w1873
                  frame False {
                  }
                  frame True {
                  }
                }
                n1104 = property on="CALIBRATE" class="Bool (strict)"("DisabledEnum"=w1873) -> ()  [unwired: 2 in, 2 out]
              }
            }
          }
          frame #7 {
            # "end test & close test files"
            n1105 = stacked-sequence {
              tunnel: w1903 -> [w1905 _ _ _ _ _ _ _ _ _]
              tunnel: w1904 -> [_ w1918 _ _ _ _ _ _ _ _]
              tunnel: w1902 -> [_ _ w1931 _ _ _ _ _ _ _]
              tunnel: w1901 -> [_ _ _ w1944 _ _ _ _ _ _]
              tunnel: w1900 -> [_ _ _ _ w1957 _ _ _ _ _]
              tunnel: w1899 -> [_ _ _ _ _ w1970 _ _ _ _]
              tunnel: w1898 -> [_ _ _ _ _ _ w1983 _ _ _]
              tunnel: w1897 -> [_ _ _ _ _ _ _ w1996 _ _]
              tunnel: w1896 -> [_ _ _ _ _ _ _ _ w2009 _]
              tunnel: w1895 -> [_ _ _ _ _ _ _ _ _ w2022]
              frame #0 {
                # "LAB01-1"
                n1106 = case shown="True" w1905 {
                  frame False {
                  }
                  frame True {
                    n1107 = local read "LAB01-1 (DISP)"() -> (w1908:T4)
                    n1108 = local read "LAB01-1 (TDMS)"() -> (w1907:refnum<k34>)
                    n1109 = Unbundle(w1908) -> ("STATUS"=w1906:string)  [unwired: 2 out]
                    n1110 = Not Equal?(x=w1906, y="RUN") -> (x != y?=w1909:bool)
                    n1111 = case shown="True" w1909 {
                      tunnel: w1908 -> [_ w1912]
                      tunnel: w1907 -> [_ w1911]
                      frame False {
                      }
                      frame True {
                        n1112 = stacked-sequence {
                          tunnel: w1912 -> [w1914 _]
                          tunnel: w1911 -> [_ w1916]
                          frame #0 {
                            (unwired) "END"
                            n1113 = Bundle(cluster=w1914) -> (w1913:T4)  [unwired: 3 in]
                            n1114 = local write "LAB01-1 (DISP)"(w1913) -> ()
                            n1115 = local write "LAB01-1RUN"(FALSE) -> ()
                          }
                          frame #1 {
                            n1116 = TDMS Close(11:w1916) -> (0:w1917:errorcluster)  [unwired: 1 in, 1 out]
                            n1117 = local write "data file error"(w1917) -> ()
                          }
                        }
                      }
                    }
                  }
                }
              }
              frame #1 {
                # "LAB01-2"
                n1118 = case shown="True" w1918 {
                  frame False {
                  }
                  frame True {
                    n1119 = local read "LAB01-2 (DISP)"() -> (w1920:T4)
                    n1120 = local read "LAB01-2 (TDMS)"() -> (w1919:refnum<k34>)
                    n1121 = Unbundle(w1920) -> ("STATUS"=w1921:string)  [unwired: 2 out]
                    n1122 = Not Equal?(x=w1921, y="RUN") -> (x != y?=w1922:bool)
                    n1123 = case shown="True" w1922 {
                      tunnel: w1920 -> [_ w1925]
                      tunnel: w1919 -> [_ w1924]
                      frame False {
                      }
                      frame True {
                        n1124 = stacked-sequence {
                          tunnel: w1925 -> [w1927 _]
                          tunnel: w1924 -> [_ w1929]
                          frame #0 {
                            (unwired) "END"
                            n1125 = Bundle(cluster=w1927) -> (w1928:T4)  [unwired: 3 in]
                            n1126 = local write "LAB01-2 RUN"(FALSE) -> ()
                            n1127 = local write "LAB01-2 (DISP)"(w1928) -> ()
                          }
                          frame #1 {
                            n1128 = TDMS Close(11:w1929) -> (0:w1930:errorcluster)  [unwired: 1 in, 1 out]
                            n1129 = local write "data file error"(w1930) -> ()
                          }
                        }
                      }
                    }
                  }
                }
              }
              frame #2 {
                # "LAB02-1"
                n1130 = case shown="True" w1931 {
                  frame False {
                  }
                  frame True {
                    n1131 = local read "LAB02-1 (DISP)"() -> (w1933:T4)
                    n1132 = local read "LAB02-1 (TDMS)"() -> (w1932:refnum<k34>)
                    n1133 = Unbundle(w1933) -> ("STATUS"=w1934:string)  [unwired: 2 out]
                    n1134 = Not Equal?(x=w1934, y="RUN") -> (x != y?=w1935:bool)
                    n1135 = case shown="True" w1935 {
                      tunnel: w1933 -> [_ w1938]
                      tunnel: w1932 -> [_ w1937]
                      frame False {
                      }
                      frame True {
                        n1136 = stacked-sequence {
                          tunnel: w1938 -> [w1940 _]
                          tunnel: w1937 -> [_ w1942]
                          frame #0 {
                            (unwired) "END"
                            n1137 = Bundle(cluster=w1940) -> (w1941:T4)  [unwired: 3 in]
                            n1138 = local write "LAB02-1 RUN"(FALSE) -> ()
                            n1139 = local write "LAB02-1 (DISP)"(w1941) -> ()
                          }
                          frame #1 {
                            n1140 = TDMS Close(11:w1942) -> (0:w1943:errorcluster)  [unwired: 1 in, 1 out]
                            n1141 = local write "data file error"(w1943) -> ()
                          }
                        }
                      }
                    }
                  }
                }
              }
              frame #3 {
                # "LAB02-2"
                n1142 = case shown="True" w1944 {
                  frame False {
                  }
                  frame True {
                    n1143 = local read "LAB02-2 (DISP)"() -> (w1946:T4)
                    n1144 = local read "LAB02-2 (TDMS)"() -> (w1945:refnum<k34>)
                    n1145 = Unbundle(w1946) -> ("STATUS"=w1947:string)  [unwired: 2 out]
                    n1146 = Not Equal?(x=w1947, y="RUN") -> (x != y?=w1948:bool)
                    n1147 = case shown="True" w1948 {
                      tunnel: w1946 -> [_ w1951]
                      tunnel: w1945 -> [_ w1950]
                      frame False {
                      }
                      frame True {
                        n1148 = stacked-sequence {
                          tunnel: w1951 -> [w1953 _]
                          tunnel: w1950 -> [_ w1955]
                          frame #0 {
                            (unwired) "END"
                            n1149 = Bundle(cluster=w1953) -> (w1954:T4)  [unwired: 3 in]
                            n1150 = local write "LAB02-2 RUN"(FALSE) -> ()
                            n1151 = local write "LAB02-2 (DISP)"(w1954) -> ()
                          }
                          frame #1 {
                            n1152 = TDMS Close(11:w1955) -> (0:w1956:errorcluster)  [unwired: 1 in, 1 out]
                            n1153 = local write "data file error"(w1956) -> ()
                          }
                        }
                      }
                    }
                  }
                }
              }
              frame #4 {
                # "LAB03-1"
                n1154 = case shown="True" w1957 {
                  frame False {
                  }
                  frame True {
                    n1155 = local read "LAB03-1 (DISP)"() -> (w1959:T4)
                    n1156 = local read "LAB03-1 (TDMS)"() -> (w1958:refnum<k34>)
                    n1157 = Unbundle(w1959) -> ("STATUS"=w1960:string)  [unwired: 2 out]
                    n1158 = Not Equal?(x=w1960, y="RUN") -> (x != y?=w1961:bool)
                    n1159 = case shown="True" w1961 {
                      tunnel: w1959 -> [_ w1964]
                      tunnel: w1958 -> [_ w1963]
                      frame False {
                      }
                      frame True {
                        n1160 = stacked-sequence {
                          tunnel: w1964 -> [w1966 _]
                          tunnel: w1963 -> [_ w1968]
                          frame #0 {
                            (unwired) "END"
                            n1161 = Bundle(cluster=w1966) -> (w1967:T4)  [unwired: 3 in]
                            n1162 = local write "LAB03-1 RUN"(FALSE) -> ()
                            n1163 = local write "LAB03-1 (DISP)"(w1967) -> ()
                          }
                          frame #1 {
                            n1164 = TDMS Close(11:w1968) -> (0:w1969:errorcluster)  [unwired: 1 in, 1 out]
                            n1165 = local write "data file error"(w1969) -> ()
                          }
                        }
                      }
                    }
                  }
                }
              }
              frame #5 {
                # "LAB03-2"
                n1166 = case shown="True" w1970 {
                  frame False {
                  }
                  frame True {
                    n1167 = local read "LAB03-2 (DISP)"() -> (w1972:T4)
                    n1168 = local read "LAB03-2 (TDMS)"() -> (w1971:refnum<k34>)
                    n1169 = Unbundle(w1972) -> ("STATUS"=w1973:string)  [unwired: 2 out]
                    n1170 = Not Equal?(x=w1973, y="RUN") -> (x != y?=w1974:bool)
                    n1171 = case shown="True" w1974 {
                      tunnel: w1972 -> [_ w1977]
                      tunnel: w1971 -> [_ w1976]
                      frame False {
                      }
                      frame True {
                        n1172 = stacked-sequence {
                          tunnel: w1977 -> [w1979 _]
                          tunnel: w1976 -> [_ w1981]
                          frame #0 {
                            (unwired) "END"
                            n1173 = Bundle(cluster=w1979) -> (w1980:T4)  [unwired: 3 in]
                            n1174 = local write "LAB03-2 RUN"(FALSE) -> ()
                            n1175 = local write "LAB03-2 (DISP)"(w1980) -> ()
                          }
                          frame #1 {
                            n1176 = TDMS Close(11:w1981) -> (0:w1982:errorcluster)  [unwired: 1 in, 1 out]
                            n1177 = local write "data file error"(w1982) -> ()
                          }
                        }
                      }
                    }
                  }
                }
              }
              frame #6 {
                # "LAB04-1"
                n1178 = case shown="True" w1983 {
                  frame False {
                  }
                  frame True {
                    n1179 = local read "LAB04-1 (DISP)"() -> (w1985:T4)
                    n1180 = local read "LAB04-1 (TDMS)"() -> (w1984:refnum<k34>)
                    n1181 = Unbundle(w1985) -> ("STATUS"=w1986:string)  [unwired: 2 out]
                    n1182 = Not Equal?(x=w1986, y="RUN") -> (x != y?=w1987:bool)
                    n1183 = case shown="True" w1987 {
                      tunnel: w1985 -> [_ w1990]
                      tunnel: w1984 -> [_ w1989]
                      frame False {
                      }
                      frame True {
                        n1184 = stacked-sequence {
                          tunnel: w1990 -> [w1992 _]
                          tunnel: w1989 -> [_ w1994]
                          frame #0 {
                            (unwired) "END"
                            n1185 = Bundle(cluster=w1992) -> (w1993:T4)  [unwired: 3 in]
                            n1186 = local write "LAB04-1 RUN"(FALSE) -> ()
                            n1187 = local write "LAB04-1 (DISP)"(w1993) -> ()
                          }
                          frame #1 {
                            n1188 = TDMS Close(11:w1994) -> (0:w1995:errorcluster)  [unwired: 1 in, 1 out]
                            n1189 = local write "data file error"(w1995) -> ()
                          }
                        }
                      }
                    }
                  }
                }
              }
              frame #7 {
                # "LAB04-2"
                n1190 = case shown="True" w1996 {
                  frame False {
                  }
                  frame True {
                    n1191 = local read "LAB04-2 (DISP)"() -> (w1998:T4)
                    n1192 = local read "LAB04-2 (TDMS)"() -> (w1997:refnum<k34>)
                    n1193 = Unbundle(w1998) -> ("STATUS"=w1999:string)  [unwired: 2 out]
                    n1194 = Not Equal?(x=w1999, y="RUN") -> (x != y?=w2000:bool)
                    n1195 = case shown="True" w2000 {
                      tunnel: w1998 -> [_ w2003]
                      tunnel: w1997 -> [_ w2002]
                      frame False {
                      }
                      frame True {
                        n1196 = stacked-sequence {
                          tunnel: w2003 -> [w2005 _]
                          tunnel: w2002 -> [_ w2007]
                          frame #0 {
                            (unwired) "END"
                            n1197 = Bundle(cluster=w2005) -> (w2006:T4)  [unwired: 3 in]
                            n1198 = local write "LAB04-2 RUN"(FALSE) -> ()
                            n1199 = local write "LAB04-2 (DISP)"(w2006) -> ()
                          }
                          frame #1 {
                            n1200 = TDMS Close(11:w2007) -> (0:w2008:errorcluster)  [unwired: 1 in, 1 out]
                            n1201 = local write "data file error"(w2008) -> ()
                          }
                        }
                      }
                    }
                  }
                }
              }
              frame #8 {
                # "LAB05-1"
                n1202 = case shown="True" w2009 {
                  frame False {
                  }
                  frame True {
                    n1203 = local read "LAB05-1 (DISP)"() -> (w2011:T4)
                    n1204 = local read "LAB05-1 (TDMS)"() -> (w2010:refnum<k34>)
                    n1205 = Unbundle(w2011) -> ("STATUS"=w2012:string)  [unwired: 2 out]
                    n1206 = Not Equal?(x=w2012, y="RUN") -> (x != y?=w2013:bool)
                    n1207 = case shown="True" w2013 {
                      tunnel: w2011 -> [_ w2016]
                      tunnel: w2010 -> [_ w2015]
                      frame False {
                      }
                      frame True {
                        n1208 = stacked-sequence {
                          tunnel: w2016 -> [w2018 _]
                          tunnel: w2015 -> [_ w2020]
                          frame #0 {
                            (unwired) "END"
                            n1209 = Bundle(cluster=w2018) -> (w2019:T4)  [unwired: 3 in]
                            n1210 = local write "LAB05-1 RUN"(FALSE) -> ()
                            n1211 = local write "LAB05-1 (DISP)"(w2019) -> ()
                          }
                          frame #1 {
                            n1212 = TDMS Close(11:w2020) -> (0:w2021:errorcluster)  [unwired: 1 in, 1 out]
                            n1213 = local write "data file error"(w2021) -> ()
                          }
                        }
                      }
                    }
                  }
                }
              }
              frame #9 {
                # "LAB05-2"
                n1214 = case shown="True" w2022 {
                  frame False {
                  }
                  frame True {
                    n1215 = local read "LAB05-2 (DISP)"() -> (w2024:T4)
                    n1216 = local read "LAB05-2 (TDMS)"() -> (w2023:refnum<k34>)
                    n1217 = Unbundle(w2024) -> ("STATUS"=w2025:string)  [unwired: 2 out]
                    n1218 = Not Equal?(x=w2025, y="RUN") -> (x != y?=w2026:bool)
                    n1219 = case shown="True" w2026 {
                      tunnel: w2024 -> [_ w2029]
                      tunnel: w2023 -> [_ w2028]
                      frame False {
                      }
                      frame True {
                        n1220 = stacked-sequence {
                          tunnel: w2029 -> [w2031 _]
                          tunnel: w2028 -> [_ w2033]
                          frame #0 {
                            (unwired) "END"
                            n1221 = Bundle(cluster=w2031) -> (w2032:T4)  [unwired: 3 in]
                            n1222 = local write "LAB05-2 RUN"(FALSE) -> ()
                            n1223 = local write "LAB05-2 (DISP)"(w2032) -> ()
                          }
                          frame #1 {
                            n1224 = TDMS Close(11:w2033) -> (0:w2034:errorcluster)  [unwired: 1 in, 1 out]
                            n1225 = local write "data file error"(w2034) -> ()
                          }
                        }
                      }
                    }
                  }
                }
              }
            }
          }
          frame #8 {
            # "drive jigs"
            n1226 = stacked-sequence {
              frame #0 {
                # "jig on"
                n1227 = local read "jig cycle"() -> (w2035:dbl)
                n1228 = Equal?(x=w2035, y=0) -> (x = y?=w2037:bool)
                n1229 = case shown="True" w2037 {
                  frame False {
                  }
                  frame True {
                    n1230 = local read "LAB01-1RUN"() -> (w2038:bool)
                    n1231 = local read "LAB01-2 RUN"() -> (w2039:bool)
                    n1232 = local read "LAB03-1 RUN"() -> (w2045:bool)
                    n1233 = local read "LAB03-2 RUN"() -> (w2044:bool)
                    n1234 = local read "LAB02-1 RUN"() -> (w2047:bool)
                    n1235 = local read "LAB02-2 RUN"() -> (w2046:bool)
                    n1236 = local read "LAB04-1 RUN"() -> (w2043:bool)
                    n1237 = local read "LAB04-2 RUN"() -> (w2042:bool)
                    n1238 = local read "LAB05-1 RUN"() -> (w2041:bool)
                    n1239 = local read "LAB05-2 RUN"() -> (w2040:bool)
                    n1240 = local write "LAB05-1 (JIG)"(w2041) -> ()
                    n1241 = local write "LAB05-2 (JIG)"(w2040) -> ()
                    n1242 = local write "LAB04-2 (JIG)"(w2042) -> ()
                    n1243 = local write "LAB02-1 (JIG)"(w2047) -> ()
                    n1244 = local write "LAB03-1 (JIG)"(w2045) -> ()
                    n1245 = local write "LAB04-1 (JIG)"(w2043) -> ()
                    n1246 = local write "LAB03-2 (JIG)"(w2044) -> ()
                    n1247 = local write "LAB02-2 (JIG)"(w2046) -> ()
                    n1248 = local write "LAB01-1 (JIG)"(w2038) -> ()
                    n1249 = local write "LAB01-2 (JIG)"(w2039) -> ()
                  }
                }
              }
              frame #1 {
                # "jig off"
                n1250 = local read "jig cycle"() -> (w2050:dbl)
                n1251 = local read "on loops"() -> (w2049:dbl)
                n1252 = Equal?(x=w2050, y=w2049) -> (x = y?=w2048:bool)
                n1253 = case shown="True" w2048 {
                  frame False {
                  }
                  frame True {
                    w2101 = FALSE
                    w2102 = TRUE
                    w2100 = 2
                    n1254 = local read "LAB05-2 SELECT"() -> (w2091:T3)
                    n1255 = local read "LAB04-2 SELECT"() -> (w2093:T3)
                    n1256 = local read "LAB04-1 SELECT"() -> (w2094:T3)
                    n1257 = local read "LAB05-1 SELECT"() -> (w2092:T3)
                    n1258 = local read "LAB03-2 SELECT"() -> (w2095:T3)
                    n1259 = local read "LAB02-1 SELECT"() -> (w2098:T3)
                    n1260 = local read "LAB03-1 SELECT"() -> (w2096:T3)
                    n1261 = local read "LAB02-2 SELECT"() -> (w2097:T3)
                    n1262 = local read "LAB01-2 SELECT"() -> (w2099:T3)
                    n1263 = local read "LAB05-1 RUN"() -> (w2061:bool)
                    n1264 = local read "LAB05-2 RUN"() -> (w2060:bool)
                    n1265 = local read "LAB04-2 RUN"() -> (w2062:bool)
                    n1266 = local read "LAB04-1 RUN"() -> (w2063:bool)
                    n1267 = local read "LAB01-2 RUN"() -> (w2068:bool)
                    n1268 = local read "LAB03-2 RUN"() -> (w2064:bool)
                    n1269 = local read "LAB01-1RUN"() -> (w2079:bool)
                    n1270 = local read "LAB01-1 SELECT"() -> (w2103:T3)
                    n1271 = local read "LAB03-1 RUN"() -> (w2065:bool)
                    n1272 = local read "LAB02-1 RUN"() -> (w2067:bool)
                    n1273 = local read "LAB02-2 RUN"() -> (w2066:bool)
                    n1274 = Equal?(x=w2100, y=w2096) -> (x = y?=w2074:bool)
                    n1275 = Equal?(x=w2100, y=w2095) -> (x = y?=w2073:bool)
                    n1276 = Equal?(x=w2100, y=w2094) -> (x = y?=w2072:bool)
                    n1277 = Equal?(x=w2100, y=w2093) -> (x = y?=w2071:bool)
                    n1278 = Equal?(x=w2100, y=w2092) -> (x = y?=w2070:bool)
                    n1279 = Equal?(x=w2100, y=w2091) -> (x = y?=w2069:bool)
                    n1280 = Equal?(x=w2100, y=w2103) -> (x = y?=w2080:bool)
                    n1281 = Equal?(x=w2100, y=w2098) -> (x = y?=w2076:bool)
                    n1282 = Equal?(x=w2100, y=w2097) -> (x = y?=w2075:bool)
                    n1283 = Equal?(x=w2100, y=w2099) -> (x = y?=w2077:bool)
                    n1284 = And(x=w2071, y=w2062) -> (x .and. y?=w2053:bool)
                    n1285 = And(x=w2074, y=w2065) -> (x .and. y?=w2056:bool)
                    n1286 = And(x=w2072, y=w2063) -> (x .and. y?=w2054:bool)
                    n1287 = And(x=w2069, y=w2060) -> (x .and. y?=w2051:bool)
                    n1288 = And(x=w2075, y=w2066) -> (x .and. y?=w2057:bool)
                    n1289 = And(x=w2073, y=w2064) -> (x .and. y?=w2055:bool)
                    n1290 = And(x=w2070, y=w2061) -> (x .and. y?=w2052:bool)
                    n1291 = And(x=w2077, y=w2068) -> (x .and. y?=w2059:bool)
                    n1292 = And(x=w2080, y=w2079) -> (x .and. y?=w2078:bool)
                    n1293 = And(x=w2076, y=w2067) -> (x .and. y?=w2058:bool)
                    n1294 = Select(t=w2102, s=w2078, f=w2101) -> (s? t:f=w2081:bool)
                    n1295 = Select(t=w2102, s=w2059, f=w2101) -> (s? t:f=w2082:bool)
                    n1296 = Select(t=w2102, s=w2058, f=w2101) -> (s? t:f=w2083:bool)
                    n1297 = Select(t=w2102, s=w2057, f=w2101) -> (s? t:f=w2084:bool)
                    n1298 = Select(t=w2102, s=w2056, f=w2101) -> (s? t:f=w2085:bool)
                    n1299 = Select(t=w2102, s=w2055, f=w2101) -> (s? t:f=w2086:bool)
                    n1300 = Select(t=w2102, s=w2054, f=w2101) -> (s? t:f=w2087:bool)
                    n1301 = Select(t=w2102, s=w2053, f=w2101) -> (s? t:f=w2088:bool)
                    n1302 = Select(t=w2102, s=w2052, f=w2101) -> (s? t:f=w2089:bool)
                    n1303 = Select(t=w2102, s=w2051, f=w2101) -> (s? t:f=w2090:bool)
                    n1304 = local write "LAB03-2 (JIG)"(w2086) -> ()
                    n1305 = local write "LAB02-1 (JIG)"(w2083) -> ()
                    n1306 = local write "LAB02-2 (JIG)"(w2084) -> ()
                    n1307 = local write "LAB01-2 (JIG)"(w2082) -> ()
                    n1308 = local write "LAB03-1 (JIG)"(w2085) -> ()
                    n1309 = local write "LAB01-1 (JIG)"(w2081) -> ()
                    n1310 = local write "LAB05-2 (JIG)"(w2090) -> ()
                    n1311 = local write "LAB04-1 (JIG)"(w2087) -> ()
                    n1312 = local write "LAB05-1 (JIG)"(w2089) -> ()
                    n1313 = local write "LAB04-2 (JIG)"(w2088) -> ()
                  }
                }
              }
            }
          }
          frame #9 {
            # "drive digital output"
            n1314 = local read "LAB05-2 (O/I)"() -> (w2109:bool)
            n1315 = local read "LAB05-2 (JIG)"() -> (w2108:bool)
            n1316 = local read "LAB05-1 (O/I)"() -> (w2111:bool)
            n1317 = local read "LAB05-1 (JIG)"() -> (w2110:bool)
            n1318 = local read "LAB04-2 (O/I)"() -> (w2113:bool)
            n1319 = local read "LAB04-2 (JIG)"() -> (w2112:bool)
            n1320 = local read "LAB03-1 (O/I)"() -> (w2118:bool)
            n1321 = local read "LAB04-1 (O/I)"() -> (w2114:bool)
            n1322 = local read "LAB04-1 (JIG)"() -> (w2107:bool)
            n1323 = local read "LAB02-1 (O/I)"() -> (w2122:bool)
            n1324 = local read "LAB02-2 (O/I)"() -> (w2120:bool)
            n1325 = local read "LAB03-2 (O/I)"() -> (w2116:bool)
            n1326 = local read "LAB03-2 (JIG)"() -> (w2115:bool)
            n1327 = local read "LAB02-1 (JIG)"() -> (w2121:bool)
            n1328 = local read "LAB02-2 (JIG)"() -> (w2119:bool)
            n1329 = local read "LAB03-1 (JIG)"() -> (w2117:bool)
            n1330 = local read "LAB01-2 (O/I)"() -> (w2124:bool)
            n1331 = local read "LAB01-2 (JIG)"() -> (w2123:bool)
            n1332 = local read "LAB01-1 (O/I)"() -> (w2126:bool)
            n1333 = local read "LAB01-1 (JIG)"() -> (w2125:bool)
            n1334 = Build Array(w2113, w2112, w2111, w2110, w2109, w2108) -> (w2104:bool[])
            n1335 = Build Array(w2119, w2118, w2117, w2116, w2115, w2114, w2107) -> (w2105:bool[])
            n1336 = Build Array(w2126, w2125, w2124, w2123, w2122, w2121, w2120) -> (w2106:bool[])
            n1337 = call "sub vi - Drive Relays All v6.vi"("Array #2"=w2104, "Array #1"=w2105, "Array #0"=w2106) -> ()  [unwired: 8 in, 1 out]
          }
          frame #10 {
            # "get temperature values"
            n1338 = stacked-sequence {
              frame #0 {
                n1339 = local read "jig cycle"() -> (w2127:dbl)
                n1340 = local read "on loops"() -> (w2130:dbl)
                n1341 = local read "jig cycle"() -> (w2132:dbl)
                n1342 = Add(x=w2130, y=2) -> (x+y=w2131:dbl)
                n1343 = Equal?(x=w2132, y=0) -> (x = y?=w2133:bool)
                n1344 = Equal?(x=w2127, y=w2131) -> (x = y?=w2128:bool)
                n1345 = case shown="True" w2133 {
                  frame False {
                  }
                  frame True {
                    w2145 = FALSE
                    w2146 = TRUE
                    n1346 = local write "TEMP update"(TRUE) -> ()
                    n1347 = call "sub vi - GET ALL TEMP v3.vi"("LA01-EN"=w2146, "LA02-EN"=w2146, "LA03-EN"=w2146, "LA04-EN"=w2145, "LA05-EN"=w2145, "Gen Cal Value"=1.0) -> ("LA01 TEMP"=w2144:T17, "LA02 TEMP"=w2142:T17, "LA03 TEMP"=w2141:T17)  [unwired: 4 in, 3 out]
                    n1348 = local write "LAB03 TEMP"(w2141) -> ()
                    n1349 = local write "LAB02 TEMP"(w2142) -> ()
                    n1350 = local write "LAB01 TEMP"(w2144) -> ()
                  }
                }
                n1351 = case shown="True" w2128 {
                  frame False {
                  }
                  frame True {
                    w2138 = TRUE
                    w2139 = FALSE
                    n1352 = local write "TEMP update"(TRUE) -> ()
                    n1353 = call "sub vi - GET ALL TEMP v3.vi"("LA01-EN"=w2139, "LA02-EN"=w2139, "LA03-EN"=w2139, "LA04-EN"=w2138, "LA05-EN"=w2138, "Gen Cal Value"=1.0) -> ("LA04 TEMP"=w2136:T17, "LA05 TEMP"=w2135:T17)  [unwired: 4 in, 4 out]
                    n1354 = local write "LAB04 TEMP"(w2136) -> ()
                    n1355 = local write "LAB05 TEMP"(w2135) -> ()
                  }
                }
              }
              frame #1 {
                n1356 = local read "LAB01 (CAL)"() -> (w2164:T6)
                n1357 = local read "LAB01 TEMP"() -> (w2165:T9)
                n1358 = Unbundle By Name(w2165) -> ("T1 Live"=w2155:dbl, "T1 Neut"=w2154:dbl, "T2 Live"=w2153:dbl, "T2 Neut"=w2152:dbl)  [unwired: 2 out]
                n1359 = Unbundle By Name(w2164) -> ("1 (TL) cal"=w2151:dbl, "1 (TN) cal"=w2150:dbl, "2 (TL) cal"=w2149:dbl, "2 (TN) cal"=w2148:dbl)  [unwired: 6 out]
                n1360 = Multiply(x=w2155, y=w2151) -> (x*y=w2161:dbl)
                n1361 = Multiply(x=w2154, y=w2150) -> (x*y=w2160:dbl)
                n1362 = Multiply(x=w2153, y=w2149) -> (x*y=w2157:dbl)
                n1363 = Multiply(x=w2152, y=w2148) -> (x*y=w2156:dbl)
                n1364 = local read "LAB01-2 (SIG)"() -> (w2159:T2)
                n1365 = local read "LAB01-1 (SIG)"() -> (w2163:T2)
                n1366 = Bundle By Name(cluster=w2163, "Tmp Live"=w2161, "Tmp Neut"=w2160) -> (w2162:T2)
                n1367 = Bundle By Name(cluster=w2159, "Tmp Live"=w2157, "Tmp Neut"=w2156) -> (w2158:T2)
                n1368 = local write "LAB01-1 (SIG)"(w2162) -> ()
                n1369 = local write "LAB01-2 (SIG)"(w2158) -> ()
              }
              frame #2 {
                n1370 = local read "LAB02 (CAL)"() -> (w2182:T7)
                n1371 = local read "LAB02 TEMP"() -> (w2183:T9)
                n1372 = Unbundle By Name(w2183) -> ("T1 Live"=w2173:dbl, "T1 Neut"=w2172:dbl, "T2 Live"=w2171:dbl, "T2 Neut"=w2170:dbl)  [unwired: 2 out]
                n1373 = Unbundle By Name(w2182) -> ("1 (TL) cal"=w2169:dbl, "1 (TN) cal"=w2168:dbl, "2 (TL) cal"=w2167:dbl, "2 (TN) cal"=w2166:dbl)  [unwired: 6 out]
                n1374 = Multiply(x=w2173, y=w2169) -> (x*y=w2179:dbl)
                n1375 = Multiply(x=w2172, y=w2168) -> (x*y=w2178:dbl)
                n1376 = Multiply(x=w2171, y=w2167) -> (x*y=w2175:dbl)
                n1377 = Multiply(x=w2170, y=w2166) -> (x*y=w2174:dbl)
                n1378 = local read "LAB02-2 (SIG)"() -> (w2177:T2)
                n1379 = local read "LAB02-1 (SIG)"() -> (w2181:T2)
                n1380 = Bundle By Name(cluster=w2181, "Tmp Live"=w2179, "Tmp Neut"=w2178) -> (w2180:T2)
                n1381 = Bundle By Name(cluster=w2177, "Tmp Live"=w2175, "Tmp Neut"=w2174) -> (w2176:T2)
                n1382 = local write "LAB02-1 (SIG)"(w2180) -> ()
                n1383 = local write "LAB02-2 (SIG)"(w2176) -> ()
              }
              frame #3 {
                n1384 = local read "LAB03 (CAL)"() -> (w2200:T6)
                n1385 = local read "LAB03 TEMP"() -> (w2201:T9)
                n1386 = Unbundle By Name(w2201) -> ("T1 Live"=w2191:dbl, "T1 Neut"=w2190:dbl, "T2 Live"=w2189:dbl, "T2 Neut"=w2188:dbl)  [unwired: 2 out]
                n1387 = Unbundle By Name(w2200) -> ("1 (TL) cal"=w2187:dbl, "1 (TN) cal"=w2186:dbl, "2 (TL) cal"=w2185:dbl, "2 (TN) cal"=w2184:dbl)  [unwired: 6 out]
                n1388 = Multiply(x=w2191, y=w2187) -> (x*y=w2197:dbl)
                n1389 = Multiply(x=w2190, y=w2186) -> (x*y=w2196:dbl)
                n1390 = Multiply(x=w2189, y=w2185) -> (x*y=w2193:dbl)
                n1391 = Multiply(x=w2188, y=w2184) -> (x*y=w2192:dbl)
                n1392 = local read "LAB03-2 (SIG)"() -> (w2195:T2)
                n1393 = local read "LAB03-1 (SIG)"() -> (w2199:T2)
                n1394 = Bundle By Name(cluster=w2199, "Tmp Live"=w2197, "Tmp Neut"=w2196) -> (w2198:T2)
                n1395 = Bundle By Name(cluster=w2195, "Tmp Live"=w2193, "Tmp Neut"=w2192) -> (w2194:T2)
                n1396 = local write "LAB03-1 (SIG)"(w2198) -> ()
                n1397 = local write "LAB03-2 (SIG)"(w2194) -> ()
              }
              frame #4 {
                n1398 = local read "LAB04 (CAL)"() -> (w2218:T6)
                n1399 = local read "LAB04 TEMP"() -> (w2219:T9)
                n1400 = Unbundle By Name(w2219) -> ("T1 Live"=w2209:dbl, "T1 Neut"=w2208:dbl, "T2 Live"=w2207:dbl, "T2 Neut"=w2206:dbl)  [unwired: 2 out]
                n1401 = Unbundle By Name(w2218) -> ("1 (TL) cal"=w2205:dbl, "1 (TN) cal"=w2204:dbl, "2 (TL) cal"=w2203:dbl, "2 (TN) cal"=w2202:dbl)  [unwired: 6 out]
                n1402 = Multiply(x=w2209, y=w2205) -> (x*y=w2215:dbl)
                n1403 = Multiply(x=w2208, y=w2204) -> (x*y=w2214:dbl)
                n1404 = Multiply(x=w2207, y=w2203) -> (x*y=w2211:dbl)
                n1405 = Multiply(x=w2206, y=w2202) -> (x*y=w2210:dbl)
                n1406 = local read "LAB04-2 (SIG)"() -> (w2213:T2)
                n1407 = local read "LAB04-1 (SIG)"() -> (w2217:T2)
                n1408 = Bundle By Name(cluster=w2217, "Tmp Live"=w2215, "Tmp Neut"=w2214) -> (w2216:T2)
                n1409 = Bundle By Name(cluster=w2213, "Tmp Live"=w2211, "Tmp Neut"=w2210) -> (w2212:T2)
                n1410 = local write "LAB04-1 (SIG)"(w2216) -> ()
                n1411 = local write "LAB04-2 (SIG)"(w2212) -> ()
              }
              frame #5 {
                n1412 = local read "LAB05 (CAL)"() -> (w2236:T6)
                n1413 = local read "LAB05 TEMP"() -> (w2237:T9)
                n1414 = Unbundle By Name(w2237) -> ("T1 Live"=w2227:dbl, "T1 Neut"=w2226:dbl, "T2 Live"=w2225:dbl, "T2 Neut"=w2224:dbl)  [unwired: 2 out]
                n1415 = Unbundle By Name(w2236) -> ("1 (TL) cal"=w2223:dbl, "1 (TN) cal"=w2222:dbl, "2 (TL) cal"=w2221:dbl, "2 (TN) cal"=w2220:dbl)  [unwired: 6 out]
                n1416 = Multiply(x=w2227, y=w2223) -> (x*y=w2233:dbl)
                n1417 = Multiply(x=w2226, y=w2222) -> (x*y=w2232:dbl)
                n1418 = Multiply(x=w2225, y=w2221) -> (x*y=w2229:dbl)
                n1419 = Multiply(x=w2224, y=w2220) -> (x*y=w2228:dbl)
                n1420 = local read "LAB05-2 (SIG)"() -> (w2231:T2)
                n1421 = local read "LAB05-1 (SIG)"() -> (w2235:T2)
                n1422 = Bundle By Name(cluster=w2235, "Tmp Live"=w2233, "Tmp Neut"=w2232) -> (w2234:T2)
                n1423 = Bundle By Name(cluster=w2231, "Tmp Live"=w2229, "Tmp Neut"=w2228) -> (w2230:T2)
                n1424 = local write "LAB05-1 (SIG)"(w2234) -> ()
                n1425 = local write "LAB05-2 (SIG)"(w2230) -> ()
              }
            }
          }
          frame #11 {
            # "get analog values"
            n1426 = local read "on loops"() -> (w2244:dbl)
            n1427 = local read "jig cycle"() -> (w2241:dbl)
            n1428 = Add(x=w2244, y=1) -> (x+y=w2242:dbl)
            n1429 = Equal?(x=w2241, y=1) -> (x = y?=w2239:bool)
            n1430 = Equal?(x=w2241, y=w2242) -> (x = y?=w2240:bool)
            n1431 = Or(x=w2239, y=w2240) -> (x .or. y?=w2238:bool)
            n1432 = case shown="True" w2238 {
              frame False {
              }
              frame True {
                n1433 = call "sub vi - Read Analog All v8.vi"() -> ("Analog loop time"=w2252:dbl, "array GRAPH"=w2251:dynamicdata[], "LAB01"=w2250:T18, "LAB02"=w2249:T19, "LAB03"=w2248:T20, "LAB04"=w2247:T21, "array ERROR"=w2253:errorcluster[], "LAB05"=w2246:T22)  [unwired: 8 in]
                n1434 = stacked-sequence {
                  tunnel: w2253 -> [w2256 _ _ _ _ _]
                  tunnel: w2252 -> [w2255 _ _ _ _ _]
                  tunnel: w2251 -> [w2254 _ _ _ _ _]
                  tunnel: w2250 -> [_ w2301 _ _ _ _]
                  tunnel: w2249 -> [_ _ w2302 _ _ _]
                  tunnel: w2248 -> [_ _ _ w2326 _ _]
                  tunnel: w2247 -> [_ _ _ _ w2350 _]
                  tunnel: w2246 -> [_ _ _ _ _ w2374]
                  frame #0 {
                    n1435 = local write "AI update"(TRUE) -> ()
                    n1436 = Index Array(array=w2254, index=6) -> (element=→"LAB04-1 (GRAPH)":dynamicdata)
                    n1437 = Index Array(array=w2254, index=7) -> (element=→"LAB04-2 (GRAPH)":dynamicdata)
                    n1438 = Index Array(array=w2254, index=9) -> (element=→"LAB05-2 (GRAPH)":dynamicdata)
                    n1439 = Index Array(array=w2254, index=8) -> (element=→"LAB05-1 (GRAPH)":dynamicdata)
                    n1440 = Index Array(array=w2254, index=5) -> (element=→"LAB03-2 (GRAPH)":dynamicdata)
                    n1441 = Index Array(array=w2254, index=0) -> (element=→"LAB01-1 (GRAPH)":dynamicdata)
                    n1442 = Index Array(array=w2254, index=1) -> (element=→"LAB01-2 (GRAPH)":dynamicdata)
                    n1443 = Index Array(array=w2254, index=2) -> (element=→"LAB02-1 (GRAPH)":dynamicdata)
                    n1444 = Index Array(array=w2254, index=3) -> (element=→"LAB02-2 (GRAPH)":dynamicdata)
                    n1445 = Index Array(array=w2254, index=4) -> (element=→"LAB03-1 (GRAPH)":dynamicdata)
                    "AI loop time" <- w2255
                    "Analog Error Array" <- w2256
                  }
                  frame #1 {
                    n1446 = local read "LAB01 (CAL)"() -> (w2300:T6)
                    n1447 = Unbundle By Name(w2301) -> ("LAB01-1 (A)"=w2299:dbl, "LAB01-1 (V)"=w2298:dbl, "LAB01-1 (PF)"=w2297:dbl, "LAB01-2 (A)"=w2296:dbl, "LAB01-2 (V)"=w2295:dbl, "LAB01-2 (PF)"=w2294:dbl)
                    n1448 = Unbundle By Name(w2300) -> ("1  (A) cal"=w2293:dbl, "1 (V) cal"=w2292:dbl, "1 (PF) cal"=w2291:dbl, "2 (A) cal"=w2290:dbl, "2 (V) cal"=w2289:dbl, "2 (PF) cal"=w2288:dbl)  [unwired: 4 out]
                    n1449 = Multiply(x=w2299, y=w2293) -> (x*y=w2286:dbl)
                    n1450 = Multiply(x=w2298, y=w2292) -> (x*y=w2285:dbl)
                    n1451 = Multiply(x=w2297, y=w2291) -> (x*y=w2284:dbl)
                    n1452 = Multiply(x=w2296, y=w2290) -> (x*y=w2280:dbl)
                    n1453 = local read "LAB01-1 (SIG)"() -> (w2287:T2)
                    n1454 = Multiply(x=w2295, y=w2289) -> (x*y=w2279:dbl)
                    n1455 = Multiply(x=w2294, y=w2288) -> (x*y=w2278:dbl)
                    n1456 = local read "LAB01-2 (SIG)"() -> (w2282:T2)
                    n1457 = Bundle By Name(cluster=w2287, "AMPS"=w2286, "VOLTS"=w2285, "PF"=w2284) -> (w2283:T2)
                    n1458 = Bundle By Name(cluster=w2282, "AMPS"=w2280, "VOLTS"=w2279, "PF"=w2278) -> (w2281:T2)
                    n1459 = local write "LAB01-2 (SIG)"(w2281) -> ()
                    n1460 = local write "LAB01-1 (SIG)"(w2283) -> ()
                  }
                  frame #2 {
                    n1461 = local read "LAB02 (CAL)"() -> (w2325:T7)
                    n1462 = Unbundle By Name(w2302) -> ("LAB02-1 (A)"=w2324:dbl, "LAB02-1 (V)"=w2323:dbl, "LAB02-1 (PF)"=w2322:dbl, "LAB02-2 (A)"=w2321:dbl, "LAB02-2 (V)"=w2320:dbl, "LAB02-2 (PF)"=w2319:dbl)
                    n1463 = Unbundle By Name(w2325) -> ("1 (A) cal"=w2318:dbl, "1 (V) cal"=w2317:dbl, "1 (PF) cal"=w2316:dbl, "2 (A) cal"=w2315:dbl, "2 (V) cal"=w2314:dbl, "2 (PF) cal"=w2313:dbl)  [unwired: 4 out]
                    n1464 = Multiply(x=w2324, y=w2318) -> (x*y=w2311:dbl)
                    n1465 = Multiply(x=w2323, y=w2317) -> (x*y=w2310:dbl)
                    n1466 = Multiply(x=w2322, y=w2316) -> (x*y=w2309:dbl)
                    n1467 = Multiply(x=w2321, y=w2315) -> (x*y=w2305:dbl)
                    n1468 = local read "LAB02-1 (SIG)"() -> (w2312:T2)
                    n1469 = Multiply(x=w2320, y=w2314) -> (x*y=w2304:dbl)
                    n1470 = Multiply(x=w2319, y=w2313) -> (x*y=w2303:dbl)
                    n1471 = local read "LAB02-2 (SIG)"() -> (w2307:T2)
                    n1472 = Bundle By Name(cluster=w2312, "AMPS"=w2311, "VOLTS"=w2310, "PF"=w2309) -> (w2308:T2)
                    n1473 = Bundle By Name(cluster=w2307, "AMPS"=w2305, "VOLTS"=w2304, "PF"=w2303) -> (w2306:T2)
                    n1474 = local write "LAB02-2 (SIG)"(w2306) -> ()
                    n1475 = local write "LAB02-1 (SIG)"(w2308) -> ()
                  }
                  frame #3 {
                    n1476 = local read "LAB03 (CAL)"() -> (w2349:T6)
                    n1477 = Unbundle By Name(w2326) -> ("LAB03-1 (A)"=w2348:dbl, "LAB03-1 (V)"=w2347:dbl, "LAB03-1 (PF)"=w2346:dbl, "LAB03-2 (A)"=w2345:dbl, "LAB03-2 (V)"=w2344:dbl, "LAB03-2 (PF)"=w2343:dbl)
                    n1478 = Unbundle By Name(w2349) -> ("1  (A) cal"=w2342:dbl, "1 (V) cal"=w2341:dbl, "1 (PF) cal"=w2340:dbl, "2 (A) cal"=w2339:dbl, "2 (V) cal"=w2338:dbl, "2 (PF) cal"=w2337:dbl)  [unwired: 4 out]
                    n1479 = Multiply(x=w2348, y=w2342) -> (x*y=w2335:dbl)
                    n1480 = Multiply(x=w2347, y=w2341) -> (x*y=w2334:dbl)
                    n1481 = Multiply(x=w2346, y=w2340) -> (x*y=w2333:dbl)
                    n1482 = Multiply(x=w2345, y=w2339) -> (x*y=w2329:dbl)
                    n1483 = local read "LAB03-1 (SIG)"() -> (w2336:T2)
                    n1484 = Multiply(x=w2344, y=w2338) -> (x*y=w2328:dbl)
                    n1485 = Multiply(x=w2343, y=w2337) -> (x*y=w2327:dbl)
                    n1486 = local read "LAB03-1 (SIG)"() -> (w2331:T2)
                    n1487 = Bundle By Name(cluster=w2336, "AMPS"=w2335, "VOLTS"=w2334, "PF"=w2333) -> (w2332:T2)
                    n1488 = Bundle By Name(cluster=w2331, "AMPS"=w2329, "VOLTS"=w2328, "PF"=w2327) -> (w2330:T2)
                    n1489 = local write "LAB03-1 (SIG)"(w2330) -> ()
                    n1490 = local write "LAB03-1 (SIG)"(w2332) -> ()
                  }
                  frame #4 {
                    n1491 = local read "LAB04 (CAL)"() -> (w2373:T6)
                    n1492 = Unbundle By Name(w2350) -> ("LAB04-1 (A)"=w2372:dbl, "LAB04-1 (V)"=w2371:dbl, "LAB04-1 (PF)"=w2370:dbl, "LAB04-2 (A)"=w2369:dbl, "LAB04-2 (V)"=w2368:dbl, "LAB04-2 (PF)"=w2367:dbl)
                    n1493 = Unbundle By Name(w2373) -> ("1  (A) cal"=w2366:dbl, "1 (V) cal"=w2365:dbl, "1 (PF) cal"=w2364:dbl, "2 (A) cal"=w2363:dbl, "2 (V) cal"=w2362:dbl, "2 (PF) cal"=w2361:dbl)  [unwired: 4 out]
                    n1494 = Multiply(x=w2372, y=w2366) -> (x*y=w2359:dbl)
                    n1495 = Multiply(x=w2371, y=w2365) -> (x*y=w2358:dbl)
                    n1496 = Multiply(x=w2370, y=w2364) -> (x*y=w2357:dbl)
                    n1497 = Multiply(x=w2369, y=w2363) -> (x*y=w2353:dbl)
                    n1498 = local read "LAB04-1 (SIG)"() -> (w2360:T2)
                    n1499 = Multiply(x=w2368, y=w2362) -> (x*y=w2352:dbl)
                    n1500 = Multiply(x=w2367, y=w2361) -> (x*y=w2351:dbl)
                    n1501 = local read "LAB04-2 (SIG)"() -> (w2355:T2)
                    n1502 = Bundle By Name(cluster=w2360, "AMPS"=w2359, "VOLTS"=w2358, "PF"=w2357) -> (w2356:T2)
                    n1503 = Bundle By Name(cluster=w2355, "AMPS"=w2353, "VOLTS"=w2352, "PF"=w2351) -> (w2354:T2)
                    n1504 = local write "LAB04-2 (SIG)"(w2354) -> ()
                    n1505 = local write "LAB04-1 (SIG)"(w2356) -> ()
                  }
                  frame #5 {
                    n1506 = local read "LAB05 (CAL)"() -> (w2397:T6)
                    n1507 = Unbundle By Name(w2374) -> ("LAB05-1 (A)"=w2396:dbl, "LAB05-1 (V)"=w2395:dbl, "LAB05-1 (PF)"=w2394:dbl, "LAB05-2 (A)"=w2393:dbl, "LAB05-2 (V)"=w2392:dbl, "LAB05-2 (PF)"=w2391:dbl)
                    n1508 = Unbundle By Name(w2397) -> ("1  (A) cal"=w2390:dbl, "1 (V) cal"=w2389:dbl, "1 (PF) cal"=w2388:dbl, "2 (A) cal"=w2387:dbl, "2 (V) cal"=w2386:dbl, "2 (PF) cal"=w2385:dbl)  [unwired: 4 out]
                    n1509 = Multiply(x=w2396, y=w2390) -> (x*y=w2383:dbl)
                    n1510 = Multiply(x=w2395, y=w2389) -> (x*y=w2382:dbl)
                    n1511 = Multiply(x=w2394, y=w2388) -> (x*y=w2381:dbl)
                    n1512 = Multiply(x=w2393, y=w2387) -> (x*y=w2377:dbl)
                    n1513 = local read "LAB05-1 (SIG)"() -> (w2384:T2)
                    n1514 = Multiply(x=w2392, y=w2386) -> (x*y=w2376:dbl)
                    n1515 = Multiply(x=w2391, y=w2385) -> (x*y=w2375:dbl)
                    n1516 = local read "LAB05-2 (SIG)"() -> (w2379:T2)
                    n1517 = Bundle By Name(cluster=w2384, "AMPS"=w2383, "VOLTS"=w2382, "PF"=w2381) -> (w2380:T2)
                    n1518 = Bundle By Name(cluster=w2379, "AMPS"=w2377, "VOLTS"=w2376, "PF"=w2375) -> (w2378:T2)
                    n1519 = local write "LAB05-2 (SIG)"(w2378) -> ()
                    n1520 = local write "LAB05-1 (SIG)"(w2380) -> ()
                  }
                }
              }
            }
          }
          frame #12 {
            # "save test data to file"
            n1521 = local read "on loops"() -> (w2414:dbl)
            n1522 = local read "jig cycle"() -> (w2411:dbl)
            n1523 = Add(x=w2414, y=2) -> (x+y=w2412:dbl)
            n1524 = Equal?(x=w2411, y=1) -> (x = y?=w2409:bool)
            n1525 = Equal?(x=w2411, y=w2412) -> (x = y?=w2410:bool)
            n1526 = Or(x=w2409, y=w2410) -> (x .or. y?=w2408:bool)
            n1527 = case shown="True" w2408 {
              tunnel: w2407 -> [_ w2425]
              tunnel: w2406 -> [_ w2424]
              tunnel: w2405 -> [_ w2423]
              tunnel: w2404 -> [_ w2422]
              tunnel: w2403 -> [_ w2421]
              tunnel: w2402 -> [_ w2420]
              tunnel: w2401 -> [_ w2419]
              tunnel: w2400 -> [_ w2418]
              tunnel: w2399 -> [_ w2417]
              tunnel: w2398 -> [_ w2416]
              frame False {
              }
              frame True {
                n1528 = stacked-sequence {
                  tunnel: w2425 -> [w2426 _ _ _ _ _ _ _ _ _]
                  tunnel: w2424 -> [_ w2471 _ _ _ _ _ _ _ _]
                  tunnel: w2423 -> [_ _ w2516 _ _ _ _ _ _ _]
                  tunnel: w2422 -> [_ _ _ w2561 _ _ _ _ _ _]
                  tunnel: w2421 -> [_ _ _ _ w2606 _ _ _ _ _]
                  tunnel: w2420 -> [_ _ _ _ _ w2651 _ _ _ _]
                  tunnel: w2419 -> [_ _ _ _ _ _ w2696 _ _ _]
                  tunnel: w2418 -> [_ _ _ _ _ _ _ w2741 _ _]
                  tunnel: w2417 -> [_ _ _ _ _ _ _ _ w2786 _]
                  tunnel: w2416 -> [_ _ _ _ _ _ _ _ _ w2831]
                  frame #0 {
                    # "LAB01-1"
                    n1529 = case shown="True" w2426 {
                      frame False {
                      }
                      frame True {
                        n1530 = local read "LAB01-1 (DISP)"() -> (w2468:T4)
                        n1531 = local read "LAB01-1 (SIG)"() -> (w2469:T2)
                        n1532 = local read "LAB01-1 (TDMS)"() -> (w2470:refnum<k34>)
                        n1533 = Build Array("TEMP Neut") -> (w2434:string[])
                        n1534 = Build Array("CYCLE") -> (w2429:string[])
                        n1535 = Build Array("TEMP Live") -> (w2439:string[])
                        n1536 = Build Array("PF") -> (w2444:string[])
                        n1537 = Build Array("AMPS") -> (w2465:string[])
                        n1538 = Build Array("VOLTS") -> (w2456:string[])
                        n1539 = Unbundle(w2469) -> ("AMPS"=w2464:dbl, "VOLTS"=w2453:dbl, "PF"=w2452:dbl, "Tmp Live"=w2451:dbl, "Tmp Neut"=w2454:dbl)
                        n1540 = Unbundle(w2468) -> ("CYCLE"=w2449:dbl)  [unwired: 2 out]
                        n1541 = Build Array(w2453) -> (w2450:dbl[])
                        n1542 = Build Array(w2452) -> (w2443:dbl[])
                        n1543 = Build Array(w2451) -> (w2438:dbl[])
                        n1544 = Build Array(w2454) -> (w2433:dbl[])
                        n1545 = Build Array(w2464) -> (w2463:dbl[])
                        n1546 = Build Array(w2449) -> (w2428:dbl[])
                        n1547 = TDMS Write(0:w2470, 5:"LAB01-1 TEST VALUES", 7:w2465, 9:w2463) -> (4:w2458:refnum<k34>, 6:w2457:string, 15:w2445:errorcluster)  [unwired: 2 in, 1 out]
                        n1548 = TDMS Write(0:w2458, 5:w2457, 7:w2456, 9:w2450, 11:w2445) -> (4:w2448:refnum<k34>, 6:w2447:string, 15:w2446:errorcluster)  [unwired: 1 in, 1 out]
                        n1549 = TDMS Write(0:w2448, 5:w2447, 7:w2444, 9:w2443, 11:w2446) -> (4:w2442:refnum<k34>, 6:w2441:string, 15:w2440:errorcluster)  [unwired: 1 in, 1 out]
                        n1550 = TDMS Write(0:w2442, 5:w2441, 7:w2439, 9:w2438, 11:w2440) -> (4:w2437:refnum<k34>, 6:w2436:string, 15:w2435:errorcluster)  [unwired: 1 in, 1 out]
                        n1551 = TDMS Write(0:w2437, 5:w2436, 7:w2434, 9:w2433, 11:w2435) -> (4:w2432:refnum<k34>, 6:w2431:string, 15:w2430:errorcluster)  [unwired: 1 in, 1 out]
                        n1552 = TDMS Write(0:w2432, 5:w2431, 7:w2429, 9:w2428, 11:w2430) -> (15:w2427:errorcluster)  [unwired: 1 in, 3 out]
                        n1553 = local write "data file error"(w2427) -> ()
                      }
                    }
                  }
                  frame #1 {
                    # "LAB01-2"
                    n1554 = case shown="True" w2471 {
                      frame False {
                      }
                      frame True {
                        n1555 = local read "LAB01-2 (DISP)"() -> (w2513:T4)
                        n1556 = local read "LAB01-2 (SIG)"() -> (w2514:T2)
                        n1557 = local read "LAB01-2 (TDMS)"() -> (w2515:refnum<k34>)
                        n1558 = Build Array("TEMP Neut") -> (w2479:string[])
                        n1559 = Build Array("CYCLE") -> (w2474:string[])
                        n1560 = Build Array("TEMP Live") -> (w2484:string[])
                        n1561 = Build Array("PF") -> (w2489:string[])
                        n1562 = Build Array("AMPS") -> (w2510:string[])
                        n1563 = Build Array("VOLTS") -> (w2501:string[])
                        n1564 = Unbundle(w2514) -> ("AMPS"=w2509:dbl, "VOLTS"=w2498:dbl, "PF"=w2497:dbl, "Tmp Live"=w2496:dbl, "Tmp Neut"=w2499:dbl)
                        n1565 = Unbundle(w2513) -> ("CYCLE"=w2494:dbl)  [unwired: 2 out]
                        n1566 = Build Array(w2498) -> (w2495:dbl[])
                        n1567 = Build Array(w2497) -> (w2488:dbl[])
                        n1568 = Build Array(w2496) -> (w2483:dbl[])
                        n1569 = Build Array(w2499) -> (w2478:dbl[])
                        n1570 = Build Array(w2509) -> (w2508:dbl[])
                        n1571 = Build Array(w2494) -> (w2473:dbl[])
                        n1572 = TDMS Write(0:w2515, 5:"LAB01-2 TEST VALUES", 7:w2510, 9:w2508) -> (4:w2503:refnum<k34>, 6:w2502:string, 15:w2490:errorcluster)  [unwired: 2 in, 1 out]
                        n1573 = TDMS Write(0:w2503, 5:w2502, 7:w2501, 9:w2495, 11:w2490) -> (4:w2493:refnum<k34>, 6:w2492:string, 15:w2491:errorcluster)  [unwired: 1 in, 1 out]
                        n1574 = TDMS Write(0:w2493, 5:w2492, 7:w2489, 9:w2488, 11:w2491) -> (4:w2487:refnum<k34>, 6:w2486:string, 15:w2485:errorcluster)  [unwired: 1 in, 1 out]
                        n1575 = TDMS Write(0:w2487, 5:w2486, 7:w2484, 9:w2483, 11:w2485) -> (4:w2482:refnum<k34>, 6:w2481:string, 15:w2480:errorcluster)  [unwired: 1 in, 1 out]
                        n1576 = TDMS Write(0:w2482, 5:w2481, 7:w2479, 9:w2478, 11:w2480) -> (4:w2477:refnum<k34>, 6:w2476:string, 15:w2475:errorcluster)  [unwired: 1 in, 1 out]
                        n1577 = TDMS Write(0:w2477, 5:w2476, 7:w2474, 9:w2473, 11:w2475) -> (15:w2472:errorcluster)  [unwired: 1 in, 3 out]
                        n1578 = local write "data file error"(w2472) -> ()
                      }
                    }
                  }
                  frame #2 {
                    # "LAB02-1"
                    n1579 = case shown="True" w2516 {
                      frame False {
                      }
                      frame True {
                        n1580 = local read "LAB02-1 (DISP)"() -> (w2558:T4)
                        n1581 = local read "LAB02-1 (SIG)"() -> (w2559:T2)
                        n1582 = local read "LAB02-1 (TDMS)"() -> (w2560:refnum<k34>)
                        n1583 = Build Array("TEMP Neut") -> (w2524:string[])
                        n1584 = Build Array("CYCLE") -> (w2519:string[])
                        n1585 = Build Array("TEMP Live") -> (w2529:string[])
                        n1586 = Build Array("PF") -> (w2534:string[])
                        n1587 = Build Array("AMPS") -> (w2555:string[])
                        n1588 = Build Array("VOLTS") -> (w2546:string[])
                        n1589 = Unbundle(w2559) -> ("AMPS"=w2554:dbl, "VOLTS"=w2543:dbl, "PF"=w2542:dbl, "Tmp Live"=w2541:dbl, "Tmp Neut"=w2544:dbl)
                        n1590 = Unbundle(w2558) -> ("CYCLE"=w2539:dbl)  [unwired: 2 out]
                        n1591 = Build Array(w2543) -> (w2540:dbl[])
                        n1592 = Build Array(w2542) -> (w2533:dbl[])
                        n1593 = Build Array(w2541) -> (w2528:dbl[])
                        n1594 = Build Array(w2544) -> (w2523:dbl[])
                        n1595 = Build Array(w2554) -> (w2553:dbl[])
                        n1596 = Build Array(w2539) -> (w2518:dbl[])
                        n1597 = TDMS Write(0:w2560, 5:"LAB02-1 TEST VALUES", 7:w2555, 9:w2553) -> (4:w2548:refnum<k34>, 6:w2547:string, 15:w2535:errorcluster)  [unwired: 2 in, 1 out]
                        n1598 = TDMS Write(0:w2548, 5:w2547, 7:w2546, 9:w2540, 11:w2535) -> (4:w2538:refnum<k34>, 6:w2537:string, 15:w2536:errorcluster)  [unwired: 1 in, 1 out]
                        n1599 = TDMS Write(0:w2538, 5:w2537, 7:w2534, 9:w2533, 11:w2536) -> (4:w2532:refnum<k34>, 6:w2531:string, 15:w2530:errorcluster)  [unwired: 1 in, 1 out]
                        n1600 = TDMS Write(0:w2532, 5:w2531, 7:w2529, 9:w2528, 11:w2530) -> (4:w2527:refnum<k34>, 6:w2526:string, 15:w2525:errorcluster)  [unwired: 1 in, 1 out]
                        n1601 = TDMS Write(0:w2527, 5:w2526, 7:w2524, 9:w2523, 11:w2525) -> (4:w2522:refnum<k34>, 6:w2521:string, 15:w2520:errorcluster)  [unwired: 1 in, 1 out]
                        n1602 = TDMS Write(0:w2522, 5:w2521, 7:w2519, 9:w2518, 11:w2520) -> (15:w2517:errorcluster)  [unwired: 1 in, 3 out]
                        n1603 = local write "data file error"(w2517) -> ()
                      }
                    }
                  }
                  frame #3 {
                    # "LAB02-2"
                    n1604 = case shown="True" w2561 {
                      frame False {
                      }
                      frame True {
                        n1605 = local read "LAB02-2 (DISP)"() -> (w2603:T4)
                        n1606 = local read "LAB02-2 (SIG)"() -> (w2604:T2)
                        n1607 = local read "LAB02-2 (TDMS)"() -> (w2605:refnum<k34>)
                        n1608 = Build Array("TEMP Neut") -> (w2569:string[])
                        n1609 = Build Array("CYCLE") -> (w2564:string[])
                        n1610 = Build Array("TEMP Live") -> (w2574:string[])
                        n1611 = Build Array("PF") -> (w2579:string[])
                        n1612 = Build Array("AMPS") -> (w2600:string[])
                        n1613 = Build Array("VOLTS") -> (w2591:string[])
                        n1614 = Unbundle(w2604) -> ("AMPS"=w2599:dbl, "VOLTS"=w2588:dbl, "PF"=w2587:dbl, "Tmp Live"=w2586:dbl, "Tmp Neut"=w2589:dbl)
                        n1615 = Unbundle(w2603) -> ("CYCLE"=w2584:dbl)  [unwired: 2 out]
                        n1616 = Build Array(w2588) -> (w2585:dbl[])
                        n1617 = Build Array(w2587) -> (w2578:dbl[])
                        n1618 = Build Array(w2586) -> (w2573:dbl[])
                        n1619 = Build Array(w2589) -> (w2568:dbl[])
                        n1620 = Build Array(w2599) -> (w2598:dbl[])
                        n1621 = Build Array(w2584) -> (w2563:dbl[])
                        n1622 = TDMS Write(0:w2605, 5:"LAB02-2 TEST VALUES", 7:w2600, 9:w2598) -> (4:w2593:refnum<k34>, 6:w2592:string, 15:w2580:errorcluster)  [unwired: 2 in, 1 out]
                        n1623 = TDMS Write(0:w2593, 5:w2592, 7:w2591, 9:w2585, 11:w2580) -> (4:w2583:refnum<k34>, 6:w2582:string, 15:w2581:errorcluster)  [unwired: 1 in, 1 out]
                        n1624 = TDMS Write(0:w2583, 5:w2582, 7:w2579, 9:w2578, 11:w2581) -> (4:w2577:refnum<k34>, 6:w2576:string, 15:w2575:errorcluster)  [unwired: 1 in, 1 out]
                        n1625 = TDMS Write(0:w2577, 5:w2576, 7:w2574, 9:w2573, 11:w2575) -> (4:w2572:refnum<k34>, 6:w2571:string, 15:w2570:errorcluster)  [unwired: 1 in, 1 out]
                        n1626 = TDMS Write(0:w2572, 5:w2571, 7:w2569, 9:w2568, 11:w2570) -> (4:w2567:refnum<k34>, 6:w2566:string, 15:w2565:errorcluster)  [unwired: 1 in, 1 out]
                        n1627 = TDMS Write(0:w2567, 5:w2566, 7:w2564, 9:w2563, 11:w2565) -> (15:w2562:errorcluster)  [unwired: 1 in, 3 out]
                        n1628 = local write "data file error"(w2562) -> ()
                      }
                    }
                  }
                  frame #4 {
                    # "LAB03-1"
                    n1629 = case shown="True" w2606 {
                      frame False {
                      }
                      frame True {
                        n1630 = local read "LAB03-1 (DISP)"() -> (w2648:T4)
                        n1631 = local read "LAB03-1 (SIG)"() -> (w2649:T2)
                        n1632 = local read "LAB03-1 (TDMS)"() -> (w2650:refnum<k34>)
                        n1633 = Build Array("TEMP Neut") -> (w2614:string[])
                        n1634 = Build Array("CYCLE") -> (w2609:string[])
                        n1635 = Build Array("TEMP Live") -> (w2619:string[])
                        n1636 = Build Array("PF") -> (w2624:string[])
                        n1637 = Build Array("AMPS") -> (w2645:string[])
                        n1638 = Build Array("VOLTS") -> (w2636:string[])
                        n1639 = Unbundle(w2649) -> ("AMPS"=w2644:dbl, "VOLTS"=w2633:dbl, "PF"=w2632:dbl, "Tmp Live"=w2631:dbl, "Tmp Neut"=w2634:dbl)
                        n1640 = Unbundle(w2648) -> ("CYCLE"=w2629:dbl)  [unwired: 2 out]
                        n1641 = Build Array(w2633) -> (w2630:dbl[])
                        n1642 = Build Array(w2632) -> (w2623:dbl[])
                        n1643 = Build Array(w2631) -> (w2618:dbl[])
                        n1644 = Build Array(w2634) -> (w2613:dbl[])
                        n1645 = Build Array(w2644) -> (w2643:dbl[])
                        n1646 = Build Array(w2629) -> (w2608:dbl[])
                        n1647 = TDMS Write(0:w2650, 5:"LAB03-1 TEST VALUES", 7:w2645, 9:w2643) -> (4:w2638:refnum<k34>, 6:w2637:string, 15:w2625:errorcluster)  [unwired: 2 in, 1 out]
                        n1648 = TDMS Write(0:w2638, 5:w2637, 7:w2636, 9:w2630, 11:w2625) -> (4:w2628:refnum<k34>, 6:w2627:string, 15:w2626:errorcluster)  [unwired: 1 in, 1 out]
                        n1649 = TDMS Write(0:w2628, 5:w2627, 7:w2624, 9:w2623, 11:w2626) -> (4:w2622:refnum<k34>, 6:w2621:string, 15:w2620:errorcluster)  [unwired: 1 in, 1 out]
                        n1650 = TDMS Write(0:w2622, 5:w2621, 7:w2619, 9:w2618, 11:w2620) -> (4:w2617:refnum<k34>, 6:w2616:string, 15:w2615:errorcluster)  [unwired: 1 in, 1 out]
                        n1651 = TDMS Write(0:w2617, 5:w2616, 7:w2614, 9:w2613, 11:w2615) -> (4:w2612:refnum<k34>, 6:w2611:string, 15:w2610:errorcluster)  [unwired: 1 in, 1 out]
                        n1652 = TDMS Write(0:w2612, 5:w2611, 7:w2609, 9:w2608, 11:w2610) -> (15:w2607:errorcluster)  [unwired: 1 in, 3 out]
                        n1653 = local write "data file error"(w2607) -> ()
                      }
                    }
                  }
                  frame #5 {
                    # "LAB03-2"
                    n1654 = case shown="True" w2651 {
                      frame False {
                      }
                      frame True {
                        n1655 = local read "LAB03-2 (DISP)"() -> (w2693:T4)
                        n1656 = local read "LAB03-2 (SIG)"() -> (w2694:T2)
                        n1657 = local read "LAB03-2 (TDMS)"() -> (w2695:refnum<k34>)
                        n1658 = Build Array("TEMP Neut") -> (w2659:string[])
                        n1659 = Build Array("CYCLE") -> (w2654:string[])
                        n1660 = Build Array("TEMP Live") -> (w2664:string[])
                        n1661 = Build Array("PF") -> (w2669:string[])
                        n1662 = Build Array("AMPS") -> (w2690:string[])
                        n1663 = Build Array("VOLTS") -> (w2681:string[])
                        n1664 = Unbundle(w2694) -> ("AMPS"=w2689:dbl, "VOLTS"=w2678:dbl, "PF"=w2677:dbl, "Tmp Live"=w2676:dbl, "Tmp Neut"=w2679:dbl)
                        n1665 = Unbundle(w2693) -> ("CYCLE"=w2674:dbl)  [unwired: 2 out]
                        n1666 = Build Array(w2678) -> (w2675:dbl[])
                        n1667 = Build Array(w2677) -> (w2668:dbl[])
                        n1668 = Build Array(w2676) -> (w2663:dbl[])
                        n1669 = Build Array(w2679) -> (w2658:dbl[])
                        n1670 = Build Array(w2689) -> (w2688:dbl[])
                        n1671 = Build Array(w2674) -> (w2653:dbl[])
                        n1672 = TDMS Write(0:w2695, 5:"LAB03-2 TEST VALUES", 7:w2690, 9:w2688) -> (4:w2683:refnum<k34>, 6:w2682:string, 15:w2670:errorcluster)  [unwired: 2 in, 1 out]
                        n1673 = TDMS Write(0:w2683, 5:w2682, 7:w2681, 9:w2675, 11:w2670) -> (4:w2673:refnum<k34>, 6:w2672:string, 15:w2671:errorcluster)  [unwired: 1 in, 1 out]
                        n1674 = TDMS Write(0:w2673, 5:w2672, 7:w2669, 9:w2668, 11:w2671) -> (4:w2667:refnum<k34>, 6:w2666:string, 15:w2665:errorcluster)  [unwired: 1 in, 1 out]
                        n1675 = TDMS Write(0:w2667, 5:w2666, 7:w2664, 9:w2663, 11:w2665) -> (4:w2662:refnum<k34>, 6:w2661:string, 15:w2660:errorcluster)  [unwired: 1 in, 1 out]
                        n1676 = TDMS Write(0:w2662, 5:w2661, 7:w2659, 9:w2658, 11:w2660) -> (4:w2657:refnum<k34>, 6:w2656:string, 15:w2655:errorcluster)  [unwired: 1 in, 1 out]
                        n1677 = TDMS Write(0:w2657, 5:w2656, 7:w2654, 9:w2653, 11:w2655) -> (15:w2652:errorcluster)  [unwired: 1 in, 3 out]
                        n1678 = local write "data file error"(w2652) -> ()
                      }
                    }
                  }
                  frame #6 {
                    # "LAB04-1"
                    n1679 = case shown="True" w2696 {
                      frame False {
                      }
                      frame True {
                        n1680 = local read "LAB04-1 (DISP)"() -> (w2738:T4)
                        n1681 = local read "LAB04-1 (SIG)"() -> (w2739:T2)
                        n1682 = local read "LAB04-1 (TDMS)"() -> (w2740:refnum<k34>)
                        n1683 = Build Array("TEMP Neut") -> (w2704:string[])
                        n1684 = Build Array("CYCLE") -> (w2699:string[])
                        n1685 = Build Array("TEMP Live") -> (w2709:string[])
                        n1686 = Build Array("PF") -> (w2714:string[])
                        n1687 = Build Array("AMPS") -> (w2735:string[])
                        n1688 = Build Array("VOLTS") -> (w2726:string[])
                        n1689 = Unbundle(w2739) -> ("AMPS"=w2734:dbl, "VOLTS"=w2723:dbl, "PF"=w2722:dbl, "Tmp Live"=w2721:dbl, "Tmp Neut"=w2724:dbl)
                        n1690 = Unbundle(w2738) -> ("CYCLE"=w2719:dbl)  [unwired: 2 out]
                        n1691 = Build Array(w2723) -> (w2720:dbl[])
                        n1692 = Build Array(w2722) -> (w2713:dbl[])
                        n1693 = Build Array(w2721) -> (w2708:dbl[])
                        n1694 = Build Array(w2724) -> (w2703:dbl[])
                        n1695 = Build Array(w2734) -> (w2733:dbl[])
                        n1696 = Build Array(w2719) -> (w2698:dbl[])
                        n1697 = TDMS Write(0:w2740, 5:"LAB04-1 TEST VALUES", 7:w2735, 9:w2733) -> (4:w2728:refnum<k34>, 6:w2727:string, 15:w2715:errorcluster)  [unwired: 2 in, 1 out]
                        n1698 = TDMS Write(0:w2728, 5:w2727, 7:w2726, 9:w2720, 11:w2715) -> (4:w2718:refnum<k34>, 6:w2717:string, 15:w2716:errorcluster)  [unwired: 1 in, 1 out]
                        n1699 = TDMS Write(0:w2718, 5:w2717, 7:w2714, 9:w2713, 11:w2716) -> (4:w2712:refnum<k34>, 6:w2711:string, 15:w2710:errorcluster)  [unwired: 1 in, 1 out]
                        n1700 = TDMS Write(0:w2712, 5:w2711, 7:w2709, 9:w2708, 11:w2710) -> (4:w2707:refnum<k34>, 6:w2706:string, 15:w2705:errorcluster)  [unwired: 1 in, 1 out]
                        n1701 = TDMS Write(0:w2707, 5:w2706, 7:w2704, 9:w2703, 11:w2705) -> (4:w2702:refnum<k34>, 6:w2701:string, 15:w2700:errorcluster)  [unwired: 1 in, 1 out]
                        n1702 = TDMS Write(0:w2702, 5:w2701, 7:w2699, 9:w2698, 11:w2700) -> (15:w2697:errorcluster)  [unwired: 1 in, 3 out]
                        n1703 = local write "data file error"(w2697) -> ()
                      }
                    }
                  }
                  frame #7 {
                    # "LAB04-2"
                    n1704 = case shown="True" w2741 {
                      frame False {
                      }
                      frame True {
                        n1705 = local read "LAB04-2 (DISP)"() -> (w2783:T4)
                        n1706 = local read "LAB04-2 (SIG)"() -> (w2784:T2)
                        n1707 = local read "LAB04-2 (TDMS)"() -> (w2785:refnum<k34>)
                        n1708 = Build Array("TEMP Neut") -> (w2749:string[])
                        n1709 = Build Array("CYCLE") -> (w2744:string[])
                        n1710 = Build Array("TEMP Live") -> (w2754:string[])
                        n1711 = Build Array("PF") -> (w2759:string[])
                        n1712 = Build Array("AMPS") -> (w2780:string[])
                        n1713 = Build Array("VOLTS") -> (w2771:string[])
                        n1714 = Unbundle(w2784) -> ("AMPS"=w2779:dbl, "VOLTS"=w2768:dbl, "PF"=w2767:dbl, "Tmp Live"=w2766:dbl, "Tmp Neut"=w2769:dbl)
                        n1715 = Unbundle(w2783) -> ("CYCLE"=w2764:dbl)  [unwired: 2 out]
                        n1716 = Build Array(w2768) -> (w2765:dbl[])
                        n1717 = Build Array(w2767) -> (w2758:dbl[])
                        n1718 = Build Array(w2766) -> (w2753:dbl[])
                        n1719 = Build Array(w2769) -> (w2748:dbl[])
                        n1720 = Build Array(w2779) -> (w2778:dbl[])
                        n1721 = Build Array(w2764) -> (w2743:dbl[])
                        n1722 = TDMS Write(0:w2785, 5:"LAB04-2 TEST VALUES", 7:w2780, 9:w2778) -> (4:w2773:refnum<k34>, 6:w2772:string, 15:w2760:errorcluster)  [unwired: 2 in, 1 out]
                        n1723 = TDMS Write(0:w2773, 5:w2772, 7:w2771, 9:w2765, 11:w2760) -> (4:w2763:refnum<k34>, 6:w2762:string, 15:w2761:errorcluster)  [unwired: 1 in, 1 out]
                        n1724 = TDMS Write(0:w2763, 5:w2762, 7:w2759, 9:w2758, 11:w2761) -> (4:w2757:refnum<k34>, 6:w2756:string, 15:w2755:errorcluster)  [unwired: 1 in, 1 out]
                        n1725 = TDMS Write(0:w2757, 5:w2756, 7:w2754, 9:w2753, 11:w2755) -> (4:w2752:refnum<k34>, 6:w2751:string, 15:w2750:errorcluster)  [unwired: 1 in, 1 out]
                        n1726 = TDMS Write(0:w2752, 5:w2751, 7:w2749, 9:w2748, 11:w2750) -> (4:w2747:refnum<k34>, 6:w2746:string, 15:w2745:errorcluster)  [unwired: 1 in, 1 out]
                        n1727 = TDMS Write(0:w2747, 5:w2746, 7:w2744, 9:w2743, 11:w2745) -> (15:w2742:errorcluster)  [unwired: 1 in, 3 out]
                        n1728 = local write "data file error"(w2742) -> ()
                      }
                    }
                  }
                  frame #8 {
                    # "LAB05-1"
                    n1729 = case shown="True" w2786 {
                      frame False {
                      }
                      frame True {
                        n1730 = local read "LAB05-1 (DISP)"() -> (w2828:T4)
                        n1731 = local read "LAB05-1 (SIG)"() -> (w2829:T2)
                        n1732 = local read "LAB05-1 (TDMS)"() -> (w2830:refnum<k34>)
                        n1733 = Build Array("TEMP Neut") -> (w2794:string[])
                        n1734 = Build Array("CYCLE") -> (w2789:string[])
                        n1735 = Build Array("TEMP Live") -> (w2799:string[])
                        n1736 = Build Array("PF") -> (w2804:string[])
                        n1737 = Build Array("AMPS") -> (w2825:string[])
                        n1738 = Build Array("VOLTS") -> (w2816:string[])
                        n1739 = Unbundle(w2829) -> ("AMPS"=w2824:dbl, "VOLTS"=w2813:dbl, "PF"=w2812:dbl, "Tmp Live"=w2811:dbl, "Tmp Neut"=w2814:dbl)
                        n1740 = Unbundle(w2828) -> ("CYCLE"=w2809:dbl)  [unwired: 2 out]
                        n1741 = Build Array(w2813) -> (w2810:dbl[])
                        n1742 = Build Array(w2812) -> (w2803:dbl[])
                        n1743 = Build Array(w2811) -> (w2798:dbl[])
                        n1744 = Build Array(w2814) -> (w2793:dbl[])
                        n1745 = Build Array(w2824) -> (w2823:dbl[])
                        n1746 = Build Array(w2809) -> (w2788:dbl[])
                        n1747 = TDMS Write(0:w2830, 5:"LAB05-1 TEST VALUES", 7:w2825, 9:w2823) -> (4:w2818:refnum<k34>, 6:w2817:string, 15:w2805:errorcluster)  [unwired: 2 in, 1 out]
                        n1748 = TDMS Write(0:w2818, 5:w2817, 7:w2816, 9:w2810, 11:w2805) -> (4:w2808:refnum<k34>, 6:w2807:string, 15:w2806:errorcluster)  [unwired: 1 in, 1 out]
                        n1749 = TDMS Write(0:w2808, 5:w2807, 7:w2804, 9:w2803, 11:w2806) -> (4:w2802:refnum<k34>, 6:w2801:string, 15:w2800:errorcluster)  [unwired: 1 in, 1 out]
                        n1750 = TDMS Write(0:w2802, 5:w2801, 7:w2799, 9:w2798, 11:w2800) -> (4:w2797:refnum<k34>, 6:w2796:string, 15:w2795:errorcluster)  [unwired: 1 in, 1 out]
                        n1751 = TDMS Write(0:w2797, 5:w2796, 7:w2794, 9:w2793, 11:w2795) -> (4:w2792:refnum<k34>, 6:w2791:string, 15:w2790:errorcluster)  [unwired: 1 in, 1 out]
                        n1752 = TDMS Write(0:w2792, 5:w2791, 7:w2789, 9:w2788, 11:w2790) -> (15:w2787:errorcluster)  [unwired: 1 in, 3 out]
                        n1753 = local write "data file error"(w2787) -> ()
                      }
                    }
                  }
                  frame #9 {
                    # "LAB05-2"
                    n1754 = case shown="True" w2831 {
                      frame False {
                      }
                      frame True {
                        n1755 = local read "LAB05-2 (DISP)"() -> (w2873:T4)
                        n1756 = local read "LAB05-2 (SIG)"() -> (w2874:T2)
                        n1757 = local read "LAB05-2 (TDMS)"() -> (w2875:refnum<k34>)
                        n1758 = Build Array("TEMP Neut") -> (w2839:string[])
                        n1759 = Build Array("CYCLE") -> (w2834:string[])
                        n1760 = Build Array("TEMP Live") -> (w2844:string[])
                        n1761 = Build Array("PF") -> (w2849:string[])
                        n1762 = Build Array("AMPS") -> (w2870:string[])
                        n1763 = Build Array("VOLTS") -> (w2861:string[])
                        n1764 = Unbundle(w2874) -> ("AMPS"=w2869:dbl, "VOLTS"=w2858:dbl, "PF"=w2857:dbl, "Tmp Live"=w2856:dbl, "Tmp Neut"=w2859:dbl)
                        n1765 = Unbundle(w2873) -> ("CYCLE"=w2854:dbl)  [unwired: 2 out]
                        n1766 = Build Array(w2858) -> (w2855:dbl[])
                        n1767 = Build Array(w2857) -> (w2848:dbl[])
                        n1768 = Build Array(w2856) -> (w2843:dbl[])
                        n1769 = Build Array(w2859) -> (w2838:dbl[])
                        n1770 = Build Array(w2869) -> (w2868:dbl[])
                        n1771 = Build Array(w2854) -> (w2833:dbl[])
                        n1772 = TDMS Write(0:w2875, 5:"LAB05-2 TEST VALUES", 7:w2870, 9:w2868) -> (4:w2863:refnum<k34>, 6:w2862:string, 15:w2850:errorcluster)  [unwired: 2 in, 1 out]
                        n1773 = TDMS Write(0:w2863, 5:w2862, 7:w2861, 9:w2855, 11:w2850) -> (4:w2853:refnum<k34>, 6:w2852:string, 15:w2851:errorcluster)  [unwired: 1 in, 1 out]
                        n1774 = TDMS Write(0:w2853, 5:w2852, 7:w2849, 9:w2848, 11:w2851) -> (4:w2847:refnum<k34>, 6:w2846:string, 15:w2845:errorcluster)  [unwired: 1 in, 1 out]
                        n1775 = TDMS Write(0:w2847, 5:w2846, 7:w2844, 9:w2843, 11:w2845) -> (4:w2842:refnum<k34>, 6:w2841:string, 15:w2840:errorcluster)  [unwired: 1 in, 1 out]
                        n1776 = TDMS Write(0:w2842, 5:w2841, 7:w2839, 9:w2838, 11:w2840) -> (4:w2837:refnum<k34>, 6:w2836:string, 15:w2835:errorcluster)  [unwired: 1 in, 1 out]
                        n1777 = TDMS Write(0:w2837, 5:w2836, 7:w2834, 9:w2833, 11:w2835) -> (15:w2832:errorcluster)  [unwired: 1 in, 3 out]
                        n1778 = local write "data file error"(w2832) -> ()
                      }
                    }
                  }
                }
              }
            }
          }
          frame #13 {
            # "check for amps fail"
            # "check for cycle test & temperature rise fail conditions"
            n1779 = local read "on loops"() -> (w2901:dbl)
            n1780 = local read "jig cycle"() -> (w2898:dbl)
            n1781 = local read "jig cycle"() -> (w2903:dbl)
            n1782 = Add(x=w2901, y=3.0) -> (x+y=w2899:dbl)
            n1783 = Equal?(x=w2898, y=w2899) -> (x = y?=w2894:bool)
            n1784 = Equal?(x=w2903, y=1.0) -> (x = y?=w2896:bool)
            n1785 = stacked-sequence {
              tunnel: w2897 -> [w2906 _ _ _ _ _ _ _ _ _]
              tunnel: w2896 -> [w2907 w2926 w2945 w2964 w2983 w3002 w3021 w3040 w3059 w3078]
              tunnel: w2895 -> [w2904 _ _ _ _ _ _ _ _ _]
              tunnel: w2894 -> [w2905 w2925 w2944 w2963 w2982 w3001 w3020 w3039 w3058 w3077]
              tunnel: w2893 -> [_ w2924 _ _ _ _ _ _ _ _]
              tunnel: w2892 -> [_ w2923 _ _ _ _ _ _ _ _]
              tunnel: w2891 -> [_ _ w2943 _ _ _ _ _ _ _]
              tunnel: w2890 -> [_ _ w2942 _ _ _ _ _ _ _]
              tunnel: w2889 -> [_ _ _ w2962 _ _ _ _ _ _]
              tunnel: w2888 -> [_ _ _ w2961 _ _ _ _ _ _]
              tunnel: w2887 -> [_ _ _ _ w2981 _ _ _ _ _]
              tunnel: w2886 -> [_ _ _ _ w2980 _ _ _ _ _]
              tunnel: w2885 -> [_ _ _ _ _ w3000 _ _ _ _]
              tunnel: w2884 -> [_ _ _ _ _ w2999 _ _ _ _]
              tunnel: w2883 -> [_ _ _ _ _ _ w3019 _ _ _]
              tunnel: w2882 -> [_ _ _ _ _ _ w3018 _ _ _]
              tunnel: w2881 -> [_ _ _ _ _ _ _ w3038 _ _]
              tunnel: w2880 -> [_ _ _ _ _ _ _ w3037 _ _]
              tunnel: w2879 -> [_ _ _ _ _ _ _ _ w3057 _]
              tunnel: w2878 -> [_ _ _ _ _ _ _ _ w3056 _]
              tunnel: w2877 -> [_ _ _ _ _ _ _ _ _ w3076]
              tunnel: w2876 -> [_ _ _ _ _ _ _ _ _ w3075]
              frame #0 {
                # "LAB01-1"
                n1786 = case shown="True" w2904 {
                  tunnel: w2907 -> [_ w2919]
                  tunnel: w2906 -> [_ w2916]
                  tunnel: w2905 -> [_ w2915]
                  frame False {
                  }
                  frame True {
                    n1787 = local read "LAB01-1 (TEMP START)"() -> (w2921:cluster{"TL":dbl, "TN":dbl})
                    n1788 = local read "LAB01-1 (RESULT)"() -> (w2908:bool)
                    n1789 = local read "LAB01-1 (FAIL)"() -> (w2912:cluster{"LO":dbl, "HI":dbl})
                    n1790 = local read "LAB01-1 (TDMS)"() -> (w2920:refnum<k34>)
                    n1791 = local read "LAB01-1 (SET)"() -> (w2917:T5)
                    n1792 = local read "LAB01-1 (DISP)"() -> (w2918:T4)
                    n1793 = local read "LAB01-1 (SIG)"() -> (w2922:T2)
                    n1794 = Bundle("LAB01-1 (FAIL)"=w2912, "LAB01-1 (SIG)"=w2922, "LAB01-1 (TEMP START)"=w2921, "LAB01-1 (DISP)"=w2918, "LAB01-1 (SET)"=w2917, "LAB01-1 (TDMS)"=w2920) -> (w2910:T23)  [unwired: 1 in]
                    n1795 = call "sub vi - cycle&temp fail v5.vi"("Amps Lo?"=w2919, "Input Cluster"=w2910, "SELECT"=w2916, "Amps Hi?"=w2915, "Result In"=w2908) -> ("(FAIL) out"=w2911:cluster{"FAIL LO":dbl, "FAIL HI":dbl}, "(DISP) out"=w2914:T4, "Result Out"=w2909:bool, "file error"=w2913:errorcluster)  [unwired: 11 in]
                    n1796 = local write "LAB01-1 (FAIL)"(w2911) -> ()
                    n1797 = local write "LAB01-1 (DISP)"(w2914) -> ()
                    n1798 = local write "LAB01-1 (RESULT)"(w2909) -> ()
                    n1799 = local write "data file error"(w2913) -> ()
                  }
                }
              }
              frame #1 {
                # "LAB01-2"
                n1800 = case shown="True" w2924 {
                  tunnel: w2926 -> [_ w2938]
                  tunnel: w2923 -> [_ w2935]
                  tunnel: w2925 -> [_ w2934]
                  frame False {
                  }
                  frame True {
                    n1801 = local read "LAB01-2 (TEMP START)"() -> (w2940:cluster{"TL":dbl, "TN":dbl})
                    n1802 = local read "LAB01-2 (FAIL)"() -> (w2931:cluster{"LO":dbl, "HI":dbl})
                    n1803 = local read "LAB01-2 (TDMS)"() -> (w2939:refnum<k34>)
                    n1804 = local read "LAB01-2 (SET)"() -> (w2936:T5)
                    n1805 = local read "LAB01-2 (DISP)"() -> (w2937:T4)
                    n1806 = local read "LAB01-2 (RESULT)"() -> (w2927:bool)
                    n1807 = local read "LAB01-2 (SIG)"() -> (w2941:T2)
                    n1808 = Bundle("LAB01-2 (FAIL)"=w2931, "LAB01-2 (SIG)"=w2941, "LAB01-2 (TEMP START)"=w2940, "LAB01-2 (DISP)"=w2937, "LAB01-2 (SET)"=w2936, "LAB01-2 (TDMS)"=w2939) -> (w2929:T24)  [unwired: 1 in]
                    n1809 = call "sub vi - cycle&temp fail v5.vi"("Amps Lo?"=w2938, "Input Cluster"=w2929, "SELECT"=w2935, "Amps Hi?"=w2934, "Result In"=w2927) -> ("(FAIL) out"=w2930:cluster{"FAIL LO":dbl, "FAIL HI":dbl}, "(DISP) out"=w2933:T4, "Result Out"=w2928:bool, "file error"=w2932:errorcluster)  [unwired: 11 in]
                    n1810 = local write "LAB01-2 (FAIL)"(w2930) -> ()
                    n1811 = local write "LAB01-2 (DISP)"(w2933) -> ()
                    n1812 = local write "LAB01-2 (RESULT)"(w2928) -> ()
                    n1813 = local write "data file error"(w2932) -> ()
                  }
                }
              }
              frame #2 {
                # "LAB02-1"
                n1814 = case shown="True" w2943 {
                  tunnel: w2945 -> [_ w2957]
                  tunnel: w2942 -> [_ w2954]
                  tunnel: w2944 -> [_ w2953]
                  frame False {
                  }
                  frame True {
                    n1815 = local read "LAB02-1 (TEMP START)"() -> (w2959:cluster{"TL":dbl, "TN":dbl})
                    n1816 = local read "LAB02-1 (FAIL)"() -> (w2950:cluster{"LO":dbl, "HI":dbl})
                    n1817 = local read "LAB02-1 (TDMS)"() -> (w2958:refnum<k34>)
                    n1818 = local read "LAB02-1 (SET)"() -> (w2955:T5)
                    n1819 = local read "LAB02-1 (DISP)"() -> (w2956:T4)
                    n1820 = local read "LAB02-1 (SIG)"() -> (w2960:T2)
                    n1821 = local read "LAB02-1 (RESULT)"() -> (w2946:bool)
                    n1822 = Bundle("LAB02-1 (FAIL)"=w2950, "LAB02-1 (SIG)"=w2960, "LAB02-1 (TEMP START)"=w2959, "LAB02-1 (DISP)"=w2956, "LAB02-1 (SET)"=w2955, "LAB02-1 (TDMS)"=w2958) -> (w2948:T25)  [unwired: 1 in]
                    n1823 = call "sub vi - cycle&temp fail v5.vi"("Amps Lo?"=w2957, "Input Cluster"=w2948, "SELECT"=w2954, "Amps Hi?"=w2953, "Result In"=w2946) -> ("(FAIL) out"=w2949:cluster{"FAIL LO":dbl, "FAIL HI":dbl}, "(DISP) out"=w2952:T4, "Result Out"=w2947:bool, "file error"=w2951:errorcluster)  [unwired: 11 in]
                    n1824 = local write "LAB02-1 (FAIL)"(w2949) -> ()
                    n1825 = local write "LAB02-1 (DISP)"(w2952) -> ()
                    n1826 = local write "LAB02-1 (RESULT)"(w2947) -> ()
                    n1827 = local write "data file error"(w2951) -> ()
                  }
                }
              }
              frame #3 {
                # "LAB02-2"
                n1828 = case shown="True" w2962 {
                  tunnel: w2964 -> [_ w2976]
                  tunnel: w2961 -> [_ w2973]
                  tunnel: w2963 -> [_ w2972]
                  frame False {
                  }
                  frame True {
                    n1829 = local read "LAB02-2 (TEMP START)"() -> (w2978:cluster{"TL":dbl, "TN":dbl})
                    n1830 = local read "LAB02-2 (FAIL)"() -> (w2969:cluster{"LO":dbl, "HI":dbl})
                    n1831 = local read "LAB02-2 (TDMS)"() -> (w2977:refnum<k34>)
                    n1832 = local read "LAB02-2 (SET)"() -> (w2974:T5)
                    n1833 = local read "LAB02-2 (DISP)"() -> (w2975:T4)
                    n1834 = local read "LAB02-2 (SIG)"() -> (w2979:T2)
                    n1835 = local read "LAB02-2 (RESULT)"() -> (w2965:bool)
                    n1836 = Bundle("LAB02-2 (FAIL)"=w2969, "LAB02-2 (SIG)"=w2979, "LAB02-2 (TEMP START)"=w2978, "LAB02-2 (DISP)"=w2975, "LAB02-2 (SET)"=w2974, "LAB02-2 (TDMS)"=w2977) -> (w2967:T26)  [unwired: 1 in]
                    n1837 = call "sub vi - cycle&temp fail v5.vi"("Amps Lo?"=w2976, "Input Cluster"=w2967, "SELECT"=w2973, "Amps Hi?"=w2972, "Result In"=w2965) -> ("(FAIL) out"=w2968:cluster{"FAIL LO":dbl, "FAIL HI":dbl}, "(DISP) out"=w2971:T4, "Result Out"=w2966:bool, "file error"=w2970:errorcluster)  [unwired: 11 in]
                    n1838 = local write "LAB02-2 (FAIL)"(w2968) -> ()
                    n1839 = local write "LAB02-2 (DISP)"(w2971) -> ()
                    n1840 = local write "LAB02-2 (RESULT)"(w2966) -> ()
                    n1841 = local write "data file error"(w2970) -> ()
                  }
                }
              }
              frame #4 {
                # "LAB03-1"
                n1842 = case shown="True" w2981 {
                  tunnel: w2983 -> [_ w2995]
                  tunnel: w2980 -> [_ w2992]
                  tunnel: w2982 -> [_ w2991]
                  frame False {
                  }
                  frame True {
                    n1843 = local read "LAB03-1 (TEMP START)"() -> (w2997:cluster{"TL":dbl, "TN":dbl})
                    n1844 = local read "LAB03-1 (FAIL)"() -> (w2988:cluster{"LO":dbl, "HI":dbl})
                    n1845 = local read "LAB03-1 (TDMS)"() -> (w2996:refnum<k34>)
                    n1846 = local read "LAB03-1 (SET)"() -> (w2993:T5)
                    n1847 = local read "LAB03-1 (DISP)"() -> (w2994:T4)
                    n1848 = local read "LAB03-1 (SIG)"() -> (w2998:T2)
                    n1849 = local read "LAB03-1 (RESULT)"() -> (w2984:bool)
                    n1850 = Bundle("LAB03-1 (FAIL)"=w2988, "LAB03-1 (SIG)"=w2998, "LAB03-1 (TEMP START)"=w2997, "LAB03-1 (DISP)"=w2994, "LAB03-1 (SET)"=w2993, "LAB03-1 (TDMS)"=w2996) -> (w2986:T27)  [unwired: 1 in]
                    n1851 = call "sub vi - cycle&temp fail v5.vi"("Amps Lo?"=w2995, "Input Cluster"=w2986, "SELECT"=w2992, "Amps Hi?"=w2991, "Result In"=w2984) -> ("(FAIL) out"=w2987:cluster{"FAIL LO":dbl, "FAIL HI":dbl}, "(DISP) out"=w2990:T4, "Result Out"=w2985:bool, "file error"=w2989:errorcluster)  [unwired: 11 in]
                    n1852 = local write "LAB03-1 (FAIL)"(w2987) -> ()
                    n1853 = local write "LAB03-1 (DISP)"(w2990) -> ()
                    n1854 = local write "LAB03-1 (RESULT)"(w2985) -> ()
                    n1855 = local write "data file error"(w2989) -> ()
                  }
                }
              }
              frame #5 {
                # "LAB03-2"
                n1856 = case shown="True" w3000 {
                  tunnel: w3002 -> [_ w3014]
                  tunnel: w2999 -> [_ w3011]
                  tunnel: w3001 -> [_ w3010]
                  frame False {
                  }
                  frame True {
                    n1857 = local read "LAB03-2 (TEMP START)"() -> (w3016:cluster{"TL":dbl, "TN":dbl})
                    n1858 = local read "LAB03-2 (FAIL)"() -> (w3007:cluster{"LO":dbl, "HI":dbl})
                    n1859 = local read "LAB03-2 (TDMS)"() -> (w3015:refnum<k34>)
                    n1860 = local read "LAB03-2 (SET)"() -> (w3012:T5)
                    n1861 = local read "LAB03-2 (DISP)"() -> (w3013:T4)
                    n1862 = local read "LAB03-2 (RESULT)"() -> (w3003:bool)
                    n1863 = local read "LAB03-2 (SIG)"() -> (w3017:T2)
                    n1864 = Bundle("LAB03-2 (FAIL)"=w3007, "LAB03-2 (SIG)"=w3017, "LAB03-2 (TEMP START)"=w3016, "LAB03-2 (DISP)"=w3013, "LAB03-2 (SET)"=w3012, "LAB03-2 (TDMS)"=w3015) -> (w3005:T28)  [unwired: 1 in]
                    n1865 = call "sub vi - cycle&temp fail v5.vi"("Amps Lo?"=w3014, "Input Cluster"=w3005, "SELECT"=w3011, "Amps Hi?"=w3010, "Result In"=w3003) -> ("(FAIL) out"=w3006:cluster{"FAIL LO":dbl, "FAIL HI":dbl}, "(DISP) out"=w3009:T4, "Result Out"=w3004:bool, "file error"=w3008:errorcluster)  [unwired: 11 in]
                    n1866 = local write "LAB03-2 (FAIL)"(w3006) -> ()
                    n1867 = local write "LAB03-2 (DISP)"(w3009) -> ()
                    n1868 = local write "LAB03-2 (RESULT)"(w3004) -> ()
                    n1869 = local write "data file error"(w3008) -> ()
                  }
                }
              }
              frame #6 {
                # "LAB04-1"
                n1870 = case shown="True" w3019 {
                  tunnel: w3021 -> [_ w3033]
                  tunnel: w3018 -> [_ w3030]
                  tunnel: w3020 -> [_ w3029]
                  frame False {
                  }
                  frame True {
                    n1871 = local read "LAB04-1 (TEMP START)"() -> (w3035:cluster{"TL":dbl, "TN":dbl})
                    n1872 = local read "LAB04-1 (FAIL)"() -> (w3026:cluster{"LO":dbl, "HI":dbl})
                    n1873 = local read "LAB04-1 (TDMS)"() -> (w3034:refnum<k34>)
                    n1874 = local read "LAB04-1 (SET)"() -> (w3031:T5)
                    n1875 = local read "LAB04-1 (DISP)"() -> (w3032:T4)
                    n1876 = local read "LAB04-1 (SIG)"() -> (w3036:T2)
                    n1877 = local read "LAB04-1 (RESULT)"() -> (w3022:bool)
                    n1878 = Bundle("LAB04-1 (FAIL)"=w3026, "LAB04-1 (SIG)"=w3036, "LAB04-1 (TEMP START)"=w3035, "LAB04-1 (DISP)"=w3032, "LAB04-1 (SET)"=w3031, "LAB04-1 (TDMS)"=w3034) -> (w3024:T29)  [unwired: 1 in]
                    n1879 = call "sub vi - cycle&temp fail v5.vi"("Amps Lo?"=w3033, "Input Cluster"=w3024, "SELECT"=w3030, "Amps Hi?"=w3029, "Result In"=w3022) -> ("(FAIL) out"=w3025:cluster{"FAIL LO":dbl, "FAIL HI":dbl}, "(DISP) out"=w3028:T4, "Result Out"=w3023:bool, "file error"=w3027:errorcluster)  [unwired: 11 in]
                    n1880 = local write "LAB04-1 (FAIL)"(w3025) -> ()
                    n1881 = local write "LAB04-1 (DISP)"(w3028) -> ()
                    n1882 = local write "LAB04-1 (RESULT)"(w3023) -> ()
                    n1883 = local write "data file error"(w3027) -> ()
                  }
                }
              }
              frame #7 {
                # "LAB04-2"
                n1884 = case shown="True" w3038 {
                  tunnel: w3040 -> [_ w3052]
                  tunnel: w3037 -> [_ w3049]
                  tunnel: w3039 -> [_ w3048]
                  frame False {
                  }
                  frame True {
                    n1885 = local read "LAB04-2 (TEMP START)"() -> (w3054:cluster{"TL":dbl, "TN":dbl})
                    n1886 = local read "LAB04-2 (FAIL)"() -> (w3045:cluster{"LO":dbl, "HI":dbl})
                    n1887 = local read "LAB04-2 (TDMS)"() -> (w3053:refnum<k34>)
                    n1888 = local read "LAB04-2 (SET)"() -> (w3050:T5)
                    n1889 = local read "LAB04-2 (DISP)"() -> (w3051:T4)
                    n1890 = local read "LAB04-2 (SIG)"() -> (w3055:T2)
                    n1891 = local read "LAB04-2 (RESULT)"() -> (w3041:bool)
                    n1892 = Bundle("LAB04-2 (FAIL)"=w3045, "LAB04-2 (SIG)"=w3055, "LAB04-2 (TEMP START)"=w3054, "LAB04-2 (DISP)"=w3051, "LAB04-2 (SET)"=w3050, "LAB04-2 (TDMS)"=w3053) -> (w3043:T30)  [unwired: 1 in]
                    n1893 = call "sub vi - cycle&temp fail v5.vi"("Amps Lo?"=w3052, "Input Cluster"=w3043, "SELECT"=w3049, "Amps Hi?"=w3048, "Result In"=w3041) -> ("(FAIL) out"=w3044:cluster{"FAIL LO":dbl, "FAIL HI":dbl}, "(DISP) out"=w3047:T4, "Result Out"=w3042:bool, "file error"=w3046:errorcluster)  [unwired: 11 in]
                    n1894 = local write "LAB04-2 (FAIL)"(w3044) -> ()
                    n1895 = local write "LAB04-2 (DISP)"(w3047) -> ()
                    n1896 = local write "LAB04-2 (RESULT)"(w3042) -> ()
                    n1897 = local write "data file error"(w3046) -> ()
                  }
                }
              }
              frame #8 {
                # "LAB05-1"
                n1898 = case shown="True" w3057 {
                  tunnel: w3059 -> [_ w3071]
                  tunnel: w3056 -> [_ w3068]
                  tunnel: w3058 -> [_ w3067]
                  frame False {
                  }
                  frame True {
                    n1899 = local read "LAB05-1 (TEMP START)"() -> (w3073:cluster{"TL":dbl, "TN":dbl})
                    n1900 = local read "LAB05-1 (FAIL)"() -> (w3064:cluster{"LO":dbl, "HI":dbl})
                    n1901 = local read "LAB05-1 (TDMS)"() -> (w3072:refnum<k34>)
                    n1902 = local read "LAB05-1 (SET)"() -> (w3069:T5)
                    n1903 = local read "LAB05-1 (DISP)"() -> (w3070:T4)
                    n1904 = local read "LAB05-1 (SIG)"() -> (w3074:T2)
                    n1905 = local read "LAB05-1 (RESULT)"() -> (w3060:bool)
                    n1906 = Bundle("LAB05-1 (FAIL)"=w3064, "LAB05-1 (SIG)"=w3074, "LAB05-1 (TEMP START)"=w3073, "LAB05-1 (DISP)"=w3070, "LAB05-1 (SET)"=w3069, "LAB05-1 (TDMS)"=w3072) -> (w3062:T31)  [unwired: 1 in]
                    n1907 = call "sub vi - cycle&temp fail v5.vi"("Amps Lo?"=w3071, "Input Cluster"=w3062, "SELECT"=w3068, "Amps Hi?"=w3067, "Result In"=w3060) -> ("(FAIL) out"=w3063:cluster{"FAIL LO":dbl, "FAIL HI":dbl}, "(DISP) out"=w3066:T4, "Result Out"=w3061:bool, "file error"=w3065:errorcluster)  [unwired: 11 in]
                    n1908 = local write "LAB05-1 (FAIL)"(w3063) -> ()
                    n1909 = local write "LAB05-1 (DISP)"(w3066) -> ()
                    n1910 = local write "LAB05-1 (RESULT)"(w3061) -> ()
                    n1911 = local write "data file error"(w3065) -> ()
                  }
                }
              }
              frame #9 {
                # "LAB05-2"
                n1912 = case shown="True" w3076 {
                  tunnel: w3078 -> [_ w3090]
                  tunnel: w3075 -> [_ w3087]
                  tunnel: w3077 -> [_ w3086]
                  frame False {
                  }
                  frame True {
                    n1913 = local read "LAB05-2 (TEMP START)"() -> (w3092:cluster{"TL":dbl, "TN":dbl})
                    n1914 = local read "LAB05-2 (FAIL)"() -> (w3083:cluster{"LO":dbl, "HI":dbl})
                    n1915 = local read "LAB05-2 (TDMS)"() -> (w3091:refnum<k34>)
                    n1916 = local read "LAB05-2 (SET)"() -> (w3088:T5)
                    n1917 = local read "LAB05-2 (DISP)"() -> (w3089:T4)
                    n1918 = local read "LAB05-2 (SIG)"() -> (w3093:T2)
                    n1919 = local read "LAB05-2 (RESULT)"() -> (w3079:bool)
                    n1920 = Bundle("LAB05-2 (FAIL)"=w3083, "LAB05-2 (SIG)"=w3093, "LAB05-2 (TEMP START)"=w3092, "LAB05-2 (DISP)"=w3089, "LAB05-2 (SET)"=w3088, "LAB05-2 (TDMS)"=w3091) -> (w3081:T32)  [unwired: 1 in]
                    n1921 = call "sub vi - cycle&temp fail v5.vi"("Amps Lo?"=w3090, "Input Cluster"=w3081, "SELECT"=w3087, "Amps Hi?"=w3086, "Result In"=w3079) -> ("(FAIL) out"=w3082:cluster{"FAIL LO":dbl, "FAIL HI":dbl}, "(DISP) out"=w3085:T4, "Result Out"=w3080:bool, "file error"=w3084:errorcluster)  [unwired: 11 in]
                    n1922 = local write "LAB05-2 (FAIL)"(w3082) -> ()
                    n1923 = local write "LAB05-2 (DISP)"(w3085) -> ()
                    n1924 = local write "LAB05-2 (RESULT)"(w3080) -> ()
                    n1925 = local write "data file error"(w3084) -> ()
                  }
                }
              }
            }
          }
          frame #14 {
            # "run calibration routine"
            n1926 = local read "CALIBRATE"() -> (w3094:bool)
            n1927 = case shown="True" w3094 {
              frame False {
              }
              frame True {
                n1928 = stacked-sequence {
                  seq-local: [w3095 _ _] -> [_ w3097 _]
                  frame #0 {
                    n1929 = call "CALIBRATION PASSWORD"() -> ("PASSWORD"=w3095:string)  [unwired: 17 in, 2 out]
                  }
                  frame #1 {
                    n1930 = Equal?(x=w3097, y="7777") -> (x = y?=w3096:bool)
                    n1931 = case shown="True" w3096 {
                      frame False {
                      }
                      frame True {
                        n1932 = stacked-sequence {
                          frame #0 {
                            n1933 = call "sub vi - calibration v1.vi"() -> ()  [unwired: 12 in]
                          }
                          frame #1 {
                            n1934 = call "sub vi - get calibration values v1.vi"() -> ("LAB01 (CAL)"=w3103:T6, "LAB02 (CAL)"=w3102:T7, "LAB03 (CAL)"=w3101:T6, "LAB04 (CAL)"=w3100:T6, "calibration file error out"=w3104:errorcluster, "LAB05 (CAL)"=w3099:T6)  [unwired: 10 in]
                            n1935 = local write "calibration file error out"(w3104) -> ()
                            n1936 = local write "LAB04 (CAL)"(w3100) -> ()
                            n1937 = local write "LAB05 (CAL)"(w3099) -> ()
                            n1938 = local write "LAB01 (CAL)"(w3103) -> ()
                            n1939 = local write "LAB02 (CAL)"(w3102) -> ()
                            n1940 = local write "LAB03 (CAL)"(w3101) -> ()
                          }
                        }
                      }
                    }
                  }
                  frame #2 {
                    n1941 = local write "CALIBRATE"(FALSE) -> ()
                  }
                }
              }
            }
          }
          frame #15 {
            # "save certain settings to file"
            n1942 = String To Path(string="c:\\crabtree\\Set Up\\") -> (path=w3108:path)
            n1943 = Build Path(base path=w3108, name or relative path="settings.bin") -> (appended path=w3106:path)
            n1944 = Create Folder(path (use dialog)=w3108) -> (error out=w3110:errorcluster)  [unwired: 2 in, 2 out]
            n1945 = call <vilib>:"Clear Errors.vi"("error in (no error)"=w3110) -> ()  [unwired: 6 in, 1 out]
            n1946 = stacked-sequence {
              seq-local: [w3111 _] -> [_ w3123]
              tunnel: w3106 -> [_ w3124]
              frame #0 {
                n1947 = local read "Network Directory"() -> (w3116:path)
                n1948 = local read "LAB05-2 (SET)"() -> (w3115:T5)
                n1949 = local read "LAB05-1 (SET)"() -> (w3114:T5)
                n1950 = local read "LAB04-2 (SET)"() -> (w3113:T5)
                n1951 = local read "LAB03-2 (SET)"() -> (w3117:T5)
                n1952 = local read "LAB04-1 (SET)"() -> (w3112:T5)
                n1953 = local read "LAB03-1 (SET)"() -> (w3118:T5)
                n1954 = local read "LAB02-2 (SET)"() -> (w3119:T5)
                n1955 = local read "LAB02-1 (SET)"() -> (w3120:T5)
                n1956 = local read "LAB01-2 (SET)"() -> (w3121:T5)
                n1957 = local read "LAB01-1 (SET)"() -> (w3122:T5)
                n1958 = Bundle("LAB01-1 (SET)"=w3122, "LAB01-2 (SET)"=w3121, "LAB02-1 (SET)"=w3120, "LAB02-2 (SET)"=w3119, "LAB03-1 (SET)"=w3118, "LAB03-2 (SET)"=w3117, "LAB04-1 (SET)"=w3112, "LAB04-2 (SET)"=w3113, "LAB05-1 (SET)"=w3114, "LAB05-2 (SET)"=w3115, "Network Directory"=w3116) -> (w3111:T16)  [unwired: 1 in]
              }
              frame #1 {
                n1959 = event shown="[1] \"LAB01-1 (SET)\", \"LAB01-2 (SET)\", \"LAB02-1 (SET)\", \"LAB02-2 (SET)\", \"LAB03-1 (SET)\", \"LAB03-2 (SET)\", \"LAB04-1 (SET)\", \"LAB04-2 (SET)\", \"LAB05-1 (SET)\", \"LAB05-2 (SET)\", \"Network Directory\": Value Change" {
                  selector: _ -> [_ _]
                  dyn-events: _ -> [_ _]
                  timeout: 10.0 -> [_ _]
                  tunnel: w3124 -> [_ w3126]
                  tunnel: w3123 -> [_ w3127]
                  event Timeout {
                    n1960 = event-data() -> ()  [unwired: 1 in, 3 out]
                  }
                  event "LAB01-1 (SET)", "LAB01-2 (SET)", "LAB02-1 (SET)", "LAB02-2 (SET)", "LAB03-1 (SET)", "LAB03-2 (SET)", "LAB04-1 (SET)", "LAB04-2 (SET)", "LAB05-1 (SET)", "LAB05-2 (SET)", "Network Directory": Value Change {
                    n1961 = event-data() -> ()  [unwired: 1 in, 6 out]
                    n1962 = Open/Create/Replace File(file path (use dialog)=w3126, operation (0:open)=T15."replace or create") -> (refnum out=w3132:refnum<file>, error out=w3131:errorcluster)  [unwired: 4 in, 1 out]
                    n1963 = Write to Binary File(file (use dialog)=w3132, data=w3127, error in=w3131) -> (refnum out=w3130:refnum<file>, error out=w3129:errorcluster)  [unwired: 3 in, 1 out]
                    n1964 = Close File(refnum=w3130, error in=w3129) -> (error out=w3128:errorcluster)  [unwired: 1 out]
                    n1965 = local write "data file error"(w3128) -> ()
                  }
                }
              }
            }
          }
        }
        n1966 = node-c288() -> ()  [unwired: 1 in, 1 out]
        "loops" <- w70
      }
      n1967 = node-c288(w47) -> ()  [unwired: 1 out]
    }
  }
